vi "manual vs automated tracked data (real world coordinates).vi"() -> ()   [LabVIEW 2013]
panel:
  out "x/y 2":dbl
  out "x/y":dbl
  out "Waveform Graph 2":sgl[][](graph)
  out "Waveform Graph":sgl[][](graph)
  out "Y":sgl[](array[numeric])
  out "X":sgl[](array[numeric])
  out "Y 2":dbl[](array[numeric])
  out "X 2":dbl[](array[numeric])
  in  "auto top FangYang vs Ueda":T1[](array[typedef])=[{"X"=-379.219, "Y"=-1944.1919}, {"X"=240.74095, "Y"=358.58084}, {"X"=236.91107, "Y"=378.82852}, {"X"=238.72923, "Y"=457.2503}, {"X"=246.48058, "Y"=461.8201}, {"X"=265.79745, "Y"=446.8123}, {"X"=271.0491, "Y"=407.61075}, {"X"=277.55893, "Y"=412.3402}, {"X"=288.31927, "Y"=362.18567}, {"X"=298.93817, "Y"=356.80734}, {"X"=303.91098, "Y"=386.79193}, {"X"=329.3833, "Y"=355.87955}, {"X"=354.7859, "Y"=344.95035}, {"X"=363.8193, "Y"=354.83017}, {"X"=363.8193, "Y"=354.83017}, {"X"=414.12973, "Y"=388.4446}, {"X"=421.80878, "Y"=393.18253}, {"X"=440.06366, "Y"=451.29065}, {"X"=455.7114, "Y"=498.36505}, {"X"=464.16785, "Y"=553.61487}, {"X"=472.8004, "Y"=511.89783}, {"X"=458.46417, "Y"=469.90585}, {"X"=458.46417, "Y"=469.90585}, {"X"=447.3518, "Y"=460.67822}, {"X"=444.36072, "Y"=387.53275}, {"X"=437.37646, "Y"=367.7333}, {"X"=415.4438, "Y"=388.40497}, {"X"=397.8395, "Y"=403.80304}, {"X"=389.98856, "Y"=404.03882}, {"X"=361.21103, "Y"=404.90305}, {"X"=363.9455, "Y"=298.30313}, {"X"=396.3589, "Y"=408.77762}, {"X"=400.2796, "Y"=408.66003}, {"X"=419.1897, "Y"=189.43721}, {"X"=436.9622, "Y"=161.15974}, {"X"=445.31467, "Y"=160.89108}, {"X"=461.96823, "Y"=103.768394}, {"X"=460.7954, "Y"=69.094284}, {"X"=468.21814, "Y"=33.54667}, {"X"=467.0633, "Y"=57.186203}, {"X"=470.7626, "Y"=68.76565}, {"X"=470.15222, "Y"=109.23079}, {"X"=464.2563, "Y"=171.41397}, {"X"=456.3204, "Y"=221.01631}, {"X"=445.86578, "Y"=269.50647}, {"X"=438.85596, "Y"=275.0047}, {"X"=424.95166, "Y"=317.16812}, {"X"=423.05118, "Y"=363.13348}, {"X"=412.08105, "Y"=373.52164}, {"X"=396.9989, "Y"=500.07834}, {"X"=382.2929, "Y"=560.511}, {"X"=371.58298, "Y"=583.38385}, {"X"=350.8116, "Y"=458.73624}, {"X"=346.625, "Y"=473.19745}, {"X"=347.8018, "Y"=477.91788}, {"X"=349.33124, "Y"=410.1879}, {"X"=345.52036, "Y"=405.37427}, {"X"=346.936, "Y"=400.39108}, {"X"=340.89392, "Y"=375.6783}, {"X"=333.8183, "Y"=330.26135}, {"X"=326.2376, "Y"=304.67575}, {"X"=323.5547, "Y"=304.75873}, {"X"=322.37048, "Y"=294.37253}, {"X"=313.15634, "Y"=278.9214}, {"X"=295.73862, "Y"=263.60336}, {"X"=294.3835, "Y"=263.64578}, {"X"=297.13943, "Y"=258.24423}, {"X"=278.10477, "Y"=269.45547}, {"X"=241.50314, "Y"=254.66132}, {"X"=216.58736, "Y"=328.72873}, {"X"=210.20592, "Y"=349.36923}, {"X"=204.47275, "Y"=228.98254}, {"X"=197.85901, "Y"=324.16034}, {"X"=200.60747, "Y"=329.22}, {"X"=205.63214, "Y"=308.4058}, {"X"=215.69052, "Y"=364.3957}, {"X"=226.2489, "Y"=364.0744}, {"X"=218.27173, "Y"=359.26556}, {"X"=227.4764, "Y"=353.91983}, {"X"=237.96664, "Y"=338.3229}, {"X"=243.2823, "Y"=338.15997}, {"X"=225.9597, "Y"=333.5725}, {"X"=225.41745, "Y"=276.38568}, {"X"=232.00192, "Y"=254.9596}, {"X"=220.97665, "Y"=239.24193}, {"X"=207.9769, "Y"=185.16287}, {"X"=213.36469, "Y"=173.9132}, {"X"=189.40637, "Y"=72.21436}, {"X"=181.8577, "Y"=48.98817}, {"X"=183.73094, "Y"=72.40179}, {"X"=195.36647, "Y"=89.45416}, {"X"=199.78233, "Y"=100.85296}, {"X"=211.69986, "Y"=151.62987}, {"X"=221.6728, "Y"=173.64636}, {"X"=232.91647, "Y"=195.38316}, {"X"=238.62537, "Y"=227.90225}, {"X"=246.82507, "Y"=227.64288}, {"X"=259.14227, "Y"=243.40915}, {"X"=260.52017, "Y"=270.00504}, {"X"=257.81534, "Y"=270.08957}, {"X"=242.96771, "Y"=275.838}, {"X"=250.69382, "Y"=150.36983}, {"X"=255.08963, "Y"=259.56235}, {"X"=261.86682, "Y"=248.67987}, {"X"=272.69354, "Y"=269.6246}, {"X"=278.10477, "Y"=269.45547}, {"X"=282.1635, "Y"=269.32864}, {"X"=286.2226, "Y"=269.20178}, {"X"=272.70654, "Y"=264.32425}, {"X"=306.6389, "Y"=257.94647}, {"X"=303.5981, "Y"=289.72357}, {"X"=347.25598, "Y"=261.9909}, {"X"=294.258, "Y"=279.51022}, {"X"=364.34863, "Y"=282.58826}, {"X"=356.25198, "Y"=282.84018}, {"X"=356.25198, "Y"=282.84018}, {"X"=309.64783, "Y"=346.32993}, {"X"=304.28574, "Y"=351.5757}, {"X"=304.6125, "Y"=320.87338}, {"X"=304.3941, "Y"=341.39526}, {"X"=300.4082, "Y"=341.51727}, {"X"=303.11807, "Y"=336.32578}, {"X"=301.73682, "Y"=341.4766}, {"X"=293.36713, "Y"=392.0872}, {"X"=265.8795, "Y"=337.4673}, {"X"=229.95079, "Y"=333.44998}, {"X"=224.6294, "Y"=333.61334}, {"X"=221.08926, "Y"=249.96196}, {"X"=206.20949, "Y"=157.41422}, {"X"=199.17181, "Y"=152.03471}, {"X"=177.59418, "Y"=118.7725}, {"X"=162.02908, "Y"=55.53973}, {"X"=181.57751, "Y"=107.19645}, {"X"=187.20538, "Y"=107.01233}, {"X"=210.45204, "Y"=162.8691}, {"X"=229.01479, "Y"=222.7933}, {"X"=241.6175, "Y"=275.88016}, {"X"=265.98276, "Y"=199.81622}, {"X"=281.8607, "Y"=331.85638}, {"X"=309.83194, "Y"=330.9977}, {"X"=353.24872, "Y"=410.0704}, {"X"=369.1337, "Y"=448.57358}, {"X"=354.31934, "Y"=419.85693}, {"X"=388.86124, "Y"=476.71115}, {"X"=404.44525, "Y"=471.49573}, {"X"=397.5853, "Y"=447.73016}, {"X"=335.15945, "Y"=468.76834}, {"X"=399.13074, "Y"=476.40933}, {"X"=409.58768, "Y"=471.34436}, {"X"=442.19287, "Y"=460.83047}, {"X"=428.71732, "Y"=531.71704}, {"X"=435.66354, "Y"=545.30023}, {"X"=441.3716, "Y"=531.35144}, {"X"=441.08243, "Y"=563.3649}, {"X"=441.82288, "Y"=599.25073}, {"X"=441.82288, "Y"=599.25073}, {"X"=300.9056, "Y"=289.80722}, {"X"=303.27682, "Y"=320.91452}, {"X"=304.88873, "Y"=294.91483}, {"X"=302.14774, "Y"=300.21722}, {"X"=311.16425, "Y"=330.9568}, {"X"=325.41125, "Y"=356.0006}, {"X"=336.2913, "Y"=340.41895}, {"X"=345.92438, "Y"=324.75232}, {"X"=359.84485, "Y"=354.9513}, {"X"=373.0323, "Y"=261.1841}, {"X"=376.3531, "Y"=239.7184}, {"X"=397.72824, "Y"=212.01292}, {"X"=403.9889, "Y"=189.92242}, {"X"=421.00232, "Y"=178.3422}, {"X"=435.3338, "Y"=166.7844}, {"X"=443.82617, "Y"=194.148}, {"X"=405.97333, "Y"=211.75133}, {"X"=395.51877, "Y"=195.68765}, {"X"=382.29224, "Y"=223.35791}, {"X"=365.83505, "Y"=277.27997}, {"X"=359.91315, "Y"=298.428}, {"X"=351.9673, "Y"=293.45447}, {"X"=359.40192, "Y"=319.1864}, {"X"=374.11057, "Y"=318.73352}, {"X"=406.23087, "Y"=353.53772}, {"X"=431.4278, "Y"=352.76987}, {"X"=433.6227, "Y"=392.8267}, {"X"=457.67108, "Y"=460.37363}, {"X"=451.4063, "Y"=507.85492}, {"X"=448.51663, "Y"=489.16385}, {"X"=448.51663, "Y"=489.16385}, {"X"=425.93756, "Y"=508.59604}, {"X"=418.19464, "Y"=480.59506}, {"X"=391.5912, "Y"=471.87402}, {"X"=392.87646, "Y"=471.8362}, {"X"=374.60245, "Y"=481.8744}, {"X"=358.30508, "Y"=468.08615}, {"X"=332.6767, "Y"=464.06296}, {"X"=310.7989, "Y"=464.7087}, {"X"=300.5541, "Y"=460.22177}, {"X"=268.79126, "Y"=160.98972}, {"X"=301.7822, "Y"=198.67523}, {"X"=274.39758, "Y"=143.9781}, {"X"=243.649, "Y"=133.67818}, {"X"=223.9627, "Y"=122.96163}, {"X"=206.67265, "Y"=89.082535}, {"X"=209.72241, "Y"=106.27566}, {"X"=213.87715, "Y"=100.39111}, {"X"=224.33687, "Y"=162.4218}, {"X"=244.06622, "Y"=222.31648}, {"X"=246.91164, "Y"=249.15009}, {"X"=248.3299, "Y"=265.08722}, {"X"=240.20668, "Y"=265.34146}, {"X"=222.39363, "Y"=244.5663}, {"X"=217.94925, "Y"=212.27502}, {"X"=216.70294, "Y"=223.18333}, {"X"=220.28804, "Y"=173.69084}, {"X"=208.69188, "Y"=134.81302}, {"X"=206.98508, "Y"=112.09752}, {"X"=199.60603, "Y"=89.31481}, {"X"=199.33972, "Y"=71.88633}, {"X"=200.75891, "Y"=71.83946}, {"X"=199.5175, "Y"=83.52155}, {"X"=197.51016, "Y"=135.17603}, {"X"=206.36482, "Y"=168.57701}, {"X"=205.60648, "Y"=212.66722}, {"X"=200.03648, "Y"=207.38855}, {"X"=192.34073, "Y"=314.00165}, {"X"=187.25673, "Y"=395.2878}, {"X"=175.81679, "Y"=410.47076}, {"X"=170.72452, "Y"=468.84314}, {"X"=160.84576, "Y"=483.4124}, {"X"=164.80504, "Y"=488.03143}, {"X"=126.20091, "Y"=549.63324}, {"X"=122.39982, "Y"=581.50006}, {"X"=113.91068, "Y"=617.37}, {"X"=111.26169, "Y"=613.0294}, {"X"=309.1677, "Y"=273.77222}, {"X"=309.5259, "Y"=356.48468}, {"X"=317.46802, "Y"=356.24268}, {"X"=314.82053, "Y"=356.32333}, {"X"=302.96057, "Y"=351.61618}, {"X"=302.96057, "Y"=351.61618}, {"X"=296.3351, "Y"=351.81836}, {"X"=263.21674, "Y"=392.9966}, {"X"=242.17143, "Y"=378.66916}, {"X"=246.204, "Y"=398.4716}, {"X"=228.1136, "Y"=423.63065}, {"X"=201.92369, "Y"=491.66708}, {"X"=293.8873, "Y"=326.35217}, {"X"=200.47363, "Y"=556.62933}, {"X"=222.29388, "Y"=486.34427}, {"X"=233.27432, "Y"=418.57858}, {"X"=250.01248, "Y"=363.3513}, {"X"=264.5458, "Y"=347.7084}, {"X"=267.19788, "Y"=347.62735}, {"X"=289.39935, "Y"=397.1706}, {"X"=297.43478, "Y"=376.99493}, {"X"=312.10898, "Y"=361.46176}, {"X"=332.48547, "Y"=330.30225}, {"X"=346.03375, "Y"=319.59802}, {"X"=346.5849, "Y"=293.62143}, {"X"=371.967, "Y"=250.56561}, {"X"=379.76813, "Y"=308.2136}, {"X"=402.4357, "Y"=348.58032}, {"X"=411.69434, "Y"=383.5361}, {"X"=419.88736, "Y"=408.07205}, {"X"=429.587, "Y"=238.04216}, {"X"=426.85587, "Y"=238.12817}, {"X"=414.32574, "Y"=383.4566}, {"X"=407.9354, "Y"=378.65494}, {"X"=399.2458, "Y"=363.85678}, {"X"=392.97385, "Y"=353.9417}, {"X"=385.34088, "Y"=344.01648}, {"X"=376.34485, "Y"=287.46362}, {"X"=374.99683, "Y"=287.5055}, {"X"=367.3255, "Y"=271.95737}, {"X"=366.10992, "Y"=266.7051}, {"X"=344.87204, "Y"=246.07013}, {"X"=328.3579, "Y"=257.26566}, {"X"=300.6056, "Y"=320.99677}, {"X"=273.95816, "Y"=301.09036}, {"X"=261.89386, "Y"=347.78946}, {"X"=229.19672, "Y"=398.98386}, {"X"=222.28929, "Y"=364.1949}, {"X"=221.96889, "Y"=333.695}, {"X"=217.18909, "Y"=379.426}, {"X"=224.97849, "Y"=369.1518}, {"X"=236.80927, "Y"=363.75305}, {"X"=257.9162, "Y"=347.91104}, {"X"=281.96057, "Y"=311.23404}, {"X"=295.3917, "Y"=305.62973}, {"X"=304.94443, "Y"=289.68173}, {"X"=306.34842, "Y"=284.3928}, {"X"=340.3712, "Y"=267.5095}, {"X"=347.3689, "Y"=256.66974}, {"X"=357.3827, "Y"=234.94028}, {"X"=360.42987, "Y"=277.4484}, {"X"=369.24594, "Y"=250.65103}, {"X"=385.66235, "Y"=333.79547}, {"X"=417.4444, "Y"=337.93494}, {"X"=413.45056, "Y"=338.0572}, {"X"=428.72202, "Y"=291.07355}, {"X"=409.45697, "Y"=338.17944}, {"X"=394.12802, "Y"=358.966}, {"X"=386.3465, "Y"=354.14368}, {"X"=376.3368, "Y"=334.08133}, {"X"=359.14832, "Y"=329.48373}, {"X"=339.45166, "Y"=314.63647}, {"X"=323.71545, "Y"=294.3308}, {"X"=310.393, "Y"=284.26697}, {"X"=300.9056, "Y"=289.80722}, {"X"=287.60858, "Y"=263.85782}, {"X"=287.64157, "Y"=258.54196}, {"X"=264.582, "Y"=259.2648}, {"X"=252.32089, "Y"=238.25346}, {"X"=234.67851, "Y"=249.5347}, {"X"=218.60973, "Y"=271.31485}, {"X"=176.73038, "Y"=272.62366}, {"X"=169.85439, "Y"=267.54343}, {"X"=161.87743, "Y"=273.08786}, {"X"=305.05627, "Y"=279.17377}, {"X"=303.54422, "Y"=294.95654}, {"X"=313.22327, "Y"=273.64566}, {"X"=320.11566, "Y"=356.162}, {"X"=337.2312, "Y"=360.69733}, {"X"=358.14706, "Y"=370.13712}, {"X"=349.7784, "Y"=390.38565}, {"X"=326.65207, "Y"=361.01923}, {"X"=293.64502, "Y"=356.96863}, {"X"=303.9795, "Y"=252.69997}, {"X"=271.46576, "Y"=210.57452}, {"X"=257.67438, "Y"=161.34784}, {"X"=228.31302, "Y"=139.8306}, {"X"=206.67265, "Y"=89.082535}, {"X"=200.93274, "Y"=83.47496}, {"X"=215.8117, "Y"=145.87416}, {"X"=205.89624, "Y"=134.90378}, {"X"=217.51859, "Y"=173.77979}, {"X"=223.00299, "Y"=168.04184}, {"X"=224.54747, "Y"=184.63231}, {"X"=235.85585, "Y"=222.57658}, {"X"=241.50314, "Y"=254.66132}, {"X"=248.5037, "Y"=312.26724}, {"X"=244.4902, "Y"=312.39117}, {"X"=240.3876, "Y"=296.91562}, {"X"=240.2975, "Y"=281.1916}, {"X"=235.01584, "Y"=297.08224}, {"X"=202.55582, "Y"=282.36755}, {"X"=176.81717, "Y"=213.58202}, {"X"=188.58812, "Y"=256.3225}, {"X"=180.3701, "Y"=186.04678}, {"X"=180.96799, "Y"=147.00183}, {"X"=177.71228, "Y"=124.46775}, {"X"=164.87761, "Y"=55.445217}, {"X"=160.02571, "Y"=31.936}, {"X"=169.54489, "Y"=72.87026}, {"X"=178.41144, "Y"=90.01146}, {"X"=194.80911, "Y"=140.91658}, {"X"=209.06375, "Y"=162.91382}, {"X"=218.84299, "Y"=168.17564}, {"X"=228.83044, "Y"=201.00035}, {"X"=239.9919, "Y"=227.85902}, {"X"=255.0473, "Y"=238.1675}, {"X"=261.87262, "Y"=269.96277}, {"X"=260.51038, "Y"=254.06462}, {"X"=270.03537, "Y"=243.06615}, {"X"=283.65466, "Y"=242.6373}, {"X"=295.8706, "Y"=247.61078}, {"X"=305.56696, "Y"=231.18684}, {"X"=310.6467, "Y"=263.13675}, {"X"=372.19714, "Y"=339.31992}, {"X"=410.2086, "Y"=353.4165}, {"X"=403.69467, "Y"=457.1731}, {"X"=407.02423, "Y"=504.47195}, {"X"=409.40213, "Y"=476.10745}, {"X"=406.8435, "Y"=509.1516}, {"X"=405.7687, "Y"=536.985}, {"X"=404.5055, "Y"=537.0214}, {"X"=398.35855, "Y"=532.59424}, {"X"=398.52753, "Y"=527.9733}, {"X"=395.66397, "Y"=537.2765}, {"X"=381.03802, "Y"=560.54694}, {"X"=347.79678, "Y"=534.0551}, {"X"=323.13248, "Y"=497.53937}, {"X"=293.8394, "Y"=493.69034}, {"X"=265.7652, "Y"=489.79614}, {"X"=250.43665, "Y"=490.24536}, {"X"=245.33957, "Y"=200.47417}, {"X"=118.084724, "Y"=-153.04642}, {"X"=187.93501, "Y"=146.77635}, {"X"=173.50957, "Y"=124.60461}, {"X"=200.81985, "Y"=168.75537}, {"X"=189.63121, "Y"=163.53984}, {"X"=199.95107, "Y"=201.92079}, {"X"=207.12892, "Y"=223.48662}, {"X"=216.70294, "Y"=223.18333}, {"X"=251.02194, "Y"=259.68985}, {"X"=271.15475, "Y"=357.654}, {"X"=286.8732, "Y"=382.31723}, {"X"=290.31995, "Y"=450.90988}, {"X"=285.35538, "Y"=417.019}, {"X"=299.80493, "Y"=535.4418}, {"X"=303.0285, "Y"=469.71536}, {"X"=304.6303, "Y"=440.82095}, {"X"=316.1484, "Y"=450.14423}, {"X"=321.84073, "Y"=415.92648}, {"X"=300.60196, "Y"=455.41882}, {"X"=307.33325, "Y"=431.02618}, {"X"=310.17142, "Y"=411.3622}, {"X"=320.8349, "Y"=396.2238}, {"X"=332.21237, "Y"=345.6403}, {"X"=330.8784, "Y"=420.55783}, {"X"=347.69815, "Y"=424.94507}, {"X"=341.93652, "Y"=256.84}, {"X"=348.63104, "Y"=197.18207}, {"X"=367.4061, "Y"=163.39705}, {"X"=393.15042, "Y"=140.13481}, {"X"=399.95477, "Y"=145.54662}, {"X"=432.32553, "Y"=104.73669}, {"X"=438.21426, "Y"=98.800285}, {"X"=422.44806, "Y"=105.05933}, {"X"=399.95477, "Y"=145.54662}, {"X"=382.86548, "Y"=157.31483}, {"X"=374.20538, "Y"=168.7476}, {"X"=364.89804, "Y"=207.60568}, {"X"=356.017, "Y"=234.98335}, {"X"=357.12906, "Y"=245.68477}, {"X"=362.17767, "Y"=261.52386}, {"X"=376.34485, "Y"=287.46362}, {"X"=403.31186, "Y"=286.62585}, {"X"=404.66055, "Y"=286.58395}, {"X"=412.35614, "Y"=296.80368}, {"X"=416.63788, "Y"=358.28104}, {"X"=404.53503, "Y"=363.69608}, {"X"=396.80368, "Y"=433.2259}, {"X"=390.8023, "Y"=418.76605}, {"X"=388.01697, "Y"=384.25134}, {"X"=382.05923, "Y"=364.379}, {"X"=368.62222, "Y"=324.05447}, {"X"=360.86798, "Y"=313.97607}, {"X"=358.56912, "Y"=298.46964}, {"X"=348.38382, "Y"=272.54846}, {"X"=344.7622, "Y"=251.41966}, {"X"=359.9835, "Y"=240.23386}, {"X"=376.65897, "Y"=228.94151}, {"X"=373.6245, "Y"=239.80432}, {"X"=357.3197, "Y"=118.61896}, {"X"=362.44385, "Y"=250.86458}, {"X"=360.821, "Y"=261.5663}, {"X"=354.0381, "Y"=261.77863}, {"X"=341.50626, "Y"=345.35623}, {"X"=332.03146, "Y"=355.79886}, {"X"=331.9691, "Y"=283.59567}, {"X"=322.37048, "Y"=294.37253}, {"X"=323.87708, "Y"=283.84744}, {"X"=328.74655, "Y"=314.96658}, {"X"=322.0569, "Y"=315.17285}, {"X"=332.76074, "Y"=314.8428}, {"X"=371.3333, "Y"=223.70456}, {"X"=385.69534, "Y"=201.48022}, {"X"=411.3019, "Y"=178.65279}, {"X"=439.07886, "Y"=144.28235}, {"X"=451.1975, "Y"=92.61483}, {"X"=466.7766, "Y"=63.05458}, {"X"=475.5642, "Y"=86.03841}, {"X"=479.00424, "Y"=74.32069}, {"X"=467.62756, "Y"=74.69521}, {"X"=461.96823, "Y"=103.768394}, {"X"=431.8558, "Y"=116.19174}, {"X"=397.63095, "Y"=173.55046}, {"X"=363.11554, "Y"=223.9645}, {"X"=331.4402, "Y"=235.75839}, {"X"=302.19974, "Y"=294.99823}, {"X"=274.0315, "Y"=274.86865}, {"X"=245.69124, "Y"=281.0235}, {"X"=236.21696, "Y"=276.04868}, {"X"=201.98804, "Y"=245.20883}, {"X"=206.22096, "Y"=255.76895}, {"X"=204.9421, "Y"=261.13428}, {"X"=208.01904, "Y"=287.45206}, {"X"=221.96889, "Y"=333.695}, {"X"=237.56705, "Y"=276.00656}, {"X"=263.223, "Y"=301.42285}, {"X"=291.29462, "Y"=316.12143}, {"X"=328.65985, "Y"=320.13297}, {"X"=362.49445, "Y"=354.87054}, {"X"=384.2289, "Y"=379.37207}, {"X"=367.65726, "Y"=359.77148}, {"X"=401.1082, "Y"=348.62085}, {"X"=396.25394, "Y"=374.00113}, {"X"=386.38184, "Y"=394.24954}, {"X"=367.3848, "Y"=369.85684}, {"X"=345.38187, "Y"=350.32153}, {"X"=328.83347, "Y"=309.78653}, {"X"=317.97086, "Y"=320.46207}, {"X"=303.5981, "Y"=289.72357}, {"X"=286.44205, "Y"=231.79086}, {"X"=274.16602, "Y"=226.77806}, {"X"=253.64651, "Y"=222.01299}, {"X"=238.62537, "Y"=227.90225}, {"X"=221.08926, "Y"=249.96196}, {"X"=210.29085, "Y"=255.64119}, {"X"=193.92058, "Y"=250.81616}, {"X"=191.3005, "Y"=256.23737}, {"X"=155.12737, "Y"=273.2988}, {"X"=164.96967, "Y"=288.7914}, {"X"=203.26804, "Y"=239.80038}, {"X"=212.1883, "Y"=190.54393}, {"X"=198.34164, "Y"=271.94827}, {"X"=208.23715, "Y"=303.12598}, {"X"=208.23715, "Y"=303.12598}, {"X"=298.88113, "Y"=215.14905}, {"X"=301.15927, "Y"=263.4337}, {"X"=303.70636, "Y"=279.21582}, {"X"=304.1243, "Y"=366.747}, {"X"=315.16135, "Y"=330.8341}, {"X"=328.00946, "Y"=278.45856}, {"X"=327.75055, "Y"=294.20566}, {"X"=327.2389, "Y"=325.32678}, {"X"=334.5714, "Y"=288.76135}, {"X"=340.2679, "Y"=272.8017}, {"X"=351.0894, "Y"=272.46402}, {"X"=352.08554, "Y"=288.21725}, {"X"=386.3465, "Y"=354.14368}, {"X"=414.32574, "Y"=383.4566}, {"X"=426.63568, "Y"=402.93823}, {"X"=418.67697, "Y"=373.3218}, {"X"=414.65796, "Y"=408.22885}, {"X"=395.2224, "Y"=403.88162}, {"X"=392.6054, "Y"=403.96024}, {"X"=367.88538, "Y"=399.76102}, {"X"=365.2663, "Y"=399.83978}, {"X"=357.40973, "Y"=400.07608}, {"X"=356.1004, "Y"=400.11545}, {"X"=349.08444, "Y"=477.8802}, {"X"=341.68768, "Y"=463.797}, {"X"=353.73636, "Y"=444.2017}, {"X"=365.51648, "Y"=439.01086}, {"X"=380.17352, "Y"=467.44162}, {"X"=386.32892, "Y"=514.4104}, {"X"=457.86722, "Y"=431.4079}, {"X"=484.4065, "Y"=-57.935837}, {"X"=442.9617, "Y"=417.20642}, {"X"=412.45734, "Y"=527.5703}, {"X"=397.76608, "Y"=514.0781}, {"X"=382.66696, "Y"=509.8551}, {"X"=375.16956, "Y"=462.80875}, {"X"=367.88538, "Y"=399.76102}, {"X"=332.62775, "Y"=395.8686}, {"X"=323.45532, "Y"=396.14487}, {"X"=302.5465, "Y"=391.8103}, {"X"=296.03244, "Y"=387.0299}, {"X"=286.81134, "Y"=392.28494}, {"X"=286.81134, "Y"=392.28494}, {"X"=400.17252, "Y"=447.65347}, {"X"=399.2077, "Y"=509.3738}, {"X"=403.02548, "Y"=509.26273}, {"X"=405.19016, "Y"=485.7102}, {"X"=403.02548, "Y"=509.26273}, {"X"=396.90216, "Y"=466.94855}, {"X"=394.44757, "Y"=500.1528}, {"X"=391.42844, "Y"=476.6357}, {"X"=386.60703, "Y"=467.25198}, {"X"=386.60703, "Y"=467.25198}, {"X"=375.7407, "Y"=528.6326}, {"X"=377.27362, "Y"=560.65485}, {"X"=391.75436, "Y"=467.10028}, {"X"=359.71393, "Y"=463.26492}, {"X"=335.34302, "Y"=459.19345}, {"X"=335.34302, "Y"=459.19345}, {"X"=361.00174, "Y"=463.22693}, {"X"=363.57742, "Y"=463.1509}, {"X"=406.55682, "Y"=195.33585}, {"X"=418.8694, "Y"=161.7417}, {"X"=427.36685, "Y"=87.62015}, {"X"=427.5587, "Y"=46.72962}, {"X"=432.80966, "Y"=22.828001}, {"X"=433.52322, "Y"=40.624928}, {"X"=429.9314, "Y"=22.924105}, {"X"=423.71936, "Y"=35.027763}, {"X"=402.69833, "Y"=105.70447}, {"X"=400.40546, "Y"=173.46149}, {"X"=397.3642, "Y"=222.88116}, {"X"=399.36795, "Y"=244.35674}, {"X"=419.91556, "Y"=275.59488}, {"X"=422.62094, "Y"=275.51056}, {"X"=421.35406, "Y"=306.92935}, {"X"=418.98203, "Y"=398.22427}, {"X"=390.63828, "Y"=423.66296}, {"X"=395.90833, "Y"=384.01294}, {"X"=380.73743, "Y"=364.41916}, {"X"=362.3646, "Y"=359.93253}, {"X"=337.32822, "Y"=355.63745}, {"X"=333.35562, "Y"=355.7585}, {"X"=330.70737, "Y"=355.8392}, {"X"=326.73523, "Y"=355.96027}, {"X"=301.38425, "Y"=376.87527}, {"X"=301.6354, "Y"=351.65662}, {"X"=298.9852, "Y"=351.7375}, {"X"=298.9852, "Y"=351.7375}, {"X"=328.31293, "Y"=175.77328}, {"X"=342.16974, "Y"=175.32893}, {"X"=363.3731, "Y"=157.94276}, {"X"=380.4029, "Y"=146.1784}, {"X"=412.9895, "Y"=93.8668}, {"X"=427.05325, "Y"=23.020203}, {"X"=445.9059, "Y"=52.011703}, {"X"=430.90436, "Y"=70.07986}, {"X"=436.11108, "Y"=81.54107}, {"X"=436.11108, "Y"=81.54107}, {"X"=442.61676, "Y"=127.21894}, {"X"=444.85556, "Y"=232.18176}, {"X"=447.96188, "Y"=253.51651}, {"X"=446.4858, "Y"=285.2846}, {"X"=441.34085, "Y"=367.613}, {"X"=451.66818, "Y"=372.32233}, {"X"=455.37817, "Y"=377.21973}, {"X"=457.47787, "Y"=488.9016}, {"X"=450.0969, "Y"=558.5684}, {"X"=438.5471, "Y"=456.1429}, {"X"=428.2476, "Y"=485.0345}, {"X"=432.30676, "Y"=451.52026}, {"X"=422.70807, "Y"=403.05618}, {"X"=417.07404, "Y"=413.07477}, {"X"=395.90833, "Y"=384.01294}, {"X"=386.5079, "Y"=349.06644}, {"X"=377.971, "Y"=323.76706}, {"X"=369.04123, "Y"=308.54486}, {"X"=360.0418, "Y"=293.20398}, {"X"=349.27603, "Y"=293.53793}, {"X"=348.38382, "Y"=272.54846}, {"X"=343.2946, "Y"=256.79742}, {"X"=342.97308, "Y"=272.7173}, {"X"=328.83347, "Y"=309.78653}, {"X"=320.41577, "Y"=335.79553}, {"X"=314.82053, "Y"=356.32333}, {"X"=309.70905, "Y"=341.23257}, {"X"=310.0175, "Y"=315.5441}, {"X"=313.6956, "Y"=341.11057}, {"X"=316.14426, "Y"=356.28302}, {"X"=330.2622, "Y"=304.55127}, {"X"=328.65985, "Y"=320.13297}, {"X"=333.35562, "Y"=355.7585}, {"X"=330.70737, "Y"=355.8392}, {"X"=384.21347, "Y"=250.18115}, {"X"=349.07306, "Y"=240.57741}, {"X"=350.31927, "Y"=245.89886}, {"X"=324.5323, "Y"=241.35014}, {"X"=373.77353, "Y"=234.42339}, {"X"=373.77353, "Y"=234.42339}] {"Y" format="%.2f"; "X" format="%.2f"}
  in  "manual top FangYang vs Ueda":T1[](array[typedef])=[{"X"=239.20204, "Y"=322.8874}, {"X"=235.19978, "Y"=323.01062}, {"X"=230.03725, "Y"=343.67123}, {"X"=239.44966, "Y"=363.67273}, {"X"=246.204, "Y"=398.4716}, {"X"=251.4529, "Y"=403.26276}, {"X"=261.89664, "Y"=357.93613}, {"X"=275.09128, "Y"=367.62915}, {"X"=280.4372, "Y"=352.30356}, {"X"=284.5524, "Y"=326.63916}, {"X"=312.7584, "Y"=310.28296}, {"X"=342.86652, "Y"=277.99564}, {"X"=370.953, "Y"=287.6311}, {"X"=382.5318, "Y"=260.88678}, {"X"=387.81464, "Y"=307.9651}, {"X"=402.80164, "Y"=338.38315}, {"X"=417.96228, "Y"=358.24075}, {"X"=442.4209, "Y"=456.0284}, {"X"=454.60397, "Y"=470.01947}, {"X"=450.98236, "Y"=465.3546}, {"X"=449.82892, "Y"=436.50436}, {"X"=437.07224, "Y"=432.027}, {"X"=433.61102, "Y"=422.37988}, {"X"=428.82626, "Y"=412.72284}, {"X"=416.55896, "Y"=393.34064}, {"X"=399.2458, "Y"=363.85678}, {"X"=396.14706, "Y"=338.58682}, {"X"=374.11057, "Y"=318.73352}, {"X"=370.52417, "Y"=303.3061}, {"X"=378.4604, "Y"=261.01422}, {"X"=392.2322, "Y"=212.1873}, {"X"=400.9716, "Y"=156.73154}, {"X"=415.1122, "Y"=150.6741}, {"X"=431.14822, "Y"=99.03146}, {"X"=444.27118, "Y"=121.48421}, {"X"=457.94797, "Y"=69.18817}, {"X"=467.07086, "Y"=27.642868}, {"X"=467.9282, "Y"=39.481594}, {"X"=488.00742, "Y"=38.81433}, {"X"=489.5957, "Y"=62.30101}, {"X"=481.6519, "Y"=50.827534}, {"X"=474.2033, "Y"=56.950043}, {"X"=455.6411, "Y"=57.563995}, {"X"=445.17215, "Y"=132.80139}, {"X"=435.54196, "Y"=194.41203}, {"X"=435.25616, "Y"=264.54413}, {"X"=411.2074, "Y"=291.61685}, {"X"=379.46008, "Y"=318.56882}, {"X"=371.91138, "Y"=349.5119}, {"X"=379.82373, "Y"=394.44708}, {"X"=360.58163, "Y"=429.43857}, {"X"=362.39056, "Y"=409.79626}, {"X"=356.46255, "Y"=385.2045}, {"X"=351.82843, "Y"=415.0285}, {"X"=360.91373, "Y"=365.02148}, {"X"=361.556, "Y"=339.64563}, {"X"=348.1457, "Y"=345.1533}, {"X"=348.3694, "Y"=334.93866}, {"X"=332.94547, "Y"=304.4683}, {"X"=325.39175, "Y"=273.26593}, {"X"=318.63116, "Y"=273.4769}, {"X"=316.13992, "Y"=257.64865}, {"X"=318.92975, "Y"=252.23064}, {"X"=320.21228, "Y"=257.521}, {"X"=309.47787, "Y"=247.18295}, {"X"=304.03458, "Y"=247.3541}, {"X"=289.0682, "Y"=247.82465}, {"X"=257.80157, "Y"=259.47733}, {"X"=234.82944, "Y"=270.80792}, {"X"=224.47781, "Y"=318.1818}, {"X"=209.71854, "Y"=313.465}, {"X"=206.67325, "Y"=287.49393}, {"X"=208.45354, "Y"=318.6759}, {"X"=203.03413, "Y"=313.67142}, {"X"=210.84918, "Y"=297.8319}, {"X"=214.74847, "Y"=287.24268}, {"X"=217.44046, "Y"=287.15894}, {"X"=228.02405, "Y"=265.72278}, {"X"=246.95456, "Y"=259.81735}, {"X"=251.10126, "Y"=286.11166}, {"X"=249.71925, "Y"=275.62732}, {"X"=253.69653, "Y"=243.58063}, {"X"=246.89008, "Y"=243.79495}, {"X"=226.02925, "Y"=195.60301}, {"X"=211.69986, "Y"=151.62987}, {"X"=205.33966, "Y"=94.906654}, {"X"=199.16093, "Y"=60.185703}, {"X"=201.83557, "Y"=48.324272}, {"X"=189.90411, "Y"=18.999298}, {"X"=189.80031, "Y"=13.007771}, {"X"=198.98116, "Y"=48.41913}, {"X"=202.43257, "Y"=89.22191}, {"X"=215.41914, "Y"=111.822014}, {"X"=228.45569, "Y"=156.69646}, {"X"=235.5224, "Y"=173.20157}, {"X"=246.5597, "Y"=161.7059}, {"X"=254.97212, "Y"=200.16716}, {"X"=265.9705, "Y"=216.1932}, {"X"=268.66595, "Y"=248.46611}, {"X"=270.03537, "Y"=243.06615}, {"X"=261.8712, "Y"=264.6634}, {"X"=260.51364, "Y"=259.3923}, {"X"=261.86972, "Y"=259.3498}, {"X"=270.03537, "Y"=243.06615}, {"X"=279.56854, "Y"=242.76596}, {"X"=276.88205, "Y"=232.0928}, {"X"=276.8446, "Y"=242.85175}, {"X"=280.88235, "Y"=253.42508}, {"X"=288.9635, "Y"=263.8154}, {"X"=284.98718, "Y"=247.95296}, {"X"=298.54404, "Y"=252.8706}, {"X"=300.00217, "Y"=242.12256}, {"X"=322.84717, "Y"=262.75488}, {"X"=351.20712, "Y"=267.17087}, {"X"=374.55194, "Y"=303.18152}, {"X"=324.97818, "Y"=299.51007}, {"X"=312.7584, "Y"=310.28296}, {"X"=304.88873, "Y"=294.91483}, {"X"=307.57788, "Y"=294.8314}, {"X"=298.2132, "Y"=289.89084}, {"X"=286.2537, "Y"=263.90024}, {"X"=271.3745, "Y"=253.72356}, {"X"=283.40732, "Y"=290.3508}, {"X"=274.00204, "Y"=285.39917}, {"X"=276.77036, "Y"=264.19705}, {"X"=267.31775, "Y"=237.78053}, {"X"=232.75221, "Y"=173.29054}, {"X"=215.74673, "Y"=140.23792}, {"X"=197.05548, "Y"=106.69007}, {"X"=181.12276, "Y"=84.12712}, {"X"=173.80034, "Y"=72.72973}, {"X"=174.84859, "Y"=55.114388}, {"X"=185.04059, "Y"=66.51422}, {"X"=198.10231, "Y"=83.56814}, {"X"=225.36484, "Y"=122.91598}, {"X"=229.80086, "Y"=151.04497}, {"X"=240.02283, "Y"=233.25694}, {"X"=249.63046, "Y"=249.06459}, {"X"=278.0243, "Y"=290.51804}, {"X"=322.52853, "Y"=283.8894}, {"X"=353.22137, "Y"=355.15314}, {"X"=369.3323, "Y"=394.76306}, {"X"=385.43167, "Y"=423.81842}, {"X"=396.97522, "Y"=428.35352}, {"X"=394.32822, "Y"=467.0244}, {"X"=385.78766, "Y"=452.89725}, {"X"=389.82434, "Y"=447.96024}, {"X"=394.2067, "Y"=433.3032}, {"X"=401.2898, "Y"=452.4384}, {"X"=424.5509, "Y"=451.74982}, {"X"=437.4779, "Y"=451.3672}, {"X"=441.6659, "Y"=498.77493}, {"X"=453.95383, "Y"=507.7808}, {"X"=454.57773, "Y"=544.75604}, {"X"=450.42508, "Y"=576.64655}, {"X"=292.8288, "Y"=290.05814}, {"X"=291.4072, "Y"=300.5499}, {"X"=288.85962, "Y"=279.67844}, {"X"=291.5207, "Y"=284.85413}, {"X"=295.56424, "Y"=284.7283}, {"X"=303.8152, "Y"=268.65198}, {"X"=324.44962, "Y"=246.71223}, {"X"=341.51572, "Y"=278.03772}, {"X"=348.15652, "Y"=283.09204}, {"X"=361.47995, "Y"=234.81107}, {"X"=364.62234, "Y"=218.49739}, {"X"=382.7011, "Y"=162.90508}, {"X"=401.60315, "Y"=178.96332}, {"X"=428.12524, "Y"=139.0029}, {"X"=432.79208, "Y"=127.53789}, {"X"=439.80954, "Y"=127.310074}, {"X"=432.55756, "Y"=133.21027}, {"X"=411.13034, "Y"=145.18549}, {"X"=398.37158, "Y"=151.21423}, {"X"=381.7242, "Y"=196.12732}, {"X"=342.25513, "Y"=240.79208}, {"X"=350.20212, "Y"=251.24889}, {"X"=340.3712, "Y"=267.5095}, {"X"=355.14798, "Y"=272.33737}, {"X"=377.54062, "Y"=292.6612}, {"X"=399.16617, "Y"=328.25522}, {"X"=423.46967, "Y"=353.0124}, {"X"=440.5809, "Y"=412.37085}, {"X"=441.19894, "Y"=427.03497}, {"X"=445.46802, "Y"=446.31076}, {"X"=447.5864, "Y"=455.87573}, {"X"=434.03534, "Y"=441.81793}, {"X"=434.91373, "Y"=422.34097}, {"X"=419.28314, "Y"=422.80768}, {"X"=394.42258, "Y"=389.03903}, {"X"=376.1881, "Y"=339.19775}, {"X"=366.87634, "Y"=339.48276}, {"X"=370.5846, "Y"=349.55237}, {"X"=368.25726, "Y"=287.71487}, {"X"=349.3053, "Y"=229.80544}, {"X"=337.20065, "Y"=219.36607}, {"X"=326.92743, "Y"=175.81772}, {"X"=299.57486, "Y"=137.52074}, {"X"=278.825, "Y"=80.910706}, {"X"=232.07677, "Y"=82.449684}, {"X"=220.80858, "Y"=88.6179}, {"X"=210.84033, "Y"=83.148796}, {"X"=216.3724, "Y"=71.323845}, {"X"=223.691, "Y"=94.3044}, {"X"=238.08875, "Y"=139.51372}, {"X"=245.09705, "Y"=144.92638}, {"X"=248.09155, "Y"=200.38646}, {"X"=250.89282, "Y"=216.67159}, {"X"=248.15187, "Y"=216.75854}, {"X"=246.71555, "Y"=200.43031}, {"X"=229.80086, "Y"=151.04497}, {"X"=218.539, "Y"=140.1474}, {"X"=205.57951, "Y"=112.143425}, {"X"=216.50261, "Y"=82.962395}, {"X"=206.2772, "Y"=59.949963}, {"X"=194.01985, "Y"=6.85391}, {"X"=198.98116, "Y"=48.41913}, {"X"=201.92157, "Y"=54.21612}, {"X"=206.19743, "Y"=54.07425}, {"X"=223.691, "Y"=94.3044}, {"X"=225.52028, "Y"=139.92111}, {"X"=214.6833, "Y"=168.30945}, {"X"=210.73833, "Y"=185.07445}, {"X"=202.47536, "Y"=277.1016}, {"X"=176.7875, "Y"=395.60358}, {"X"=172.86205, "Y"=395.722}, {"X"=164.08694, "Y"=410.82303}, {"X"=134.96031, "Y"=474.66898}, {"X"=131.66402, "Y"=526.44995}, {"X"=119.037506, "Y"=494.09613}, {"X"=113.462845, "Y"=545.4187}, {"X"=109.466774, "Y"=599.76953}, {"X"=317.13464, "Y"=284.05722}, {"X"=322.29178, "Y"=299.5933}, {"X"=322.37048, "Y"=294.37253}, {"X"=307.8159, "Y"=273.8144}, {"X"=313.15634, "Y"=278.9214}, {"X"=300.9056, "Y"=289.80722}, {"X"=269.90463, "Y"=316.781}, {"X"=269.95078, "Y"=290.76886}, {"X"=263.223, "Y"=301.42285}, {"X"=231.1978, "Y"=323.13382}, {"X"=205.3592, "Y"=379.7844}, {"X"=200.09319, "Y"=458.39398}, {"X"=194.00696, "Y"=477.68924}, {"X"=190.3484, "Y"=487.2818}, {"X"=205.5351, "Y"=477.34998}, {"X"=206.74506, "Y"=472.5532}, {"X"=219.51836, "Y"=467.40295}, {"X"=239.72214, "Y"=408.55157}, {"X"=260.58963, "Y"=383.11234}, {"X"=298.93817, "Y"=356.80734}, {"X"=306.0049, "Y"=315.66782}, {"X"=316.6349, "Y"=320.5032}, {"X"=322.21326, "Y"=304.8002}, {"X"=342.97308, "Y"=272.7173}, {"X"=365.97232, "Y"=271.9996}, {"X"=377.872, "Y"=234.29413}, {"X"=381.81067, "Y"=239.54655}, {"X"=394.5717, "Y"=265.8156}, {"X"=409.87863, "Y"=254.71028}, {"X"=415.78433, "Y"=312.28268}, {"X"=410.98233, "Y"=333.01932}, {"X"=417.4444, "Y"=337.93494}, {"X"=413.45056, "Y"=338.0572}, {"X"=411.53455, "Y"=353.3761}, {"X"=410.4243, "Y"=312.44797}, {"X"=397.0264, "Y"=312.8611}, {"X"=386.1092, "Y"=276.64825}, {"X"=371.38525, "Y"=271.8307}, {"X"=375.89737, "Y"=255.77547}, {"X"=379.8175, "Y"=260.97174}, {"X"=366.66412, "Y"=245.38498}, {"X"=363.25095, "Y"=218.54083}, {"X"=357.12906, "Y"=245.68477}, {"X"=327.3451, "Y"=235.88753}, {"X"=282.4234, "Y"=215.6712}, {"X"=247.03975, "Y"=280.9815}, {"X"=227.1017, "Y"=312.92816}, {"X"=208.88121, "Y"=349.40973}, {"X"=200.52539, "Y"=324.07825}, {"X"=207.33832, "Y"=334.14417}, {"X"=214.3075, "Y"=359.38635}, {"X"=227.29002, "Y"=333.53168}, {"X"=245.828, "Y"=312.34988}, {"X"=274.00204, "Y"=285.39917}, {"X"=290.20917, "Y"=279.63638}, {"X"=303.8152, "Y"=268.65198}, {"X"=312.06784, "Y"=257.77628}, {"X"=324.44962, "Y"=246.71223}, {"X"=353.2857, "Y"=235.06947}, {"X"=357.51, "Y"=229.54631}, {"X"=354.528, "Y"=240.40564}, {"X"=355.76703, "Y"=245.72758}, {"X"=377.25623, "Y"=255.73286}, {"X"=393.7403, "Y"=249.88208}, {"X"=408.32034, "Y"=296.92868}, {"X"=409.66556, "Y"=296.88702}, {"X"=411.568, "Y"=317.5802}, {"X"=410.2298, "Y"=317.6214}, {"X"=393.00766, "Y"=312.98502}, {"X"=389.4904, "Y"=297.5119}, {"X"=384.11157, "Y"=297.6785}, {"X"=350.62164, "Y"=293.4962}, {"X"=325.22568, "Y"=283.80548}, {"X"=310.77457, "Y"=252.48665}, {"X"=313.3577, "Y"=263.05188}, {"X"=297.27725, "Y"=242.20836}, {"X"=290.5397, "Y"=231.66145}, {"X"=283.6269, "Y"=247.99573}, {"X"=267.2944, "Y"=259.17975}, {"X"=248.21169, "Y"=232.9983}, {"X"=219.37984, "Y"=217.6714}, {"X"=192.27815, "Y"=234.76488}, {"X"=176.03485, "Y"=240.6592}, {"X"=143.37236, "Y"=241.68924}, {"X"=290.13678, "Y"=290.14175}, {"X"=298.0269, "Y"=310.73788}, {"X"=292.90836, "Y"=279.55228}, {"X"=302.4617, "Y"=268.69427}, {"X"=321.10266, "Y"=289.17978}, {"X"=346.9191, "Y"=277.86935}, {"X"=360.1708, "Y"=287.96606}, {"X"=351.84933, "Y"=298.6778}, {"X"=359.33545, "Y"=266.91684}, {"X"=335.63342, "Y"=230.23724}, {"X"=295.11438, "Y"=171.2877}, {"X"=266.02444, "Y"=144.24908}, {"X"=243.46063, "Y"=93.6556}, {"X"=222.16544, "Y"=82.77597}, {"X"=205.0978, "Y"=77.52516}, {"X"=207.6228, "Y"=54.02696}, {"X"=210.84033, "Y"=83.148796}, {"X"=220.86732, "Y"=94.39707}, {"X"=226.91663, "Y"=139.87585}, {"X"=233.97882, "Y"=150.90996}, {"X"=238.29272, "Y"=173.1126}, {"X"=242.56001, "Y"=195.07533}, {"X"=245.41104, "Y"=216.8455}, {"X"=256.43686, "Y"=254.1925}, {"X"=252.36363, "Y"=254.32037}, {"X"=249.68388, "Y"=265.04483}, {"X"=248.34941, "Y"=270.3854}, {"X"=209.72043, "Y"=212.5365}, {"X"=189.15364, "Y"=213.19002}, {"X"=181.41675, "Y"=169.37947}, {"X"=182.36133, "Y"=146.95674}, {"X"=178.17488, "Y"=78.412865}, {"X"=175.34163, "Y"=78.50628}, {"X"=173.17143, "Y"=43.36698}, {"X"=171.87143, "Y"=49.32003}, {"X"=171.61406, "Y"=37.492336}, {"X"=177.4572, "Y"=43.224335}, {"X"=185.04059, "Y"=66.51422}, {"X"=201.01929, "Y"=89.26836}, {"X"=215.55072, "Y"=123.235565}, {"X"=227.0157, "Y"=151.13496}, {"X"=236.90755, "Y"=173.15709}, {"X"=239.74142, "Y"=184.14583}, {"X"=255.03665, "Y"=232.78275}, {"X"=264.59296, "Y"=232.48093}, {"X"=274.13583, "Y"=237.56552}, {"X"=283.68253, "Y"=237.26447}, {"X"=285.13602, "Y"=221.01544}, {"X"=301.67697, "Y"=209.61456}, {"X"=308.4837, "Y"=214.84439}, {"X"=311.293, "Y"=209.309}, {"X"=430.9709, "Y"=301.4366}, {"X"=421.2309, "Y"=342.91956}, {"X"=413.9342, "Y"=393.4197}, {"X"=414.0739, "Y"=422.9632}, {"X"=397.41385, "Y"=452.5531}, {"X"=399.4008, "Y"=433.14856}, {"X"=409.2406, "Y"=413.30933}, {"X"=409.42905, "Y"=408.38565}, {"X"=408.4969, "Y"=398.5396}, {"X"=382.75665, "Y"=384.41022}, {"X"=377.49686, "Y"=384.56912}, {"X"=367.24908, "Y"=374.87985}, {"X"=351.61435, "Y"=309.083}, {"X"=346.8074, "Y"=283.134}, {"X"=324.20294, "Y"=262.71243}, {"X"=287.9426, "Y"=210.05096}, {"X"=263.23178, "Y"=172.31165}, {"X"=245.07243, "Y"=139.28735}, {"X"=210.08975, "Y"=134.76764}, {"X"=179.82416, "Y"=89.96503}, {"X"=180.40004, "Y"=118.680984}, {"X"=181.80301, "Y"=118.63523}, {"X"=195.92763, "Y"=123.87458}, {"X"=206.51932, "Y"=179.67885}, {"X"=227.59892, "Y"=217.41063}, {"X"=238.59251, "Y"=222.48988}, {"X"=255.07909, "Y"=254.23512}, {"X"=280.73935, "Y"=285.18954}, {"X"=287.18747, "Y"=331.69287}, {"X"=293.5253, "Y"=372.09772}, {"X"=296.03244, "Y"=387.0299}, {"X"=296.3351, "Y"=351.81836}, {"X"=294.39368, "Y"=426.53662}, {"X"=296.03244, "Y"=387.0299}, {"X"=289.6755, "Y"=357.0896}, {"X"=301.4843, "Y"=366.8272}, {"X"=295.05206, "Y"=346.77603}, {"X"=298.89124, "Y"=361.86395}, {"X"=301.8899, "Y"=326.10614}, {"X"=320.49127, "Y"=330.67047}, {"X"=318.1892, "Y"=304.92468}, {"X"=322.92737, "Y"=257.43588}, {"X"=323.2503, "Y"=236.01666}, {"X"=337.10043, "Y"=224.78738}, {"X"=354.7634, "Y"=107.27028}, {"X"=375.59305, "Y"=118.0239}, {"X"=402.89285, "Y"=99.95587}, {"X"=412.9895, "Y"=93.8668}, {"X"=421.69928, "Y"=87.80615}, {"X"=424.7589, "Y"=81.91421}, {"X"=421.8352, "Y"=46.91952}, {"X"=396.20218, "Y"=88.642914}, {"X"=386.28976, "Y"=88.96822}, {"X"=368.71072, "Y"=112.539276}, {"X"=361.44037, "Y"=180.24925}, {"X"=352.16034, "Y"=224.31102}, {"X"=358.7484, "Y"=234.8972}, {"X"=374.8383, "Y"=245.12798}, {"X"=380.28842, "Y"=244.95662}, {"X"=396.92502, "Y"=276.31122}, {"X"=409.2776, "Y"=307.30228}, {"X"=408.50772, "Y"=327.96844}, {"X"=406.23087, "Y"=353.53772}, {"X"=406.4046, "Y"=312.57193}, {"X"=404.53503, "Y"=363.69608}, {"X"=395.9726, "Y"=343.69153}, {"X"=385.82373, "Y"=328.66483}, {"X"=372.3009, "Y"=287.58923}, {"X"=361.7811, "Y"=277.40628}, {"X"=354.528, "Y"=240.40564}, {"X"=356.50092, "Y"=272.29514}, {"X"=346.45807, "Y"=235.28479}, {"X"=343.72726, "Y"=235.37091}, {"X"=350.67267, "Y"=229.76225}, {"X"=352.04007, "Y"=229.71906}, {"X"=359.26718, "Y"=213.23318}, {"X"=367.50662, "Y"=212.97177}, {"X"=365.7159, "Y"=229.28714}, {"X"=361.2153, "Y"=245.55629}, {"X"=358.49112, "Y"=245.64194}, {"X"=347.7094, "Y"=240.62035}, {"X"=327.0002, "Y"=257.3082}, {"X"=315.20224, "Y"=225.48004}, {"X"=315.9979, "Y"=268.27124}, {"X"=314.71323, "Y"=263.00946}, {"X"=321.5698, "Y"=257.47842}, {"X"=336.9008, "Y"=235.58618}, {"X"=353.38123, "Y"=169.4164}, {"X"=391.5746, "Y"=145.81741}, {"X"=407.33127, "Y"=94.0522}, {"X"=424.81992, "Y"=116.42086}, {"X"=444.6267, "Y"=81.26116}, {"X"=467.62756, "Y"=74.69521}, {"X"=475.63144, "Y"=56.90281}, {"X"=482.15582, "Y"=68.38999}, {"X"=482.89117, "Y"=27.115475}, {"X"=468.4912, "Y"=57.138973}, {"X"=439.19592, "Y"=75.6312}, {"X"=427.1376, "Y"=93.403206}, {"X"=397.71783, "Y"=128.67653}, {"X"=347.94574, "Y"=164.023}, {"X"=340.57178, "Y"=186.43959}, {"X"=279.6133, "Y"=232.00655}, {"X"=264.60855, "Y"=194.37154}, {"X"=248.17186, "Y"=222.18642}, {"X"=222.17453, "Y"=223.01}, {"X"=204.47275, "Y"=228.98254}, {"X"=198.83734, "Y"=218.32315}, {"X"=205.76134, "Y"=223.52995}, {"X"=218.43153, "Y"=255.38562}, {"X"=232.12582, "Y"=270.89243}, {"X"=234.86691, "Y"=276.09082}, {"X"=251.03789, "Y"=265.00244}, {"X"=292.90836, "Y"=279.55228}, {"X"=337.26553, "Y"=288.67764}, {"X"=370.09872, "Y"=318.85706}, {"X"=378.27472, "Y"=313.43933}, {"X"=397.3017, "Y"=343.6509}, {"X"=401.1082, "Y"=348.62085}, {"X"=395.1631, "Y"=328.3781}, {"X"=385.66235, "Y"=333.79547}, {"X"=351.49734, "Y"=314.26505}, {"X"=328.92065, "Y"=304.59277}, {"X"=324.03958, "Y"=273.30814}, {"X"=310.77457, "Y"=252.48665}, {"X"=300.25284, "Y"=215.10553}, {"X"=285.2869, "Y"=193.71147}, {"X"=285.13602, "Y"=221.01544}, {"X"=261.85052, "Y"=188.95625}, {"X"=254.97212, "Y"=200.16716}, {"X"=227.40663, "Y"=195.55904}, {"X"=200.03648, "Y"=207.38855}, {"X"=183.99109, "Y"=229.6304}, {"X"=158.19951, "Y"=235.84119}, {"X"=154.54918, "Y"=252.05402}, {"X"=166.50633, "Y"=240.95969}, {"X"=169.10243, "Y"=235.49684}, {"X"=187.02863, "Y"=245.67987}, {"X"=198.92392, "Y"=223.74655}, {"X"=207.65163, "Y"=261.04935}, {"X"=288.5866, "Y"=321.36682}, {"X"=292.59265, "Y"=321.24347}, {"X"=288.62042, "Y"=316.2039}, {"X"=296.64337, "Y"=315.9565}, {"X"=298.26007, "Y"=284.64444}, {"X"=317.4244, "Y"=262.9246}, {"X"=327.83664, "Y"=288.97058}, {"X"=333.59976, "Y"=267.72113}, {"X"=330.89142, "Y"=267.80576}, {"X"=337.76242, "Y"=262.28806}, {"X"=352.92227, "Y"=251.1635}, {"X"=363.66913, "Y"=256.15878}, {"X"=379.66135, "Y"=266.2816}, {"X"=396.92502, "Y"=276.31122}, {"X"=412.90622, "Y"=317.539}, {"X"=422.56058, "Y"=342.8789}, {"X"=421.2309, "Y"=342.91956}, {"X"=417.85086, "Y"=327.6816}, {"X"=391.98547, "Y"=343.8134}, {"X"=382.52667, "Y"=349.18793}, {"X"=366.49667, "Y"=303.43063}, {"X"=346.69598, "Y"=288.38467}, {"X"=320.9486, "Y"=299.6349}, {"X"=325.14294, "Y"=289.05426}, {"X"=315.43726, "Y"=310.20023}, {"X"=308.8009, "Y"=305.21503}, {"X"=325.5748, "Y"=345.84314}, {"X"=345.94833, "Y"=385.5221}, {"X"=368.51352, "Y"=424.32355}, {"X"=396.73245, "Y"=471.72272}, {"X"=389.18063, "Y"=467.17615}, {"X"=399.8947, "Y"=490.58673}, {"X"=399.30328, "Y"=471.64706}, {"X"=386.13828, "Y"=481.53583}, {"X"=394.2067, "Y"=433.3032}, {"X"=384.65097, "Y"=448.1136}, {"X"=370.2898, "Y"=453.35602}, {"X"=354.43683, "Y"=414.9504}, {"X"=347.59152, "Y"=370.45737}, {"X"=327.07013, "Y"=335.59155}, {"X"=317.5393, "Y"=351.17123}, {"X"=304.66745, "Y"=315.70908}, {"X"=287.12396, "Y"=341.9239}, {"X"=414.0452, "Y"=322.65796}, {"X"=417.55872, "Y"=368.33456}, {"X"=415.57202, "Y"=418.0254}, {"X"=409.6027, "Y"=437.70023}, {"X"=400.52332, "Y"=437.97015}, {"X"=399.57565, "Y"=428.27597}, {"X"=391.13165, "Y"=408.93436}, {"X"=388.01697, "Y"=384.25134}, {"X"=368.06863, "Y"=344.54437}, {"X"=357.5661, "Y"=339.76773}, {"X"=338.01434, "Y"=319.84494}, {"X"=340.07748, "Y"=350.48343}, {"X"=353.33942, "Y"=350.07867}, {"X"=355.51312, "Y"=314.1412}, {"X"=351.84933, "Y"=298.6778}, {"X"=364.21164, "Y"=234.72493}, {"X"=381.96304, "Y"=140.49687}, {"X"=384.4248, "Y"=151.66422}, {"X"=400.90436, "Y"=117.19965}, {"X"=409.15338, "Y"=82.42715}, {"X"=431.61383, "Y"=52.48516}, {"X"=437.12735, "Y"=22.683838}, {"X"=433.53534, "Y"=4.8309765}, {"X"=423.87723, "Y"=-6.91128}, {"X"=434.0063, "Y"=28.745121}, {"X"=433.77863, "Y"=-1.2022539}, {"X"=414.74915, "Y"=5.4612136}, {"X"=393.91827, "Y"=71.29936}, {"X"=392.82605, "Y"=106.02695}, {"X"=392.6142, "Y"=157.00078}, {"X"=397.08078, "Y"=190.14294}, {"X"=400.36182, "Y"=255.00859}, {"X"=395.57294, "Y"=276.35336}, {"X"=393.8288, "Y"=328.41907}, {"X"=387.83505, "Y"=349.0259}, {"X"=392.97385, "Y"=353.9417}, {"X"=383.5382, "Y"=359.28824}, {"X"=369.53668, "Y"=339.40134}, {"X"=359.40192, "Y"=319.1864}, {"X"=351.7317, "Y"=303.8873}, {"X"=345.23938, "Y"=293.66315}, {"X"=321.41327, "Y"=268.102}, {"X"=314.3013, "Y"=294.62283}, {"X"=317.06268, "Y"=289.30527}, {"X"=309.4155, "Y"=252.52931}, {"X"=311.49033, "Y"=192.87505}, {"X"=327.54526, "Y"=136.6141}, {"X"=335.33984, "Y"=169.99582}, {"X"=348.41418, "Y"=141.58264}, {"X"=383.1225, "Y"=100.60268}, {"X"=402.8436, "Y"=59.310295}, {"X"=417.32538, "Y"=52.9585}, {"X"=432.3293, "Y"=34.741188}, {"X"=453.59024, "Y"=39.95807}, {"X"=455.56796, "Y"=28.026333}, {"X"=448.76474, "Y"=51.916996}, {"X"=450.56686, "Y"=75.25686}, {"X"=445.53543, "Y"=92.80036}, {"X"=443.7704, "Y"=132.84682}, {"X"=441.30725, "Y"=188.7312}, {"X"=433.0048, "Y"=221.75381}, {"X"=429.4065, "Y"=306.68066}, {"X"=432.53262, "Y"=357.7974}, {"X"=427.27164, "Y"=388.04822}, {"X"=434.05023, "Y"=412.5664}, {"X"=426.5931, "Y"=373.082}, {"X"=431.4382, "Y"=412.64462}, {"X"=428.37177, "Y"=392.98486}, {"X"=426.84714, "Y"=397.9877}, {"X"=423.74524, "Y"=378.17667}, {"X"=412.11932, "Y"=338.09793}, {"X"=393.8288, "Y"=328.41907}, {"X"=376.19437, "Y"=292.70294}, {"X"=368.6787, "Y"=271.91513}, {"X"=372.4464, "Y"=282.33633}, {"X"=368.6787, "Y"=271.91513}, {"X"=355.64255, "Y"=251.0781}, {"X"=346.23383, "Y"=246.02731}, {"X"=340.68262, "Y"=251.54773}, {"X"=324.44962, "Y"=246.71223}, {"X"=314.5752, "Y"=273.60345}, {"X"=310.07965, "Y"=310.36566}, {"X"=306.93622, "Y"=351.49484}, {"X"=297.7511, "Y"=341.5986}, {"X"=297.88846, "Y"=326.22916}, {"X"=301.9926, "Y"=315.79156}, {"X"=315.8566, "Y"=278.83725}, {"X"=329.35995, "Y"=278.41647}, {"X"=334.85794, "Y"=272.97052}, {"X"=340.68262, "Y"=251.54773}, {"X"=335.63342, "Y"=230.23724}, {"X"=340.89163, "Y"=240.83502}, {"X"=381.08176, "Y"=217.97597}, {"X"=396.5351, "Y"=206.60042}, {"X"=403.9889, "Y"=189.92242}, {"X"=402.4173, "Y"=195.46779}, {"X"=-379.219, "Y"=-1944.1919}] {"Y" format="%.2f"; "X" format="%.2f"}
  in  "auto bottom FangYang vs Ueda":T1[](array[typedef])=[{"X"=-379.219, "Y"=-1944.1919}, {"X"=317.43216, "Y"=1053.8207}, {"X"=317.49054, "Y"=1050.41}, {"X"=317.43216, "Y"=1053.8207}, {"X"=311.58713, "Y"=1080.9746}, {"X"=309.33588, "Y"=1087.7101}, {"X"=313.90225, "Y"=1070.8431}, {"X"=323.50958, "Y"=1019.24695}, {"X"=334.87592, "Y"=1001.4716}, {"X"=354.02655, "Y"=947.34045}, {"X"=386.00964, "Y"=931.91864}, {"X"=424.87033, "Y"=897.5589}, {"X"=417.93372, "Y"=875.1119}, {"X"=368.66806, "Y"=910.1948}, {"X"=368.66806, "Y"=910.1948}, {"X"=394.78656, "Y"=909.5272}, {"X"=402.11484, "Y"=924.15295}, {"X"=393.6163, "Y"=939.0497}, {"X"=364.13254, "Y"=983.05554}, {"X"=366.33206, "Y"=1018.1932}, {"X"=365.123, "Y"=1021.7003}, {"X"=365.123, "Y"=1021.7003}, {"X"=368.22855, "Y"=993.592}, {"X"=379.46252, "Y"=957.5743}, {"X"=391.91815, "Y"=953.6435}, {"X"=399.0943, "Y"=942.56116}, {"X"=436.46927, "Y"=893.511}, {"X"=438.20255, "Y"=882.16473}, {"X"=431.334, "Y"=904.86804}, {"X"=404.85126, "Y"=912.9857}, {"X"=425.50708, "Y"=930.91675}, {"X"=387.59222, "Y"=978.9086}, {"X"=384.96686, "Y"=989.6375}, {"X"=372.923, "Y"=1018.031}, {"X"=362.39078, "Y"=1039.0417}, {"X"=355.14923, "Y"=1063.0914}, {"X"=349.45752, "Y"=1073.3512}, {"X"=341.65085, "Y"=1083.5963}, {"X"=340.98856, "Y"=1110.1201}, {"X"=342.05533, "Y"=1110.0947}, {"X"=357.95953, "Y"=1112.9989}, {"X"=366.27075, "Y"=1119.3464}, {"X"=377.734, "Y"=1125.5931}, {"X"=388.48526, "Y"=1122.0826}, {"X"=390.6117, "Y"=1122.0322}, {"X"=386.48837, "Y"=1118.8671}, {"X"=378.21664, "Y"=1112.5173}, {"X"=362.5376, "Y"=1103.0209}, {"X"=365.9632, "Y"=1096.3248}, {"X"=297.37637, "Y"=1101.2738}, {"X"=306.54126, "Y"=1133.7643}, {"X"=307.14096, "Y"=1091.0928}, {"X"=312.71637, "Y"=1077.5961}, {"X"=314.11032, "Y"=1123.8441}, {"X"=309.61893, "Y"=1140.152}, {"X"=307.55307, "Y"=1136.9739}, {"X"=305.38947, "Y"=1215.7245}, {"X"=295.84958, "Y"=1240.287}, {"X"=297.13528, "Y"=1305.2252}, {"X"=297.068, "Y"=1310.9933}, {"X"=293.07706, "Y"=1311.0812}, {"X"=291.165, "Y"=1302.4653}, {"X"=288.98395, "Y"=1322.636}, {"X"=286.76315, "Y"=1350.9562}, {"X"=286.7863, "Y"=1348.1533}, {"X"=275.12143, "Y"=1311.4768}, {"X"=272.20215, "Y"=1288.3424}, {"X"=262.15225, "Y"=1294.3995}, {"X"=262.14096, "Y"=1253.0728}, {"X"=256.96518, "Y"=1207.6039}, {"X"=257.94162, "Y"=1173.256}, {"X"=257.91043, "Y"=1154.2036}, {"X"=261.0532, "Y"=1138.07}, {"X"=255.6882, "Y"=1102.2697}, {"X"=238.17624, "Y"=1048.9259}, {"X"=245.70853, "Y"=1035.0114}, {"X"=235.8871, "Y"=1035.2518}, {"X"=175.00629, "Y"=962.7145}, {"X"=165.87134, "Y"=955.7153}, {"X"=158.47481, "Y"=934.02374}, {"X"=158.82188, "Y"=944.9903}, {"X"=162.5189, "Y"=955.7998}, {"X"=169.43042, "Y"=962.8546}, {"X"=183.33957, "Y"=984.0048}, {"X"=199.34192, "Y"=1008.3379}, {"X"=210.51334, "Y"=1018.54736}, {"X"=221.96846, "Y"=1056.1407}, {"X"=235.24364, "Y"=1086.1538}, {"X"=244.96594, "Y"=1095.9045}, {"X"=247.10716, "Y"=1095.8533}, {"X"=244.92784, "Y"=1089.2562}, {"X"=236.48578, "Y"=1106.0283}, {"X"=226.9968, "Y"=1116.1119}, {"X"=210.14957, "Y"=1126.3064}, {"X"=203.905, "Y"=1187.0785}, {"X"=195.5931, "Y"=1187.2709}, {"X"=177.58412, "Y"=1175.125}, {"X"=177.58412, "Y"=1175.125}, {"X"=173.33037, "Y"=1275.867}, {"X"=171.13054, "Y"=1270.0055}, {"X"=180.90848, "Y"=1257.893}, {"X"=186.84438, "Y"=1251.7764}, {"X"=195.66212, "Y"=1190.3944}, {"X"=205.63031, "Y"=1168.1509}, {"X"=216.8946, "Y"=1151.967}, {"X"=239.88142, "Y"=1132.0991}, {"X"=254.66339, "Y"=1118.727}, {"X"=264.24527, "Y"=1082.1139}, {"X"=278.22852, "Y"=1081.7773}, {"X"=292.46585, "Y"=1054.4275}, {"X"=299.28894, "Y"=1026.7861}, {"X"=306.9053, "Y"=1030.0598}, {"X"=315.20477, "Y"=1057.2767}, {"X"=328.74234, "Y"=1083.9065}, {"X"=328.74234, "Y"=1083.9065}, {"X"=220.92953, "Y"=1059.5651}, {"X"=220.92953, "Y"=1059.5651}, {"X"=224.89444, "Y"=1028.6123}, {"X"=227.87157, "Y"=1000.6026}, {"X"=229.04831, "Y"=1007.6032}, {"X"=225.62517, "Y"=997.132}, {"X"=224.47919, "Y"=993.6266}, {"X"=235.50273, "Y"=989.81055}, {"X"=245.52074, "Y"=1000.16504}, {"X"=245.55861, "Y"=1007.1949}, {"X"=262.0804, "Y"=1031.1587}, {"X"=259.93384, "Y"=1072.1467}, {"X"=248.00401, "Y"=1058.9078}, {"X"=248.11508, "Y"=1082.502}, {"X"=251.41423, "Y"=1102.3718}, {"X"=253.58083, "Y"=1112.2004}, {"X"=251.43852, "Y"=1108.965}, {"X"=251.43852, "Y"=1108.965}, {"X"=214.08228, "Y"=1106.5627}, {"X"=199.21866, "Y"=1110.2094}, {"X"=186.1953, "Y"=1100.6243}, {"X"=167.06949, "Y"=1104.3866}, {"X"=154.61108, "Y"=1114.5559}, {"X"=152.97029, "Y"=1098.1075}, {"X"=170.17238, "Y"=1101.0076}, {"X"=192.60574, "Y"=1100.471}, {"X"=227.87617, "Y"=1099.6274}, {"X"=262.10156, "Y"=1108.7108}, {"X"=273.8447, "Y"=1105.137}, {"X"=304.5114, "Y"=1127.3252}, {"X"=312.19302, "Y"=1110.8054}, {"X"=318.59076, "Y"=1110.6532}, {"X"=313.3653, "Y"=1104.1941}, {"X"=374.1852, "Y"=1106.04}, {"X"=308.07062, "Y"=1101.0184}, {"X"=337.9461, "Y"=1103.6077}, {"X"=330.03958, "Y"=1123.4669}, {"X"=325.7256, "Y"=1126.8234}, {"X"=323.60382, "Y"=1126.8735}, {"X"=314.0568, "Y"=1127.0994}, {"X"=307.55307, "Y"=1136.9739}, {"X"=390.63345, "Y"=1041.7854}, {"X"=391.04657, "Y"=1031.4528}, {"X"=397.0964, "Y"=1017.43616}, {"X"=400.4864, "Y"=989.2518}, {"X"=406.17334, "Y"=960.51294}, {"X"=404.85126, "Y"=912.9857}, {"X"=398.19485, "Y"=964.3152}, {"X"=396.40134, "Y"=953.53064}, {"X"=363.80133, "Y"=993.70184}, {"X"=389.40057, "Y"=989.5273}, {"X"=380.48615, "Y"=1021.32275}, {"X"=373.5425, "Y"=1031.8813}, {"X"=363.37402, "Y"=1042.4503}, {"X"=356.9139, "Y"=1076.5311}, {"X"=357.8914, "Y"=1079.8604}, {"X"=364.35544, "Y"=1079.7048}, {"X"=368.44113, "Y"=1086.2913}, {"X"=378.60922, "Y"=1072.648}, {"X"=377.79416, "Y"=1035.2251}, {"X"=388.56662, "Y"=982.44666}, {"X"=383.88058, "Y"=1075.8815}, {"X"=380.7692, "Y"=1072.5958}, {"X"=377.4414, "Y"=1014.4345}, {"X"=365.11508, "Y"=1056.0652}, {"X"=348.01596, "Y"=1086.7816}, {"X"=352.12637, "Y"=1093.3385}, {"X"=349.98117, "Y"=1093.3899}, {"X"=355.2467, "Y"=1096.5812}, {"X"=355.2467, "Y"=1096.5812}, {"X"=354.17517, "Y"=1096.6068}, {"X"=374.88528, "Y"=1055.828}, {"X"=392.4431, "Y"=996.52234}, {"X"=395.90652, "Y"=992.90485}, {"X"=397.6018, "Y"=978.65894}, {"X"=391.77585, "Y"=957.2647}, {"X"=375.48044, "Y"=910.0207}, {"X"=338.98715, "Y"=918.37244}, {"X"=329.85562, "Y"=922.30206}, {"X"=324.06586, "Y"=929.81793}, {"X"=345.25888, "Y"=983.5259}, {"X"=305.31195, "Y"=984.5213}, {"X"=303.8005, "Y"=1016.2489}, {"X"=293.71576, "Y"=1037.2811}, {"X"=280.54816, "Y"=1051.309}, {"X"=273.8908, "Y"=1091.89}, {"X"=270.63345, "Y"=1108.5076}, {"X"=259.97192, "Y"=1112.0483}, {"X"=242.86725, "Y"=1102.5759}, {"X"=234.56107, "Y"=1128.9799}, {"X"=229.23006, "Y"=1125.8545}, {"X"=219.64369, "Y"=1122.8235}, {"X"=212.00273, "Y"=1109.9047}, {"X"=215.04802, "Y"=1099.9342}, {"X"=219.50714, "Y"=1113.0114}, {"X"=227.9869, "Y"=1109.5238}, {"X"=239.73592, "Y"=1112.5299}, {"X"=254.63722, "Y"=1108.8887}, {"X"=262.10156, "Y"=1108.7108}, {"X"=267.42914, "Y"=1111.8708}, {"X"=272.74603, "Y"=1115.0245}, {"X"=274.88733, "Y"=1111.6934}, {"X"=257.8415, "Y"=1112.099}, {"X"=235.50548, "Y"=1115.9097}, {"X"=209.64755, "Y"=1096.7504}, {"X"=165.7979, "Y"=1097.8003}, {"X"=125.99809, "Y"=1141.253}, {"X"=94.56652, "Y"=1145.2146}, {"X"=78.01701, "Y"=1132.6831}, {"X"=71.93826, "Y"=1119.7979}, {"X"=94.03958, "Y"=1135.5449}, {"X"=126.11102, "Y"=1095.4331}, {"X"=116.03825, "Y"=1108.902}, {"X"=144.42017, "Y"=1098.3123}, {"X"=232.4427, "Y"=1129.03}, {"X"=248.1778, "Y"=1095.8276}, {"X"=269.60187, "Y"=1091.9928}, {"X"=287.80573, "Y"=1094.8788}, {"X"=216.4497, "Y"=1049.4552}, {"X"=223.13757, "Y"=1062.9033}, {"X"=219.3811, "Y"=1025.2822}, {"X"=213.64305, "Y"=1007.9842}, {"X"=213.42786, "Y"=993.90125}, {"X"=227.87157, "Y"=1000.6026}, {"X"=235.50273, "Y"=989.81055}, {"X"=232.04779, "Y"=975.6513}, {"X"=248.70644, "Y"=971.6532}, {"X"=253.14786, "Y"=967.9525}, {"X"=252.09328, "Y"=985.8474}, {"X"=249.93388, "Y"=1000.0556}, {"X"=251.03722, "Y"=1000.02826}, {"X"=254.31917, "Y"=989.3423}, {"X"=275.3703, "Y"=985.2674}, {"X"=274.11514, "Y"=1027.404}, {"X"=309.34305, "Y"=1012.62164}, {"X"=310.72488, "Y"=1136.8992}, {"X"=306.49582, "Y"=1136.9989}, {"X"=321.6222, "Y"=1174.9293}, {"X"=345.22577, "Y"=1190.0593}, {"X"=370.97424, "Y"=1253.6117}, {"X"=391.95245, "Y"=1285.6796}, {"X"=401.47684, "Y"=1297.1262}, {"X"=397.59592, "Y"=1294.3063}, {"X"=387.03903, "Y"=1282.8601}, {"X"=373.25366, "Y"=1274.3469}, {"X"=370.43484, "Y"=1268.5006}, {"X"=364.04752, "Y"=1217.4493}, {"X"=357.7015, "Y"=1189.7712}, {"X"=354.7662, "Y"=1148.7332}, {"X"=348.00232, "Y"=1164.8314}, {"X"=343.29117, "Y"=1103.4801}, {"X"=340.74307, "Y"=1119.9518}, {"X"=357.36417, "Y"=1132.5651}, {"X"=367.73914, "Y"=1138.7838}, {"X"=390.5978, "Y"=1173.3269}, {"X"=417.88095, "Y"=1191.5}, {"X"=449.33923, "Y"=1236.8092}, {"X"=458.4028, "Y"=1254.632}, {"X"=466.14484, "Y"=1260.4194}, {"X"=448.96368, "Y"=1242.8508}, {"X"=434.82242, "Y"=1240.1573}, {"X"=415.28033, "Y"=1222.396}, {"X"=400.54175, "Y"=1207.3944}, {"X"=378.50058, "Y"=1189.2909}, {"X"=356.19556, "Y"=1170.9707}, {"X"=335.57574, "Y"=1158.7659}, {"X"=314.63092, "Y"=1156.0684}, {"X"=295.34027, "Y"=1091.3757}, {"X"=293.0358, "Y"=1107.9738}, {"X"=307.5996, "Y"=1133.7394}, {"X"=315.62714, "Y"=1159.232}, {"X"=342.10724, "Y"=1190.1313}, {"X"=366.232, "Y"=1183.321}, {"X"=392.13712, "Y"=1210.6669}, {"X"=418.29443, "Y"=1243.5441}, {"X"=429.20297, "Y"=1249.3052}, {"X"=439.8924, "Y"=1258.0315}, {"X"=431.07437, "Y"=1252.2579}, {"X"=414.61743, "Y"=1255.6171}, {"X"=403.10715, "Y"=1240.8751}, {"X"=393.0377, "Y"=1213.7197}, {"X"=405.4047, "Y"=1191.7877}, {"X"=379.45624, "Y"=1164.0981}, {"X"=360.33868, "Y"=1138.958}, {"X"=349.58774, "Y"=1145.6469}, {"X"=334.96704, "Y"=1093.7494}, {"X"=320.78433, "Y"=1107.3125}, {"X"=298.83377, "Y"=1159.6245}, {"X"=269.4574, "Y"=1160.311}, {"X"=247.62549, "Y"=1198.5342}, {"X"=231.18791, "Y"=1211.2772}, {"X"=197.37207, "Y"=1221.2572}, {"X"=177.94211, "Y"=1224.7563}, {"X"=163.3621, "Y"=1249.3068}, {"X"=153.62811, "Y"=1261.4889}, {"X"=149.80202, "Y"=1267.52}, {"X"=156.774, "Y"=1264.3938}, {"X"=172.063, "Y"=1234.0188}, {"X"=177.00327, "Y"=1227.8269}, {"X"=178.02148, "Y"=1190.8022}, {"X"=176.45218, "Y"=1171.9945}, {"X"=175.45996, "Y"=1136.8577}, {"X"=396.80643, "Y"=1024.3925}, {"X"=392.8412, "Y"=1014.0551}, {"X"=394.226, "Y"=1007.0267}, {"X"=394.6554, "Y"=996.46747}, {"X"=394.79913, "Y"=992.9324}, {"X"=373.64227, "Y"=996.98846}, {"X"=348.21576, "Y"=997.61884}, {"X"=344.8109, "Y"=1001.2256}, {"X"=347.3876, "Y"=1029.0674}, {"X"=326.52716, "Y"=1033.0325}, {"X"=315.03763, "Y"=1067.4427}, {"X"=298.70975, "Y"=1077.9335}, {"X"=281.5348, "Y"=1068.253}, {"X"=268.5297, "Y"=1092.0186}, {"X"=258.8853, "Y"=1095.5713}, {"X"=247.24, "Y"=1122.1691}, {"X"=231.38356, "Y"=1129.055}, {"X"=201.67142, "Y"=1126.5072}, {"X"=181.58812, "Y"=1168.7113}, {"X"=167.8421, "Y"=1197.267}, {"X"=142.50998, "Y"=1185.3696}, {"X"=128.172, "Y"=1213.6392}, {"X"=121.63982, "Y"=1271.1151}, {"X"=114.15748, "Y"=1283.0746}, {"X"=114.30515, "Y"=1286.0045}, {"X"=121.92117, "Y"=1277.0167}, {"X"=145.40562, "Y"=1258.6926}, {"X"=159.08377, "Y"=1243.3859}, {"X"=165.43448, "Y"=1218.9258}, {"X"=183.37242, "Y"=1196.9088}, {"X"=197.67096, "Y"=1187.2228}, {"X"=208.1446, "Y"=1132.849}, {"X"=216.4116, "Y"=1119.6353}, {"X"=224.86983, "Y"=1116.1626}, {"X"=231.21765, "Y"=1112.7327}, {"X"=227.83913, "Y"=1096.3147}, {"X"=219.73424, "Y"=1129.3307}, {"X"=194.46902, "Y"=1136.409}, {"X"=179.49799, "Y"=1168.7601}, {"X"=167.6472, "Y"=1191.0421}, {"X"=148.25287, "Y"=1143.9507}, {"X"=131.87415, "Y"=1105.2273}, {"X"=127.96529, "Y"=1137.9784}, {"X"=122.99322, "Y"=1235.1345}, {"X"=125.678246, "Y"=1271.0245}, {"X"=123.797806, "Y"=1274.0237}, {"X"=139.44537, "Y"=1261.808}, {"X"=167.97223, "Y"=1234.1118}, {"X"=195.4546, "Y"=1181.0046}, {"X"=214.64189, "Y"=1142.3878}, {"X"=257.80902, "Y"=1092.2755}, {"X"=289.2665, "Y"=1047.6812}, {"X"=294.70438, "Y"=1047.5487}, {"X"=304.2281, "Y"=1067.7042}, {"X"=314.87155, "Y"=1077.5441}, {"X"=323.4288, "Y"=1080.6897}, {"X"=312.66354, "Y"=1080.9487}, {"X"=356.05453, "Y"=993.89417}, {"X"=357.47052, "Y"=983.22156}, {"X"=355.55414, "Y"=972.56195}, {"X"=355.14905, "Y"=947.31213}, {"X"=349.37085, "Y"=910.6881}, {"X"=344.3757, "Y"=929.3021}, {"X"=323.1386, "Y"=918.77655}, {"X"=337.817, "Y"=969.4214}, {"X"=308.34183, "Y"=1005.64215}, {"X"=286.0288, "Y"=1044.3372}, {"X"=281.6946, "Y"=1041.0127}, {"X"=252.30298, "Y"=1048.5817}, {"X"=245.8923, "Y"=1069.115}, {"X"=234.2003, "Y"=1089.5137}, {"X"=219.23146, "Y"=1093.2004}, {"X"=202.09433, "Y"=1093.6113}, {"X"=192.15758, "Y"=1080.5007}, {"X"=187.42303, "Y"=1107.1989}, {"X"=182.99036, "Y"=1100.7009}, {"X"=191.70367, "Y"=1060.2744}, {"X"=204.62875, "Y"=1056.5621}, {"X"=217.63304, "Y"=1056.2461}, {"X"=231.95659, "Y"=1079.5419}, {"X"=253.4913, "Y"=1082.3727}, {"X"=236.23248, "Y"=1076.0825}, {"X"=242.76079, "Y"=1085.973}, {"X"=308.40628, "Y"=1077.6998}, {"X"=336.9787, "Y"=1053.3457}, {"X"=349.5097, "Y"=990.5188}, {"X"=364.46594, "Y"=972.33905}, {"X"=372.23102, "Y"=939.59076}, {"X"=378.24164, "Y"=928.44196}, {"X"=382.2936, "Y"=909.84656}, {"X"=378.65802, "Y"=883.7006}, {"X"=385.24936, "Y"=891.07}, {"X"=378.9834, "Y"=939.4199}, {"X"=369.98038, "Y"=939.6477}, {"X"=361.01614, "Y"=976.00244}, {"X"=358.47626, "Y"=986.7501}, {"X"=354.4488, "Y"=1011.5089}, {"X"=349.48328, "Y"=1032.4705}, {"X"=349.92032, "Y"=1056.4341}, {"X"=354.85483, "Y"=1073.221}, {"X"=363.38474, "Y"=1076.3752}, {"X"=374.05295, "Y"=1079.4714}, {"X"=413.98303, "Y"=1054.879}, {"X"=425.58667, "Y"=1061.386}, {"X"=441.72452, "Y"=1043.9668}, {"X"=432.27396, "Y"=1057.8331}, {"X"=431.72995, "Y"=1047.6302}, {"X"=419.7512, "Y"=1047.9218}, {"X"=411.04095, "Y"=1048.1337}, {"X"=386.9617, "Y"=1052.1309}, {"X"=381.5266, "Y"=1052.263}, {"X"=332.1895, "Y"=1073.7677}, {"X"=322.16357, "Y"=1090.7325}, {"X"=334.27182, "Y"=1077.0767}, {"X"=329.96008, "Y"=1077.1805}, {"X"=336.87714, "Y"=1103.6332}, {"X"=340.50528, "Y"=1171.3357}, {"X"=346.52228, "Y"=1180.6416}, {"X"=359.18127, "Y"=1142.2068}, {"X"=387.64792, "Y"=1062.3046}, {"X"=404.6555, "Y"=1185.5625}, {"X"=420.33853, "Y"=1243.4978}, {"X"=437.96283, "Y"=1290.499}, {"X"=444.1086, "Y"=1304.8695}, {"X"=441.63348, "Y"=1296.2374}, {"X"=434.78995, "Y"=1275.9196}, {"X"=422.00137, "Y"=1231.3727}, {"X"=408.22583, "Y"=1197.9398}, {"X"=395.18976, "Y"=1163.7313}, {"X"=377.37466, "Y"=1135.3282}, {"X"=362.74805, "Y"=1096.4017}, {"X"=341.40732, "Y"=1049.8281}, {"X"=343.88312, "Y"=994.19635}, {"X"=339.79312, "Y"=980.10126}, {"X"=341.07547, "Y"=972.92413}, {"X"=337.16434, "Y"=997.8929}, {"X"=329.213, "Y"=1008.6325}, {"X"=327.0105, "Y"=1008.68695}, {"X"=334.40924, "Y"=1022.45514}, {"X"=335.58145, "Y"=1066.946}, {"X"=331.4018, "Y"=1060.2786}, {"X"=330.10284, "Y"=1070.4519}, {"X"=330.5351, "Y"=1100.4818}, {"X"=334.66373, "Y"=1106.9818}, {"X"=331.53268, "Y"=1103.7606}, {"X"=318.64935, "Y"=1107.3634}, {"X"=294.10278, "Y"=1107.9482}, {"X"=257.75955, "Y"=1062.064}, {"X"=232.61368, "Y"=1035.3319}, {"X"=207.22366, "Y"=1018.6284}, {"X"=192.66629, "Y"=1004.99304}, {"X"=184.70451, "Y"=994.61523}, {"X"=184.03046, "Y"=1012.21857}, {"X"=188.50522, "Y"=1015.6026}, {"X"=193.34737, "Y"=1036.2935}, {"X"=201.57513, "Y"=1066.8099}, {"X"=215.14891, "Y"=1106.5374}, {"X"=218.34892, "Y"=1106.461}, {"X"=215.14891, "Y"=1106.5374}, {"X"=209.87184, "Y"=1109.9554}, {"X"=211.10472, "Y"=986.8688}, {"X"=221.25456, "Y"=1000.76666}, {"X"=224.74951, "Y"=1106.3083}, {"X"=228.02364, "Y"=1112.8087}, {"X"=238.67107, "Y"=1112.5553}, {"X"=258.91095, "Y"=1115.3534}, {"X"=274.8748, "Y"=1114.9739}, {"X"=286.53494, "Y"=1121.2373}, {"X"=295.13593, "Y"=1111.2114}, {"X"=287.57153, "Y"=1124.4727}, {"X"=268.45407, "Y"=1134.6631}, {"X"=245.46492, "Y"=1182.9836}, {"X"=229.12575, "Y"=1211.3246}, {"X"=194.13058, "Y"=1168.419}, {"X"=170.27744, "Y"=1140.2095}, {"X"=152.42903, "Y"=1200.7273}, {"X"=140.61429, "Y"=1240.787}, {"X"=126.63017, "Y"=1291.5796}, {"X"=134.39723, "Y"=1285.5568}, {"X"=148.23816, "Y"=1279.374}, {"X"=168.25916, "Y"=1243.178}, {"X"=187.09955, "Y"=1221.492}, {"X"=194.42914, "Y"=1227.4297}, {"X"=196.15233, "Y"=1165.2013}, {"X"=194.8146, "Y"=1103.7238}, {"X"=186.88753, "Y"=1039.8936}, {"X"=183.19157, "Y"=1022.6998}, {"X"=184.03046, "Y"=1012.21857}, {"X"=167.6202, "Y"=977.2628}, {"X"=150.35143, "Y"=926.87286}, {"X"=150.35143, "Y"=926.87286}, {"X"=384.0408, "Y"=1014.2719}, {"X"=387.3408, "Y"=1014.1906}, {"X"=394.6132, "Y"=1024.4463}, {"X"=407.6219, "Y"=1075.3094}, {"X"=413.45807, "Y"=1088.5437}, {"X"=417.61414, "Y"=1134.3799}, {"X"=425.62033, "Y"=1163.0219}, {"X"=435.18842, "Y"=1215.8241}, {"X"=440.7315, "Y"=1260.9899}, {"X"=439.36194, "Y"=1266.957}, {"X"=425.81512, "Y"=1255.3651}, {"X"=405.5841, "Y"=1231.7456}, {"X"=394.06964, "Y"=1213.6962}, {"X"=404.07596, "Y"=1198.0354}, {"X"=370.95517, "Y"=1167.4651}, {"X"=359.73346, "Y"=1158.2013}, {"X"=350.2792, "Y"=1158.4222}, {"X"=355.92535, "Y"=1109.7646}, {"X"=355.44553, "Y"=1052.8969}, {"X"=357.6185, "Y"=1052.844}, {"X"=353.759, "Y"=1035.8129}, {"X"=323.97195, "Y"=994.6906}, {"X"=292.9802, "Y"=998.98834}, {"X"=281.93954, "Y"=999.2621}, {"X"=269.77505, "Y"=1010.10065}, {"X"=262.07184, "Y"=999.7547}, {"X"=264.27756, "Y"=1003.2198}, {"X"=268.67493, "Y"=1010.1278}, {"X"=308.3912, "Y"=1002.12744}, {"X"=356.3603, "Y"=983.2492}, {"X"=352.93115, "Y"=986.8881}, {"X"=370.55972, "Y"=989.9956}, {"X"=358.8959, "Y"=972.4784}, {"X"=368.31427, "Y"=921.32275}, {"X"=382.56647, "Y"=837.6409}, {"X"=359.1968, "Y"=802.95575}, {"X"=372.25012, "Y"=834.0247}, {"X"=372.8794, "Y"=814.44147}, {"X"=373.00613, "Y"=810.4977}, {"X"=318.19775, "Y"=804.0427}, {"X"=319.63058, "Y"=788.086}, {"X"=313.7487, "Y"=788.24274}, {"X"=281.5745, "Y"=1061.4866}] {"Y" format="%.2f"; "X" format="%.2f"}
  in  "manual bottom FangYang vs Ueda":T1[](array[typedef])=[{"X"=328.9264, "Y"=1022.5899}, {"X"=326.73343, "Y"=1022.6438}, {"X"=329.42963, "Y"=998.08466}, {"X"=323.90546, "Y"=998.2216}, {"X"=313.85245, "Y"=1005.50586}, {"X"=312.5884, "Y"=1016.0324}, {"X"=309.3934, "Y"=1009.1221}, {"X"=315.23883, "Y"=987.8262}, {"X"=329.33743, "Y"=947.9635}, {"X"=361.52554, "Y"=921.4956}, {"X"=396.67096, "Y"=890.7762}, {"X"=407.76764, "Y"=871.57446}, {"X"=419.96964, "Y"=855.9692}, {"X"=424.03778, "Y"=867.3437}, {"X"=425.60135, "Y"=882.4898}, {"X"=431.70978, "Y"=874.7556}, {"X"=422.16516, "Y"=882.5784}, {"X"=400.56268, "Y"=879.35266}, {"X"=382.2936, "Y"=909.84656}, {"X"=375.8576, "Y"=932.17615}, {"X"=369.2727, "Y"=961.43945}, {"X"=370.09924, "Y"=935.98755}, {"X"=395.5287, "Y"=890.80554}, {"X"=422.8872, "Y"=867.37354}, {"X"=430.56165, "Y"=874.78534}, {"X"=437.4508, "Y"=874.6072}, {"X"=443.1924, "Y"=874.4587}, {"X"=444.54626, "Y"=870.62213}, {"X"=434.39404, "Y"=867.07513}, {"X"=424.63843, "Y"=878.73083}, {"X"=411.02228, "Y"=901.6553}, {"X"=388.1267, "Y"=935.5308}, {"X"=376.2298, "Y"=954.0384}, {"X"=367.2355, "Y"=990.07825}, {"X"=358.4368, "Y"=1025.3344}, {"X"=357.13736, "Y"=1032.283}, {"X"=352.95755, "Y"=1025.4688}, {"X"=345.93488, "Y"=1042.8757}, {"X"=339.33716, "Y"=1090.3208}, {"X"=332.7487, "Y"=1097.1193}, {"X"=340.16547, "Y"=1100.2517}, {"X"=355.44214, "Y"=1089.9347}, {"X"=377.87512, "Y"=1092.7219}, {"X"=388.34192, "Y"=1099.101}, {"X"=391.69107, "Y"=1095.7095}, {"X"=393.1762, "Y"=1085.6975}, {"X"=379.07108, "Y"=1089.3682}, {"X"=368.48456, "Y"=1052.58}, {"X"=349.2971, "Y"=1039.3616}, {"X"=324.27527, "Y"=1036.5338}, {"X"=326.4587, "Y"=1036.4805}, {"X"=315.2607, "Y"=1053.8734}, {"X"=313.03577, "Y"=1057.3293}, {"X"=297.63245, "Y"=1077.9595}, {"X"=283.36923, "Y"=1118.0455}, {"X"=288.4991, "Y"=1140.6492}, {"X"=289.11887, "Y"=1191.355}, {"X"=292.02594, "Y"=1212.9595}, {"X"=290.60107, "Y"=1255.4221}, {"X"=289.29382, "Y"=1287.9624}, {"X"=286.37018, "Y"=1276.288}, {"X"=286.44037, "Y"=1267.4203}, {"X"=280.27902, "Y"=1282.305}, {"X"=274.21268, "Y"=1288.2977}, {"X"=270.23505, "Y"=1270.7444}, {"X"=258.04288, "Y"=1235.0964}, {"X"=253.9043, "Y"=1219.9657}, {"X"=254.90817, "Y"=1210.7334}, {"X"=257.92606, "Y"=1163.7594}, {"X"=257.89993, "Y"=1147.8}, {"X"=264.22507, "Y"=1131.5239}, {"X"=264.23038, "Y"=1118.5}, {"X"=264.24255, "Y"=1088.7926}, {"X"=265.35132, "Y"=1041.4119}, {"X"=251.06313, "Y"=1007.0587}, {"X"=219.9646, "Y"=986.648}, {"X"=186.26138, "Y"=918.5661}, {"X"=160.82816, "Y"=900.5933}, {"X"=153.85449, "Y"=930.4665}, {"X"=149.59413, "Y"=904.62274}, {"X"=149.21164, "Y"=893.3851}, {"X"=150.72888, "Y"=904.5936}, {"X"=173.19908, "Y"=937.31683}, {"X"=197.53145, "Y"=972.9349}, {"X"=201.07138, "Y"=983.5624}, {"X"=211.44264, "Y"=1008.0386}, {"X"=229.26788, "Y"=1028.5049}, {"X"=241.459, "Y"=1052.2601}, {"X"=253.43065, "Y"=1062.1688}, {"X"=254.50383, "Y"=1058.7501}, {"X"=239.28818, "Y"=1052.313}, {"X"=227.50203, "Y"=1066.1821}, {"X"=211.46107, "Y"=1076.6802}, {"X"=204.42188, "Y"=1103.4943}, {"X"=191.91205, "Y"=1116.946}, {"X"=186.57733, "Y"=1159.0647}, {"X"=177.75961, "Y"=1181.4153}, {"X"=174.05371, "Y"=1197.1238}, {"X"=177.26346, "Y"=1236.9312}, {"X"=170.29834, "Y"=1243.1317}, {"X"=171.78676, "Y"=1224.8969}, {"X"=185.20494, "Y"=1187.5114}, {"X"=200.07835, "Y"=1152.3616}, {"X"=213.69005, "Y"=1148.8383}, {"X"=243.95558, "Y"=1105.8501}, {"X"=268.5653, "Y"=1071.9382}, {"X"=274.01956, "Y"=1054.8757}, {"X"=283.94177, "Y"=1030.6228}, {"X"=290.8631, "Y"=988.4328}, {"X"=302.28558, "Y"=959.5146}, {"X"=309.64694, "Y"=991.50964}, {"X"=316.92438, "Y"=1019.409}, {"X"=315.6558, "Y"=1029.8452}, {"X"=322.0919, "Y"=1036.5873}, {"X"=332.36618, "Y"=1015.5451}, {"X"=211.55429, "Y"=1015.034}, {"X"=215.74097, "Y"=1000.9034}, {"X"=226.53076, "Y"=979.3621}, {"X"=228.44855, "Y"=950.50964}, {"X"=231.70496, "Y"=939.4936}, {"X"=230.68855, "Y"=950.4531}, {"X"=231.70496, "Y"=939.4936}, {"X"=237.32413, "Y"=939.3512}, {"X"=240.76974, "Y"=950.19867}, {"X"=244.21342, "Y"=964.5795}, {"X"=248.79973, "Y"=993.02203}, {"X"=250.0184, "Y"=1021.0554}, {"X"=246.8692, "Y"=1048.7141}, {"X"=250.15686, "Y"=1055.4557}, {"X"=256.7173, "Y"=1082.295}, {"X"=261.01886, "Y"=1082.1915}, {"X"=257.79263, "Y"=1082.2692}, {"X"=251.34074, "Y"=1082.4244}, {"X"=245.92859, "Y"=1075.8486}, {"X"=228.61919, "Y"=1069.5327}, {"X"=198.197, "Y"=1060.1168}, {"X"=164.20749, "Y"=1081.1742}, {"X"=155.83763, "Y"=1088.0623}, {"X"=155.61024, "Y"=1081.3813}, {"X"=165.17844, "Y"=1077.7966}, {"X"=198.40395, "Y"=1070.2634}, {"X"=243.855, "Y"=1089.282}, {"X"=261.0168, "Y"=1078.8417}, {"X"=274.00772, "Y"=1058.2766}, {"X"=295.27188, "Y"=1098.0155}, {"X"=313.3653, "Y"=1104.1941}, {"X"=323.36465, "Y"=1084.0358}, {"X"=328.6726, "Y"=1087.246}, {"X"=333.19385, "Y"=1077.1027}, {"X"=339.33716, "Y"=1090.3208}, {"X"=336.19424, "Y"=1087.0653}, {"X"=339.92178, "Y"=1110.1455}, {"X"=339.01508, "Y"=1103.5822}, {"X"=319.59756, "Y"=1113.9108}, {"X"=299.32324, "Y"=1117.6667}, {"X"=390.09232, "Y"=1000.1043}, {"X"=389.81598, "Y"=1007.1356}, {"X"=389.81598, "Y"=1007.1356}, {"X"=395.3773, "Y"=978.7144}, {"X"=403.93625, "Y"=960.5691}, {"X"=398.94354, "Y"=946.20685}, {"X"=399.91528, "Y"=949.8163}, {"X"=397.9697, "Y"=942.58954}, {"X"=395.86786, "Y"=938.99274}, {"X"=386.04276, "Y"=961.0184}, {"X"=388.00345, "Y"=968.1645}, {"X"=384.96686, "Y"=989.6375}, {"X"=379.04474, "Y"=1000.37787}, {"X"=365.88617, "Y"=1032.0687}, {"X"=354.16367, "Y"=1059.7268}, {"X"=352.9833, "Y"=1063.1439}, {"X"=365.76047, "Y"=1069.5906}, {"X"=378.4862, "Y"=1076.0114}, {"X"=380.18845, "Y"=1059.0958}, {"X"=380.18845, "Y"=1059.0958}, {"X"=383.44238, "Y"=1059.017}, {"X"=387.5149, "Y"=1065.6901}, {"X"=386.56433, "Y"=1062.3308}, {"X"=368.14648, "Y"=1062.7767}, {"X"=360.46027, "Y"=1066.3444}, {"X"=359.48132, "Y"=1062.9866}, {"X"=362.17728, "Y"=1045.9048}, {"X"=363.48206, "Y"=1039.0151}, {"X"=362.4979, "Y"=1035.5991}, {"X"=367.62213, "Y"=1045.7721}, {"X"=376.71158, "Y"=1003.9513}, {"X"=380.71176, "Y"=953.9256}, {"X"=383.2945, "Y"=913.536}, {"X"=377.2719, "Y"=857.08057}, {"X"=378.2943, "Y"=860.8879}, {"X"=376.88324, "Y"=868.5663}, {"X"=368.04422, "Y"=857.32074}, {"X"=357.23605, "Y"=872.88293}, {"X"=351.29672, "Y"=880.62506}, {"X"=346.24576, "Y"=899.5765}, {"X"=326.6054, "Y"=914.9832}, {"X"=308.79025, "Y"=973.7317}, {"X"=296.1842, "Y"=1009.44836}, {"X"=289.52307, "Y"=1016.6007}, {"X"=276.2463, "Y"=1041.1458}, {"X"=271.8403, "Y"=1058.3292}, {"X"=270.69043, "Y"=1085.3018}, {"X"=267.45755, "Y"=1092.0442}, {"X"=263.16867, "Y"=1098.7833}, {"X"=255.63417, "Y"=1078.9713}, {"X"=249.17566, "Y"=1079.127}, {"X"=222.40237, "Y"=1089.7969}, {"X"=222.31633, "Y"=1083.1228}, {"X"=221.37398, "Y"=1093.149}, {"X"=223.43297, "Y"=1086.4376}, {"X"=240.66019, "Y"=1092.6866}, {"X"=253.4913, "Y"=1082.3727}, {"X"=261.02298, "Y"=1088.8699}, {"X"=268.5356, "Y"=1088.6895}, {"X"=277.15277, "Y"=1081.8032}, {"X"=286.7595, "Y"=1091.5814}, {"X"=281.41672, "Y"=1088.3802}, {"X"=277.18295, "Y"=1075.0947}, {"X"=254.5755, "Y"=1085.6891}, {"X"=218.20757, "Y"=1096.5453}, {"X"=174.35126, "Y"=1097.5956}, {"X"=123.638725, "Y"=1112.0103}, {"X"=89.242546, "Y"=1106.2456}, {"X"=75.86843, "Y"=1096.6377}, {"X"=76.93695, "Y"=1096.612}, {"X"=103.71637, "Y"=1075.9198}, {"X"=124.9444, "Y"=1068.6654}, {"X"=157.19817, "Y"=1064.5018}, {"X"=201.57513, "Y"=1066.8099}, {"X"=231.98947, "Y"=1082.89}, {"X"=257.78717, "Y"=1078.9194}, {"X"=277.25903, "Y"=1058.1978}, {"X"=210.39955, "Y"=1011.56726}, {"X"=213.74994, "Y"=1014.97986}, {"X"=213.48183, "Y"=997.4335}, {"X"=216.5913, "Y"=983.1752}, {"X"=221.63766, "Y"=943.401}, {"X"=229.56854, "Y"=950.4814}, {"X"=236.2299, "Y"=943.0318}, {"X"=232.559, "Y"=909.9556}, {"X"=241.77289, "Y"=931.9081}, {"X"=238.42082, "Y"=935.6624}, {"X"=245.0529, "Y"=913.3547}, {"X"=245.07289, "Y"=917.0647}, {"X"=249.644, "Y"=928.03046}, {"X"=246.31598, "Y"=939.1234}, {"X"=251.93661, "Y"=938.981}, {"X"=262.0621, "Y"=964.13135}, {"X"=262.07278, "Y"=1003.27435}, {"X"=277.30508, "Y"=1047.9725}, {"X"=284.6835, "Y"=1081.6221}, {"X"=294.20148, "Y"=1098.0411}, {"X"=320.8761, "Y"=1159.1094}, {"X"=348.43207, "Y"=1186.8623}, {"X"=369.79596, "Y"=1229.5227}, {"X"=388.159, "Y"=1256.2123}, {"X"=386.24786, "Y"=1253.2676}, {"X"=382.77588, "Y"=1238.3175}, {"X"=366.9275, "Y"=1223.498}, {"X"=363.1189, "Y"=1214.404}, {"X"=363.52798, "Y"=1202.0662}, {"X"=364.6704, "Y"=1167.6115}, {"X"=361.80798, "Y"=1125.9698}, {"X"=358.26004, "Y"=1103.1229}, {"X"=338.5839, "Y"=1076.9728}, {"X"=334.81506, "Y"=1100.3795}, {"X"=337.78833, "Y"=1110.1963}, {"X"=336.56674, "Y"=1116.7826}, {"X"=358.62332, "Y"=1126.0452}, {"X"=389.5503, "Y"=1147.9174}, {"X"=421.71497, "Y"=1197.6295}, {"X"=455.2392, "Y"=1224.5356}, {"X"=464.92044, "Y"=1248.4998}, {"X"=454.46274, "Y"=1236.6931}, {"X"=437.0748, "Y"=1218.8433}, {"X"=423.08023, "Y"=1191.38}, {"X"=412.22336, "Y"=1200.947}, {"X"=399.10455, "Y"=1169.9727}, {"X"=377.35876, "Y"=1164.147}, {"X"=348.45645, "Y"=1109.9424}, {"X"=327.59818, "Y"=1087.2717}, {"X"=298.67178, "Y"=1081.2854}, {"X"=288.9872, "Y"=1081.5184}, {"X"=289.92007, "Y"=1098.1436}, {"X"=293.9722, "Y"=1121.0609}, {"X"=308.5153, "Y"=1143.3981}, {"X"=340.90726, "Y"=1155.4535}, {"X"=367.38135, "Y"=1180.1582}, {"X"=405.1134, "Y"=1198.0115}, {"X"=428.15906, "Y"=1231.2329}, {"X"=437.89258, "Y"=1240.0879}, {"X"=435.8458, "Y"=1240.1342}, {"X"=415.33298, "Y"=1200.8756}, {"X"=398.40567, "Y"=1185.707}, {"X"=400.20706, "Y"=1191.9076}, {"X"=389.8136, "Y"=1167.026}, {"X"=379.49182, "Y"=1135.2783}, {"X"=372.39407, "Y"=1096.171}, {"X"=363.06537, "Y"=1086.4203}, {"X"=348.1062, "Y"=1083.4412}, {"X"=340.49277, "Y"=1086.9622}, {"X"=325.3832, "Y"=1090.6554}, {"X"=288.68674, "Y"=1117.9193}, {"X"=263.16577, "Y"=1141.2456}, {"X"=238.10252, "Y"=1173.7174}, {"X"=208.67398, "Y"=1220.999}, {"X"=186.86803, "Y"=1212.2935}, {"X"=167.68355, "Y"=1224.9905}, {"X"=159.29253, "Y"=1249.3987}, {"X"=144.93272, "Y"=1246.7179}, {"X"=151.61208, "Y"=1234.4838}, {"X"=175.85724, "Y"=1187.7278}, {"X"=183.76007, "Y"=1171.8243}, {"X"=181.41983, "Y"=1162.3687}, {"X"=176.78542, "Y"=1146.4954}, {"X"=176.94392, "Y"=1114.0244}, {"X"=399.88785, "Y"=1003.3781}, {"X"=401.29272, "Y"=996.3029}, {"X"=400.27805, "Y"=967.85706}, {"X"=403.31732, "Y"=974.9457}, {"X"=397.22552, "Y"=960.7376}, {"X"=390.5156, "Y"=960.90607}, {"X"=381.7011, "Y"=957.518}, {"X"=381.57025, "Y"=961.1307}, {"X"=362.02023, "Y"=979.5467}, {"X"=342.86395, "Y"=990.684}, {"X"=320.15497, "Y"=1022.8055}, {"X"=307.9505, "Y"=1033.4873}, {"X"=289.43698, "Y"=1027.028}, {"X"=278.32642, "Y"=1061.5653}, {"X"=261.01062, "Y"=1068.7494}, {"X"=264.25354, "Y"=1061.9065}, {"X"=241.55072, "Y"=1065.842}, {"X"=216.747, "Y"=1069.8198}, {"X"=197.0189, "Y"=1106.9698}, {"X"=175.5511, "Y"=1140.0852}, {"X"=153.74623, "Y"=1150.246}, {"X"=137.05678, "Y"=1179.2169}, {"X"=124.055275, "Y"=1213.7335}, {"X"=114.96846, "Y"=1238.346}, {"X"=102.83165, "Y"=1259.6516}, {"X"=110.9385, "Y"=1259.469}, {"X"=135.38547, "Y"=1237.8822}, {"X"=161.22012, "Y"=1215.955}, {"X"=168.0362, "Y"=1203.4666}, {"X"=180.4579, "Y"=1165.5676}, {"X"=197.77379, "Y"=1142.7849}, {"X"=210.03883, "Y"=1119.7866}, {"X"=215.04802, "Y"=1099.9342}, {"X"=229.83974, "Y"=1082.9418}, {"X"=241.70937, "Y"=1089.3335}, {"X"=236.26086, "Y"=1079.4381}, {"X"=226.6153, "Y"=1083.0194}, {"X"=200.82637, "Y"=1083.64}, {"X"=178.00761, "Y"=1113.999}, {"X"=171.7123, "Y"=1153.0269}, {"X"=150.93758, "Y"=1188.3046}, {"X"=143.36049, "Y"=1153.6919}, {"X"=136.4062, "Y"=1188.6409}, {"X"=142.09125, "Y"=1200.9655}, {"X"=122.228264, "Y"=1262.1954}, {"X"=125.453415, "Y"=1244.1478}, {"X"=127.21778, "Y"=1238.0677}, {"X"=138.96948, "Y"=1225.6458}, {"X"=154.60745, "Y"=1203.7755}, {"X"=195.94461, "Y"=1155.6553}, {"X"=226.95901, "Y"=1112.834}, {"X"=286.2036, "Y"=1020.165}, {"X"=296.0048, "Y"=1026.8668}, {"X"=294.97925, "Y"=1019.94904}, {"X"=323.64096, "Y"=1012.2689}, {"X"=339.8926, "Y"=1022.3204}, {"X"=345.73465, "Y"=1008.2244}, {"X"=353.62515, "Y"=961.83234}, {"X"=354.2286, "Y"=940.04626}, {"X"=359.42276, "Y"=876.62506}, {"X"=355.56915, "Y"=849.95294}, {"X"=358.31537, "Y"=834.39026}, {"X"=350.94638, "Y"=850.0736}, {"X"=349.39676, "Y"=865.4634}, {"X"=347.95712, "Y"=876.9216}, {"X"=319.4279, "Y"=937.27124}, {"X"=302.24225, "Y"=963.1225}, {"X"=291.97086, "Y"=988.4052}, {"X"=276.43472, "Y"=995.8707}, {"X"=266.45956, "Y"=1024.1251}, {"X"=240.34937, "Y"=1048.8729}, {"X"=234.97675, "Y"=1055.8246}, {"X"=220.97441, "Y"=1062.9557}, {"X"=216.69771, "Y"=1066.4437}, {"X"=212.37656, "Y"=1066.5485}, {"X"=189.14505, "Y"=1043.2731}, {"X"=182.35814, "Y"=1033.1132}, {"X"=191.0118, "Y"=1029.444}, {"X"=203.2257, "Y"=1039.494}, {"X"=218.43103, "Y"=1035.6792}, {"X"=246.7999, "Y"=1034.9846}, {"X"=274.10312, "Y"=1030.864}, {"X"=289.29477, "Y"=1044.2574}, {"X"=301.3128, "Y"=1040.5336}, {"X"=326.73343, "Y"=1022.6438}, {"X"=348.96567, "Y"=969.14215}, {"X"=365.82178, "Y"=928.75745}, {"X"=376.4972, "Y"=879.9742}, {"X"=381.2139, "Y"=876.0615}, {"X"=395.88303, "Y"=852.75287}, {"X"=392.1448, "Y"=829.6067}, {"X"=393.72147, "Y"=848.9573}, {"X"=387.5132, "Y"=860.64825}, {"X"=367.53275, "Y"=910.2239}, {"X"=362.7683, "Y"=917.7661}, {"X"=351.68344, "Y"=951.0319}, {"X"=349.06033, "Y"=965.54736}, {"X"=346.46033, "Y"=979.9349}, {"X"=346.65442, "Y"=1015.19305}, {"X"=353.8569, "Y"=1032.3633}, {"X"=346.39697, "Y"=1066.6844}, {"X"=366.42203, "Y"=1049.2194}, {"X"=405.29233, "Y"=1055.09}, {"X"=428.4392, "Y"=1027.0803}, {"X"=441.40094, "Y"=1030.2198}, {"X"=451.25812, "Y"=1029.9785}, {"X"=448.37234, "Y"=1023.1267}, {"X"=433.7354, "Y"=1030.4075}, {"X"=429.17624, "Y"=1033.9685}, {"X"=423.65332, "Y"=1013.29596}, {"X"=407.30127, "Y"=1010.2051}, {"X"=382.81088, "Y"=1017.7877}, {"X"=357.64786, "Y"=1014.92224}, {"X"=336.12772, "Y"=1043.115}, {"X"=327.8299, "Y"=1022.6169}, {"X"=326.25424, "Y"=1046.78}, {"X"=320.199, "Y"=1080.7673}, {"X"=319.71683, "Y"=1107.3379}, {"X"=334.82333, "Y"=1145.9935}, {"X"=358.1897, "Y"=1174.0797}, {"X"=379.98032, "Y"=1122.284}, {"X"=401.85913, "Y"=1201.1853}, {"X"=433.1128, "Y"=1252.212}, {"X"=465.34375, "Y"=1315.9061}, {"X"=456.65344, "Y"=1281.3102}, {"X"=447.38373, "Y"=1251.8905}, {"X"=433.46344, "Y"=1228.075}, {"X"=415.4888, "Y"=1197.7727}, {"X"=404.9256, "Y"=1157.145}, {"X"=394.07635, "Y"=1115.4171}, {"X"=369.9701, "Y"=1072.8563}, {"X"=360.26877, "Y"=1000.84283}, {"X"=345.53006, "Y"=972.8127}, {"X"=347.38657, "Y"=987.02606}, {"X"=350.08066, "Y"=969.11426}, {"X"=342.62656, "Y"=954.8843}, {"X"=335.82782, "Y"=958.6713}, {"X"=328.97217, "Y"=966.0511}, {"X"=334.00418, "Y"=990.90424}, {"X"=328.1826, "Y"=1005.1515}, {"X"=326.73343, "Y"=1022.6438}, {"X"=323.2485, "Y"=1033.1128}, {"X"=322.79697, "Y"=1057.0924}, {"X"=333.3435, "Y"=1070.3735}, {"X"=337.26883, "Y"=1087.0396}, {"X"=334.0451, "Y"=1087.117}, {"X"=322.542, "Y"=1070.6345}, {"X"=292.18417, "Y"=1084.7852}, {"X"=256.64362, "Y"=1045.054}, {"X"=219.91754, "Y"=983.09216}, {"X"=202.4447, "Y"=997.7075}, {"X"=186.66386, "Y"=983.9219}, {"X"=177.88358, "Y"=944.508}, {"X"=177.42519, "Y"=969.85144}, {"X"=182.67076, "Y"=1001.7233}, {"X"=186.5589, "Y"=1026.0889}, {"X"=205.46631, "Y"=1042.8745}, {"X"=220.07599, "Y"=1076.4723}, {"X"=230.88057, "Y"=1079.5677}, {"X"=221.28584, "Y"=1086.4893}, {"X"=224.54727, "Y"=1089.7455}, {"X"=225.58018, "Y"=1086.386}, {"X"=217.96996, "Y"=1079.8788}, {"X"=221.37398, "Y"=1093.149}, {"X"=223.39104, "Y"=1083.0969}, {"X"=243.75334, "Y"=1072.5375}, {"X"=270.73166, "Y"=1068.5143}, {"X"=294.30078, "Y"=1088.071}, {"X"=299.82623, "Y"=1074.5485}, {"X"=303.0191, "Y"=1077.8297}, {"X"=288.84976, "Y"=1098.1691}, {"X"=262.10602, "Y"=1125.0758}, {"X"=247.45119, "Y"=1164.0039}, {"X"=222.48668, "Y"=1177.2323}, {"X"=190.17482, "Y"=1177.9829}, {"X"=169.81734, "Y"=1194.1099}, {"X"=155.4846, "Y"=1228.3173}, {"X"=126.55183, "Y"=1268.0419}, {"X"=123.06801, "Y"=1279.9364}, {"X"=131.4741, "Y"=1264.9624}, {"X"=157.70612, "Y"=1203.7042}, {"X"=186.89232, "Y"=1171.7513}, {"X"=212.16602, "Y"=1183.7552}, {"X"=214.59155, "Y"=1139.165}, {"X"=208.63503, "Y"=1100.0876}, {"X"=204.18866, "Y"=1032.578}, {"X"=191.72017, "Y"=1012.0286}, {"X"=177.70625, "Y"=980.58185}, {"X"=172.07524, "Y"=937.34534}, {"X"=165.4827, "Y"=904.215}, {"X"=151.86365, "Y"=904.5645}, {"X"=389.12488, "Y"=996.6046}, {"X"=392.86804, "Y"=985.89417}, {"X"=386.3449, "Y"=982.502}, {"X"=399.59055, "Y"=1010.3953}, {"X"=406.05835, "Y"=1037.9752}, {"X"=406.3786, "Y"=1055.0636}, {"X"=417.59412, "Y"=1091.7708}, {"X"=426.8066, "Y"=1140.6167}, {"X"=432.96277, "Y"=1181.7764}, {"X"=441.1976, "Y"=1218.7491}, {"X"=430.71234, "Y"=1203.6156}, {"X"=402.10193, "Y"=1173.0597}, {"X"=397.50223, "Y"=1182.5972}, {"X"=390.86148, "Y"=1167.0016}, {"X"=380.55045, "Y"=1135.2534}, {"X"=366.5969, "Y"=1109.5106}, {"X"=363.81973, "Y"=1096.3761}, {"X"=371.51218, "Y"=1059.3063}, {"X"=360.84018, "Y"=1018.3283}, {"X"=339.79312, "Y"=980.10126}, {"X"=323.5267, "Y"=958.9805}, {"X"=313.85703, "Y"=933.7489}, {"X"=310.53, "Y"=930.16174}, {"X"=300.17325, "Y"=948.6995}, {"X"=290.08145, "Y"=948.9542}, {"X"=287.81158, "Y"=952.64185}, {"X"=286.71793, "Y"=949.0391}, {"X"=302.11285, "Y"=973.89874}, {"X"=307.72647, "Y"=970.17505}, {"X"=346.63278, "Y"=929.2448}, {"X"=374.4698, "Y"=906.3234}, {"X"=373.97217, "Y"=921.17865}, {"X"=383.83517, "Y"=898.6119}, {"X"=382.7675, "Y"=864.597}, {"X"=389.23468, "Y"=814.0095}, {"X"=379.4297, "Y"=758.26117}, {"X"=381.80438, "Y"=758.19727}, {"X"=387.57516, "Y"=729.343}, {"X"=391.77533, "Y"=712.61523}, {"X"=373.20947, "Y"=729.73315}, {"X"=347.47995, "Y"=755.0511}, {"X"=335.5158, "Y"=759.44257}, {"X"=314.2246, "Y"=755.9469}, {"X"=-379.219, "Y"=-1944.1919}] {"Y" format="%.2f"; "X" format="%.2f"}
  in  "auto top ChenJin vs DuPengYu":T1[](array[typedef])=[{"X"=288.0406, "Y"=182.67284}, {"X"=308.2389, "Y"=133.07611}, {"X"=300.85416, "Y"=151.20926}, {"X"=296.96878, "Y"=173.83543}, {"X"=295.00314, "Y"=187.33553}, {"X"=293.7917, "Y"=267.28165}, {"X"=294.45398, "Y"=336.57956}, {"X"=298.15305, "Y"=319.4983}, {"X"=303.89093, "Y"=284.98685}, {"X"=315.57, "Y"=306.95084}, {"X"=319.60938, "Y"=276.61542}, {"X"=324.26416, "Y"=302.82043}, {"X"=322.54178, "Y"=302.78146}, {"X"=317.1562, "Y"=223.6457}, {"X"=319.95352, "Y"=259.09164}, {"X"=320.213, "Y"=245.87904}, {"X"=301.44354, "Y"=223.294}, {"X"=270.366, "Y"=191.28714}, {"X"=249.47635, "Y"=168.25151}, {"X"=238.9849, "Y"=154.39336}, {"X"=226.7244, "Y"=126.68263}, {"X"=223.17773, "Y"=126.60424}, {"X"=221.40443, "Y"=126.56505}, {"X"=217.87636, "Y"=117.28437}, {"X"=230.32771, "Y"=112.94699}, {"X"=253.29005, "Y"=131.86093}, {"X"=277.88095, "Y"=150.69997}, {"X"=294.73105, "Y"=205.2913}, {"X"=303.48645, "Y"=205.48682}, {"X"=310.7312, "Y"=192.18687}, {"X"=322.48282, "Y"=219.31165}, {"X"=331.626, "Y"=281.25278}, {"X"=343.52173, "Y"=290.23465}, {"X"=348.9166, "Y"=281.64273}, {"X"=348.9166, "Y"=281.64273}, {"X"=370.3977, "Y"=376.56277}, {"X"=376.6957, "Y"=393.54694}, {"X"=389.99347, "Y"=402.23444}, {"X"=398.19925, "Y"=308.82074}, {"X"=396.62802, "Y"=406.56885}, {"X"=370.2758, "Y"=380.77936}, {"X"=378.9037, "Y"=376.757}, {"X"=371.97568, "Y"=380.8182}, {"X"=358.8303, "Y"=363.60336}, {"X"=330.12766, "Y"=350.19812}, {"X"=310.4855, "Y"=302.5088}, {"X"=305.54327, "Y"=289.37717}, {"X"=296.70798, "Y"=302.19717}, {"X"=287.91287, "Y"=314.9589}, {"X"=279.82062, "Y"=275.71857}, {"X"=277.8197, "Y"=297.43692}, {"X"=270.53854, "Y"=331.75488}, {"X"=251.52797, "Y"=352.66507}, {"X"=234.40248, "Y"=365.0035}, {"X"=224.1484, "Y"=377.44104}, {"X"=212.25989, "Y"=377.16946}, {"X"=207.1714, "Y"=347.39996}, {"X"=213.98798, "Y"=356.05914}, {"X"=215.69987, "Y"=351.84927}, {"X"=224.32544, "Y"=322.12476}, {"X"=234.52985, "Y"=339.49265}, {"X"=243.21873, "Y"=318.25302}, {"X"=246.6516, "Y"=318.33084}, {"X"=245.14061, "Y"=288.01334}, {"X"=212.34041, "Y"=304.61475}, {"X"=210.64159, "Y"=278.52423}, {"X"=205.45476, "Y"=234.46014}, {"X"=222.86363, "Y"=234.85048}, {"X"=222.8124, "Y"=252.50897}, {"X"=222.79964, "Y"=256.9069}, {"X"=226.16138, "Y"=287.58484}, {"X"=241.68968, "Y"=287.93542}, {"X"=254.02156, "Y"=257.609}, {"X"=262.14246, "Y"=314.37506}, {"X"=272.8513, "Y"=279.92725}, {"X"=274.3219, "Y"=301.69086}, {"X"=272.60004, "Y"=301.65192}, {"X"=274.73526, "Y"=266.85263}, {"X"=266.48572, "Y"=226.95732}, {"X"=252.78308, "Y"=195.38855}, {"X"=254.57356, "Y"=190.93513}, {"X"=252.78308, "Y"=195.38855}, {"X"=251.44745, "Y"=140.98119}, {"X"=244.60835, "Y"=104.01568}, {"X"=244.72885, "Y"=85.439186}, {"X"=212.60518, "Y"=66.039665}, {"X"=209.0156, "Y"=79.9919}, {"X"=210.80258, "Y"=80.03115}, {"X"=221.47652, "Y"=98.87238}, {"X"=224.89243, "Y"=144.96277}, {"X"=230.12149, "Y"=163.28682}, {"X"=235.43167, "Y"=158.86314}, {"X"=252.64023, "Y"=213.29016}, {"X"=266.11945, "Y"=262.27316}, {"X"=269.58652, "Y"=262.35117}, {"X"=273.41083, "Y"=231.55151}, {"X"=279.98822, "Y"=262.58524}, {"X"=275.10107, "Y"=236.02177}, {"X"=284.28503, "Y"=200.57802}, {"X"=281.29892, "Y"=159.88121}, {"X"=277.99203, "Y"=141.56894}, {"X"=281.4733, "Y"=146.21634}, {"X"=280.22055, "Y"=104.80031}, {"X"=262.6337, "Y"=81.169556}, {"X"=257.39145, "Y"=67.02148}, {"X"=232.14586, "Y"=103.7411}, {"X"=219.73785, "Y"=80.2274}, {"X"=228.60292, "Y"=99.0293}, {"X"=241.02031, "Y"=108.56333}, {"X"=246.04617, "Y"=154.54999}, {"X"=251.09889, "Y"=186.35748}, {"X"=271.71802, "Y"=227.07451}, {"X"=279.98822, "Y"=262.58524}, {"X"=279.93225, "Y"=266.96964}, {"X"=262.31143, "Y"=297.08636}, {"X"=227.73904, "Y"=326.49582}, {"X"=222.57318, "Y"=334.9465}, {"X"=208.91833, "Y"=269.74896}, {"X"=222.73611, "Y"=278.797}, {"X"=222.59805, "Y"=326.37915}, {"X"=232.92055, "Y"=318.0196}, {"X"=245.14061, "Y"=288.01334}, {"X"=255.30801, "Y"=309.9069}, {"X"=264.1658, "Y"=284.09042}, {"X"=280.98416, "Y"=319.1091}, {"X"=305.16974, "Y"=311.03592}, {"X"=312.60843, "Y"=280.82388}, {"X"=328.44525, "Y"=268.06183}, {"X"=340.0688, "Y"=290.15668}, {"X"=351.19345, "Y"=259.79416}, {"X"=352.59613, "Y"=272.98553}, {"X"=364.71912, "Y"=273.25864}, {"X"=380.43893, "Y"=269.23242}, {"X"=411.95435, "Y"=261.16055}, {"X"=426.17914, "Y"=252.67204}, {"X"=433.48083, "Y"=244.00073}, {"X"=440.98386, "Y"=230.86539}, {"X"=465.23062, "Y"=235.85004}, {"X"=465.23062, "Y"=235.85004}, {"X"=425.98633, "Y"=348.11542}, {"X"=418.66812, "Y"=360.72226}, {"X"=411.1052, "Y"=427.72137}, {"X"=405.1665, "Y"=452.36823}, {"X"=401.95187, "Y"=448.1787}, {"X"=418.19424, "Y"=373.4279}, {"X"=421.12073, "Y"=386.1547}, {"X"=412.80484, "Y"=473.03192}, {"X"=406.6986, "Y"=456.51297}, {"X"=402.5768, "Y"=381.5173}, {"X"=394.35532, "Y"=372.88388}, {"X"=385.07068, "Y"=342.91473}, {"X"=381.7736, "Y"=282.38373}, {"X"=373.25256, "Y"=277.82452}, {"X"=368.06055, "Y"=277.7075}, {"X"=352.37494, "Y"=281.7207}, {"X"=340.2711, "Y"=281.44772}, {"X"=323.87067, "Y"=237.1153}, {"X"=311.4365, "Y"=250.09474}, {"X"=304.4849, "Y"=249.9386}, {"X"=304.03873, "Y"=276.26443}, {"X"=236.17215, "Y"=352.3154}, {"X"=227.54527, "Y"=377.51865}, {"X"=217.3718, "Y"=368.84506}, {"X"=217.28764, "Y"=410.80026}, {"X"=217.28764, "Y"=410.80026}, {"X"=215.7217, "Y"=339.0651}, {"X"=219.17079, "Y"=326.3014}, {"X"=219.05322, "Y"=377.32465}, {"X"=220.71877, "Y"=389.97778}, {"X"=222.52368, "Y"=352.00464}, {"X"=227.69028, "Y"=339.3372}, {"X"=229.38266, "Y"=343.64374}, {"X"=232.84, "Y"=335.17975}, {"X"=239.68488, "Y"=335.33527}, {"X"=243.21873, "Y"=318.25302}, {"X"=246.6516, "Y"=318.33084}, {"X"=243.55669, "Y"=266.15067}, {"X"=231.414, "Y"=270.2557}, {"X"=219.31067, "Y"=265.6048}, {"X"=224.63301, "Y"=226.01999}, {"X"=212.44275, "Y"=212.39148}, {"X"=233.33063, "Y"=230.65335}, {"X"=233.18568, "Y"=261.53214}, {"X"=240.22224, "Y"=244.08337}, {"X"=250.08455, "Y"=318.40866}, {"X"=256.98886, "Y"=314.2583}, {"X"=261.16953, "Y"=235.7094}, {"X"=260.71188, "Y"=284.01248}, {"X"=264.03452, "Y"=297.1253}, {"X"=267.61978, "Y"=284.16837}, {"X"=267.2503, "Y"=318.7978}, {"X"=270.78076, "Y"=310.25726}, {"X"=265.35568, "Y"=335.9185}, {"X"=264.61105, "Y"=407.71762}, {"X"=277.39456, "Y"=465.81787}, {"X"=290.47006, "Y"=486.48096}, {"X"=297.47086, "Y"=466.2817}, {"X"=301.3043, "Y"=437.61307}, {"X"=305.61844, "Y"=478.70486}, {"X"=306.62808, "Y"=515.11456}, {"X"=303.38123, "Y"=511.01962}, {"X"=295.86334, "Y"=462.15445}, {"X"=288.39514, "Y"=399.90707}, {"X"=283.48862, "Y"=387.21454}, {"X"=275.4176, "Y"=353.209}, {"X"=273.81213, "Y"=344.65427}, {"X"=270.53854, "Y"=331.75488}, {"X"=270.78076, "Y"=310.25726}, {"X"=267.57336, "Y"=288.51984}, {"X"=258.945, "Y"=288.32504}, {"X"=239.98987, "Y"=283.54486}, {"X"=233.39322, "Y"=217.31876}, {"X"=228.00288, "Y"=257.0239}, {"X"=228.01959, "Y"=252.62599}, {"X"=236.88605, "Y"=217.39688}, {"X"=233.64648, "Y"=163.36511}, {"X"=235.45438, "Y"=154.31503}, {"X"=239.31902, "Y"=94.62417}, {"X"=244.4886, "Y"=122.47708}, {"X"=257.91956, "Y"=5.4553514}, {"X"=225.09923, "Y"=80.34515}, {"X"=214.29851, "Y"=135.58218}, {"X"=216.08466, "Y"=126.44748}, {"X"=231.90393, "Y"=158.78485}, {"X"=270.46478, "Y"=182.28154}, {"X"=286.09857, "Y"=196.13159}, {"X"=294.25888, "Y"=236.45132}, {"X"=307.42218, "Y"=280.7069}, {"X"=331.1539, "Y"=302.97626}, {"X"=365.0093, "Y"=325.31564}, {"X"=380.19647, "Y"=334.24484}, {"X"=394.77594, "Y"=360.17795}, {"X"=427.36664, "Y"=356.66888}, {"X"=449.2105, "Y"=365.66357}, {"X"=464.3707, "Y"=370.24854}, {"X"=479.30673, "Y"=379.04947}, {"X"=318.5591, "Y"=241.42241}, {"X"=319.95352, "Y"=259.09164}, {"X"=323.33548, "Y"=263.56058}, {"X"=325.8065, "Y"=311.50317}, {"X"=318.75803, "Y"=319.9654}, {"X"=328.26035, "Y"=276.8104}, {"X"=331.626, "Y"=281.25278}, {"X"=333.16312, "Y"=290.00076}, {"X"=342.82596, "Y"=246.38667}, {"X"=366.90756, "Y"=193.43904}, {"X"=388.118, "Y"=189.4098}, {"X"=400.86823, "Y"=176.14578}, {"X"=416.09125, "Y"=144.62672}, {"X"=454.63586, "Y"=113.27279}, {"X"=471.90735, "Y"=85.76598}, {"X"=476.43246, "Y"=104.486244}, {"X"=479.57532, "Y"=113.82262}, {"X"=484.91995, "Y"=113.940445}, {"X"=498.71835, "Y"=123.48362}, {"X"=488.9459, "Y"=141.65967}, {"X"=478.06577, "Y"=222.79198}, {"X"=464.05252, "Y"=262.33212}, {"X"=460.38614, "Y"=266.64432}, {"X"=458.05975, "Y"=240.12411}, {"X"=401.05698, "Y"=326.13324}, {"X"=431.1182, "Y"=348.23212}, {"X"=449.7545, "Y"=352.9205}, {"X"=299.87003, "Y"=319.53723}, {"X"=296.09848, "Y"=340.89224}, {"X"=301.444, "Y"=328.1685}, {"X"=304.94696, "Y"=323.95337}, {"X"=311.81012, "Y"=324.109}, {"X"=311.73096, "Y"=328.40192}, {"X"=308.07278, "Y"=341.16443}, {"X"=290.7139, "Y"=357.80713}, {"X"=276.546, "Y"=399.63565}, {"X"=256.12396, "Y"=411.69135}, {"X"=238.96991, "Y"=456.7453}, {"X"=235.83841, "Y"=415.38788}, {"X"=225.65697, "Y"=431.74042}, {"X"=239.11534, "Y"=432.05005}, {"X"=237.50247, "Y"=419.58194}, {"X"=247.5579, "Y"=428.10657}, {"X"=257.9276, "Y"=399.20914}, {"X"=268.40567, "Y"=370.00967}, {"X"=283.60355, "Y"=378.79932}, {"X"=295.6967, "Y"=366.4015}, {"X"=312.9653, "Y"=354.064}, {"X"=327.70898, "Y"=302.89835}, {"X"=331.24805, "Y"=298.64462}, {"X"=335.8678, "Y"=246.23047}, {"X"=336.0282, "Y"=316.04898}, {"X"=322.10544, "Y"=324.34253}, {"X"=285.36145, "Y"=374.6212}, {"X"=251.39265, "Y"=369.62143}, {"X"=236.01547, "Y"=381.92358}, {"X"=203.77826, "Y"=402.14874}, {"X"=190.14832, "Y"=363.99417}, {"X"=205.4636, "Y"=338.8319}, {"X"=210.57187, "Y"=364.46}, {"X"=212.27866, "Y"=360.2627}, {"X"=224.18895, "Y"=364.77057}, {"X"=236.2624, "Y"=335.2575}, {"X"=241.44916, "Y"=326.80698}, {"X"=248.20982, "Y"=339.80362}, {"X"=256.95062, "Y"=318.5643}, {"X"=260.26175, "Y"=331.5215}, {"X"=261.8909, "Y"=340.11462}, {"X"=255.56851, "Y"=279.53748}, {"X"=260.67065, "Y"=288.36398}, {"X"=260.96054, "Y"=257.76505}, {"X"=252.53365, "Y"=226.64485}, {"X"=230.01048, "Y"=190.38762}, {"X"=217.77554, "Y"=167.54703}, {"X"=205.44559, "Y"=126.21234}, {"X"=203.6707, "Y"=121.575516}, {"X"=194.74652, "Y"=93.64334}, {"X"=180.3864, "Y"=70.01724}, {"X"=178.72449, "Y"=97.93103}, {"X"=184.11879, "Y"=111.92761}, {"X"=189.44995, "Y"=112.04522}, {"X"=200.1218, "Y"=121.49713}, {"X"=205.44519, "Y"=121.614716}, {"X"=224.95105, "Y"=126.64343}, {"X"=258.28317, "Y"=168.44722}, {"X"=285.85406, "Y"=214.0327}, {"X"=303.11533, "Y"=227.77768}, {"X"=306.8346, "Y"=214.50174}, {"X"=324.77353, "Y"=192.49988}, {"X"=337.20895, "Y"=263.87274}, {"X"=343.93738, "Y"=272.7905}, {"X"=343.31485, "Y"=298.9174}, {"X"=338.96698, "Y"=337.59088}, {"X"=332.40137, "Y"=324.57605}, {"X"=309.70602, "Y"=345.47064}, {"X"=285.06802, "Y"=395.64365}, {"X"=280.59283, "Y"=349.07086}, {"X"=270.68365, "Y"=318.8756}, {"X"=264.12198, "Y"=288.44193}, {"X"=265.17877, "Y"=352.9759}, {"X"=260.6295, "Y"=292.70895}, {"X"=258.90515, "Y"=292.67}, {"X"=259.63208, "Y"=213.44647}, {"X"=264.38593, "Y"=262.23416}, {"X"=258.74628, "Y"=309.98474}, {"X"=258.78592, "Y"=305.6658}, {"X"=262.01642, "Y"=327.2737}, {"X"=274.01514, "Y"=327.54602}, {"X"=296.36835, "Y"=323.7588}, {"X"=325.09146, "Y"=345.8206}, {"X"=345.08878, "Y"=367.528}, {"X"=360.65018, "Y"=359.40045}, {"X"=380.1755, "Y"=277.98056}, {"X"=390.97946, "Y"=265.0826}, {"X"=373.46597, "Y"=329.80295}, {"X"=372.34576, "Y"=368.14966}, {"X"=370.88718, "Y"=359.6337}, {"X"=366.20895, "Y"=282.0327}, {"X"=370.28735, "Y"=260.22354}, {"X"=368.19916, "Y"=333.9724}, {"X"=371.50314, "Y"=338.33008}, {"X"=379.7819, "Y"=291.05334}, {"X"=384.559, "Y"=304.1841}, {"X"=389.72815, "Y"=304.30103}, {"X"=396.184, "Y"=265.1997}, {"X"=413.3678, "Y"=221.34471}, {"X"=431.71188, "Y"=199.37924}, {"X"=446.67474, "Y"=177.16435}, {"X"=453.29117, "Y"=145.4504}, {"X"=466.70007, "Y"=122.776855}, {"X"=464.92145, "Y"=122.737595}, {"X"=464.92145, "Y"=122.737595}, {"X"=464.92145, "Y"=122.737595}, {"X"=483.35385, "Y"=109.27589}, {"X"=477.37216, "Y"=123.01243}, {"X"=469.09088, "Y"=108.96163}, {"X"=470.05255, "Y"=127.45922}, {"X"=484.53766, "Y"=159.84033}, {"X"=486.99036, "Y"=182.58493}, {"X"=482.1135, "Y"=284.64667}, {"X"=473.5763, "Y"=319.16522}, {"X"=467.67758, "Y"=297.38647}, {"X"=458.47525, "Y"=310.18478}, {"X"=457.88806, "Y"=284.1003}, {"X"=453.4938, "Y"=305.74323}, {"X"=448.4214, "Y"=261.98062}, {"X"=450.19885, "Y"=177.24272}, {"X"=454.72058, "Y"=195.3964}, {"X"=445.2805, "Y"=168.0654}, {"X"=432.75336, "Y"=172.32446}, {"X"=423.19516, "Y"=239.34238}, {"X"=420.6884, "Y"=212.57892}, {"X"=421.34625, "Y"=194.65248}, {"X"=344.16455, "Y"=405.36636}, {"X"=316.46143, "Y"=349.88712}, {"X"=321.4267, "Y"=272.2834}, {"X"=316.79178, "Y"=332.8051}, {"X"=310.1723, "Y"=319.77075}, {"X"=306.51218, "Y"=332.57172}, {"X"=292.61273, "Y"=345.08188}, {"X"=273.40976, "Y"=378.56644}, {"X"=252.8156, "Y"=403.27267}, {"X"=225.70045, "Y"=419.31085}, {"X"=227.37065, "Y"=423.49884}, {"X"=207.15701, "Y"=414.72943}, {"X"=220.58887, "Y"=439.88037}, {"X"=227.35492, "Y"=427.64203}, {"X"=239.18854, "Y"=419.62067}, {"X"=257.966, "Y"=395.02313}, {"X"=275.00632, "Y"=387.02054}, {"X"=285.53854, "Y"=361.93268}, {"X"=297.3996, "Y"=366.44034}, {"X"=316.8747, "Y"=328.51865}, {"X"=323.73322, "Y"=328.67432}, {"X"=331.81586, "Y"=272.51743}, {"X"=349.0245, "Y"=277.2784}, {"X"=366.45105, "Y"=273.29767}, {"X"=398.19925, "Y"=308.82074}, {"X"=418.86288, "Y"=309.28836}, {"X"=416.20822, "Y"=287.52133}, {"X"=426.24762, "Y"=296.45053}, {"X"=414.47968, "Y"=287.48233}, {"X"=378.18475, "Y"=286.66333}, {"X"=361.72598, "Y"=255.63101}, {"X"=356.17322, "Y"=268.6861}, {"X"=349.56647, "Y"=255.35773}, {"X"=339.2457, "Y"=250.71938}, {"X"=325.0696, "Y"=263.59958}, {"X"=316.5665, "Y"=254.61606}, {"X"=314.66513, "Y"=263.36548}, {"X"=278.3093, "Y"=258.15518}, {"X"=255.75629, "Y"=257.648}, {"X"=222.73611, "Y"=278.797}, {"X"=193.37465, "Y"=282.49298}, {"X"=151.90904, "Y"=277.19968}, {"X"=145.00067, "Y"=277.04385}, {"X"=138.09259, "Y"=276.88806}, {"X"=124.583885, "Y"=298.30423}, {"X"=123.78886, "Y"=362.48068}, {"X"=141.83652, "Y"=303.01926}, {"X"=145.04657, "Y"=281.4024}, {"X"=179.58507, "Y"=286.5332}, {"X"=205.45921, "Y"=287.1174}, {"X"=229.62982, "Y"=283.3111}, {"X"=263.73047, "Y"=327.31262}, {"X"=287.30313, "Y"=357.72943}, {"X"=295.63007, "Y"=370.63095}, {"X"=348.19116, "Y"=446.9399}, {"X"=402.33704, "Y"=485.01056}, {"X"=429.9022, "Y"=505.90002}, {"X"=458.74774, "Y"=530.68024}, {"X"=474.34515, "Y"=550.97754}, {"X"=498.86234, "Y"=587.075}, {"X"=531.23285, "Y"=649.88043}, {"X"=531.23285, "Y"=649.88043}, {"X"=425.7513, "Y"=309.44424}, {"X"=426.1506, "Y"=343.84857}, {"X"=404.0677, "Y"=435.84497}, {"X"=402.62338, "Y"=476.87604}, {"X"=395.93658, "Y"=476.72137}, {"X"=389.93048, "Y"=351.55908}, {"X"=395.3548, "Y"=393.9739}, {"X"=389.38382, "Y"=472.4905}, {"X"=375.19336, "Y"=443.44104}, {"X"=375.81613, "Y"=422.7589}, {"X"=374.005, "Y"=426.86874}, {"X"=357.47827, "Y"=414.0169}, {"X"=335.99216, "Y"=392.61554}, {"X"=319.2028, "Y"=383.82507}, {"X"=302.009, "Y"=396.03152}, {"X"=293.60306, "Y"=391.64557}, {"X"=278.45285, "Y"=382.89362}, {"X"=285.47943, "Y"=366.16846}, {"X"=308.40726, "Y"=417.05383}, {"X"=346.71768, "Y"=438.65842}, {"X"=367.99323, "Y"=459.72308}, {"X"=383.08032, "Y"=460.0713}, {"X"=382.30646, "Y"=431.205}, {"X"=392.41693, "Y"=431.43747}, {"X"=398.73257, "Y"=443.98315}, {"X"=401.95187, "Y"=448.1787}, {"X"=393.13916, "Y"=460.30344}, {"X"=383.33972, "Y"=451.865}, {"X"=372.22223, "Y"=372.37878}, {"X"=362.00793, "Y"=372.1457}, {"X"=352.22864, "Y"=354.958}, {"X"=340.77994, "Y"=333.34982}, {"X"=334.79248, "Y"=294.38443}, {"X"=352.818, "Y"=264.22394}, {"X"=364.5993, "Y"=277.62946}, {"X"=390.0805, "Y"=238.59987}, {"X"=392.67468, "Y"=211.953}, {"X"=376.0102, "Y"=242.71135}, {"X"=415.2616, "Y"=313.5287}, {"X"=385.09747, "Y"=286.8193}, {"X"=386.59512, "Y"=238.52171}, {"X"=384.58093, "Y"=247.324}, {"X"=375.3669, "Y"=264.73132}, {"X"=364.5993, "Y"=277.62946}, {"X"=353.15204, "Y"=251.03174}, {"X"=352.525, "Y"=206.58185}, {"X"=337.8074, "Y"=237.42778}, {"X"=229.4352, "Y"=330.82156}, {"X"=232.73997, "Y"=356.48636}, {"X"=225.89116, "Y"=364.8094}, {"X"=220.58887, "Y"=439.88037}, {"X"=222.29254, "Y"=431.66302}, {"X"=237.85452, "Y"=356.60287}, {"X"=242.69589, "Y"=398.86023}, {"X"=247.5885, "Y"=423.9635}, {"X"=254.43526, "Y"=411.6526}, {"X"=254.43526, "Y"=411.6526}, {"X"=266.83987, "Y"=357.26324}, {"X"=285.47943, "Y"=366.16846}, {"X"=295.63007, "Y"=370.63095}, {"X"=309.3975, "Y"=362.47653}, {"X"=321.8452, "Y"=337.20187}, {"X"=334.2134, "Y"=320.31573}, {"X"=344.93423, "Y"=303.28793}, {"X"=364.12173, "Y"=295.047}, {"X"=374.6533, "Y"=229.37984}, {"X"=379.4644, "Y"=184.70822}, {"X"=382.30536, "Y"=207.24683}, {"X"=381.5006, "Y"=233.97371}, {"X"=370.66147, "Y"=247.01154}, {"X"=374.7285, "Y"=286.58533}, {"X"=368.42847, "Y"=264.5752}, {"X"=353.6585, "Y"=299.15118}, {"X"=335.9308, "Y"=320.35468}, {"X"=327.80054, "Y"=298.56668}, {"X"=329.61728, "Y"=294.2675}, {"X"=318.67358, "Y"=324.26468}, {"X"=329.2092, "Y"=392.46033}, {"X"=351.76434, "Y"=438.7746}, {"X"=372.90005, "Y"=463.93335}, {"X"=376.87463, "Y"=443.47974}, {"X"=384.12244, "Y"=427.10126}, {"X"=386.82993, "Y"=447.83026}, {"X"=381.5323, "Y"=455.93243}, {"X"=373.02213, "Y"=459.83914}, {"X"=355.45798, "Y"=426.4425}, {"X"=337.88312, "Y"=384.25208}, {"X"=326.44165, "Y"=362.86505}, {"X"=318.0861, "Y"=354.18057}, {"X"=301.444, "Y"=328.1685}, {"X"=290.0091, "Y"=289.02643}, {"X"=288.22122, "Y"=293.3323}, {"X"=284.59448, "Y"=306.24988}, {"X"=275.8862, "Y"=314.68643}, {"X"=256.87436, "Y"=327.157}, {"X"=236.3532, "Y"=318.0974}, {"X"=227.69028, "Y"=339.3372}, {"X"=214.02402, "Y"=330.47162}, {"X"=190.14832, "Y"=363.99417}, {"X"=162.98457, "Y"=371.82697}, {"X"=164.68364, "Y"=371.86575}, {"X"=294.71912, "Y"=319.42047}, {"X"=296.03125, "Y"=345.15964}, {"X"=298.639, "Y"=289.22125}, {"X"=303.67, "Y"=298.02124}, {"X"=308.2254, "Y"=332.61063}, {"X"=310.0943, "Y"=324.0701}, {"X"=310.01642, "Y"=328.363}, {"X"=303.0858, "Y"=332.4939}, {"X"=298.56927, "Y"=293.56607}, {"X"=290.39053, "Y"=262.81927}, {"X"=266.76334, "Y"=200.187}, {"X"=259.8788, "Y"=186.55307}, {"X"=240.64331, "Y"=172.58296}, {"X"=230.12149, "Y"=163.28682}, {"X"=208.98482, "Y"=140.04099}, {"X"=184.20311, "Y"=134.91621}, {"X"=169.95903, "Y"=120.83091}, {"X"=175.1862, "Y"=102.48612}, {"X"=166.288, "Y"=102.29007}, {"X"=157.39026, "Y"=102.094025}, {"X"=171.6801, "Y"=111.65321}, {"X"=116.881676, "Y"=128.84428}, {"X"=316.9871, "Y"=232.52802}, {"X"=318.1332, "Y"=263.4435}, {"X"=310.87967, "Y"=280.78488}, {"X"=318.5051, "Y"=332.84402}, {"X"=323.5573, "Y"=337.24078}, {"X"=330.77878, "Y"=320.23788}, {"X"=338.96698, "Y"=337.59088}, {"X"=340.37805, "Y"=350.4314}, {"X"=348.81918, "Y"=422.13882}, {"X"=371.8309, "Y"=443.3636}, {"X"=376.62436, "Y"=451.71017}, {"X"=387.0954, "Y"=439.58786}, {"X"=378.3919, "Y"=393.58575}, {"X"=384.4957, "Y"=468.2923}, {"X"=380.1095, "Y"=447.6754}, {"X"=361.8582, "Y"=439.00693}, {"X"=349.02975, "Y"=413.82306}, {"X"=333.35452, "Y"=358.7786}, {"X"=321.50003, "Y"=354.25833}, {"X"=310.01642, "Y"=328.363}, {"X"=292.7422, "Y"=336.54068}, {"X"=276.14926, "Y"=293.05957}, {"X"=260.71188, "Y"=284.01248}, {"X"=245.08168, "Y"=296.6969}, {"X"=236.81549, "Y"=230.73145}, {"X"=226.29926, "Y"=248.18242}, {"X"=219.36134, "Y"=243.61507}, {"X"=219.36134, "Y"=243.61507}, {"X"=229.86403, "Y"=226.13715}, {"X"=243.55669, "Y"=266.15067}, {"X"=271.07385, "Y"=284.2463}, {"X"=294.91904, "Y"=306.48352}, {"X"=316.066, "Y"=280.90186}, {"X"=331.1539, "Y"=302.97626}, {"X"=364.6529, "Y"=338.17444}, {"X"=391.63943, "Y"=351.59796}, {"X"=403.7501, "Y"=347.60965}, {"X"=414.94794, "Y"=322.14584}, {"X"=422.20892, "Y"=265.7853}, {"X"=423.6147, "Y"=274.58536}, {"X"=425.34723, "Y"=274.6244}, {"X"=415.4106, "Y"=356.39667}, {"X"=408.57898, "Y"=356.2411}, {"X"=400.1845, "Y"=351.79242}, {"X"=391.4512, "Y"=304.34}, {"X"=389.1061, "Y"=269.42755}, {"X"=384.1573, "Y"=317.13937}, {"X"=385.60703, "Y"=325.7828}, {"X"=390.89532, "Y"=321.60062}, {"X"=392.05554, "Y"=338.797}, {"X"=396.62433, "Y"=355.9689}, {"X"=411.883, "Y"=452.52307}, {"X"=436.05563, "Y"=518.12354}, {"X"=456.75504, "Y"=574.2983}, {"X"=431.16522, "Y"=635.99243}, {"X"=441.03928, "Y"=670.65015}, {"X"=467.2407, "Y"=663.6583}, {"X"=452.83478, "Y"=514.4923}, {"X"=446.36374, "Y"=510.31497}, {"X"=431.5657, "Y"=505.93863}, {"X"=412.3531, "Y"=485.24246}, {"X"=394.10208, "Y"=431.4762}, {"X"=385.1498, "Y"=447.79153}, {"X"=374.005, "Y"=426.86874}, {"X"=356.0097, "Y"=405.63788}, {"X"=345.5035, "Y"=350.54803}, {"X"=336.0884, "Y"=388.4175}, {"X"=331.55524, "Y"=362.98163}, {"X"=319.43808, "Y"=285.33768}, {"X"=312.4478, "Y"=289.53305}, {"X"=308.45523, "Y"=319.73184}, {"X"=305.39352, "Y"=298.06018}, {"X"=295.32156, "Y"=280.434}, {"X"=278.03647, "Y"=280.0442}, {"X"=281.8942, "Y"=249.43117}, {"X"=282.12518, "Y"=231.7468}, {"X"=271.9188, "Y"=209.25494}, {"X"=261.46475, "Y"=204.54848}, {"X"=269.8281, "Y"=240.32912}, {"X"=275.36478, "Y"=213.79819}, {"X"=288.84488, "Y"=249.5873}, {"X"=307.57544, "Y"=271.97137}, {"X"=316.1491, "Y"=276.5374}, {"X"=323.0697, "Y"=276.6934}, {"X"=331.12424, "Y"=223.95834}, {"X"=334.98666, "Y"=285.68854}, {"X"=338.6421, "Y"=277.0444}, {"X"=347.08102, "Y"=285.96146}, {"X"=368.06055, "Y"=277.7075}, {"X"=382.30566, "Y"=264.88745}, {"X"=398.3676, "Y"=198.63556}, {"X"=409.60123, "Y"=278.6438}, {"X"=428.98083, "Y"=270.3253}, {"X"=440.4483, "Y"=244.15704}, {"X"=442.36978, "Y"=239.77232}, {"X"=429.3186, "Y"=261.55103}, {"X"=399.8004, "Y"=260.88724}, {"X"=388.75458, "Y"=225.24828}, {"X"=381.23398, "Y"=242.82855}, {"X"=369.54227, "Y"=224.81825}, {"X"=351.52408, "Y"=246.58194}, {"X"=337.5075, "Y"=250.68033}, {"X"=329.7104, "Y"=289.92282}, {"X"=313.849, "Y"=306.9119}, {"X"=288.15936, "Y"=297.67062}, {"X"=261.68298, "Y"=361.3889}, {"X"=246.16968, "Y"=386.36102}, {"X"=218.91867, "Y"=435.71667}, {"X"=200.41322, "Y"=418.73}, {"X"=193.58879, "Y"=380.95383}, {"X"=202.079, "Y"=389.55124}, {"X"=208.85042, "Y"=402.26498}, {"X"=213.95819, "Y"=377.20825}, {"X"=222.53604, "Y"=347.74963}, {"X"=225.98042, "Y"=339.2983}, {"X"=244.96437, "Y"=313.98587}, {"X"=258.74628, "Y"=309.98474}, {"X"=265.66782, "Y"=305.82156}, {"X"=265.8928, "Y"=284.1294}, {"X"=260.46542, "Y"=310.02368}, {"X"=236.55951, "Y"=279.10876}, {"X"=226.19186, "Y"=278.87494}, {"X"=215.86972, "Y"=252.35294}, {"X"=215.87724, "Y"=247.94832}, {"X"=205.4555, "Y"=243.3029}, {"X"=200.21938, "Y"=221.02834}, {"X"=200.21938, "Y"=221.02834}, {"X"=423.2134, "Y"=330.9319}, {"X"=416.80447, "Y"=364.9249}] {"Y" format="%.2f"; "X" format="%.2f"}
  in  "manual top ChenJin vs DuPengYu":T1[](array[typedef])=[{"X"=281.66464, "Y"=267.00864}, {"X"=284.9503, "Y"=280.2001}, {"X"=291.5417, "Y"=302.08032}, {"X"=283.22183, "Y"=280.16113}, {"X"=290.32672, "Y"=267.20364}, {"X"=279.8764, "Y"=271.3474}, {"X"=290.263, "Y"=271.5814}, {"X"=291.8644, "Y"=280.35605}, {"X"=307.3457, "Y"=285.0648}, {"X"=321.51398, "Y"=267.9058}, {"X"=328.35272, "Y"=272.43942}, {"X"=328.35272, "Y"=272.43942}, {"X"=326.98685, "Y"=254.85025}, {"X"=324.05014, "Y"=228.24654}, {"X"=322.39407, "Y"=223.76294}, {"X"=317.92368, "Y"=183.33813}, {"X"=291.75336, "Y"=169.19102}, {"X"=267.5163, "Y"=127.584175}, {"X"=249.81342, "Y"=122.594696}, {"X"=228.58533, "Y"=103.66264}, {"X"=223.23123, "Y"=108.17115}, {"X"=217.89487, "Y"=108.0535}, {"X"=210.77998, "Y"=107.896645}, {"X"=219.70566, "Y"=94.19257}, {"X"=246.3888, "Y"=104.0549}, {"X"=274.55844, "Y"=132.33127}, {"X"=295.3456, "Y"=164.73543}, {"X"=304.2372, "Y"=160.39035}, {"X"=312.6498, "Y"=183.22072}, {"X"=317.75223, "Y"=192.34337}, {"X"=326.06906, "Y"=214.93175}, {"X"=334.42072, "Y"=232.9187}, {"X"=341.0864, "Y"=246.34763}, {"X"=337.10974, "Y"=268.2569}, {"X"=339.66602, "Y"=307.49612}, {"X"=356.87958, "Y"=307.88568}, {"X"=382.43713, "Y"=372.6119}, {"X"=388.70465, "Y"=389.62085}, {"X"=385.70877, "Y"=376.91238}, {"X"=372.7175, "Y"=355.42453}, {"X"=368.07797, "Y"=338.25226}, {"X"=366.36545, "Y"=338.21335}, {"X"=347.63434, "Y"=333.50546}, {"X"=341.08295, "Y"=320.47147}, {"X"=317.20752, "Y"=311.30847}, {"X"=296.7762, "Y"=297.86542}, {"X"=295.0528, "Y"=297.82645}, {"X"=286.43604, "Y"=297.63168}, {"X"=276.25507, "Y"=284.36322}, {"X"=274.68332, "Y"=271.23044}, {"X"=276.30807, "Y"=280.0052}, {"X"=269.0142, "Y"=314.53073}, {"X"=248.27298, "Y"=331.2493}, {"X"=244.76077, "Y"=343.9935}, {"X"=224.20251, "Y"=360.53452}, {"X"=207.16687, "Y"=368.61218}, {"X"=205.46503, "Y"=355.86496}, {"X"=215.71442, "Y"=343.33286}, {"X"=224.22969, "Y"=352.0435}, {"X"=232.98128, "Y"=305.08185}, {"X"=243.21873, "Y"=318.25302}, {"X"=251.8354, "Y"=314.14154}, {"X"=246.74326, "Y"=305.39328}, {"X"=239.9131, "Y"=296.58005}, {"X"=246.83531, "Y"=292.39734}, {"X"=227.8537, "Y"=296.30746}, {"X"=233.06267, "Y"=287.74066}, {"X"=219.35118, "Y"=248.02635}, {"X"=219.31067, "Y"=265.6048}, {"X"=222.77417, "Y"=265.68277}, {"X"=238.45908, "Y"=248.45555}, {"X"=254.09444, "Y"=248.80675}, {"X"=259.30655, "Y"=248.92381}, {"X"=280.04425, "Y"=258.19418}, {"X"=283.22183, "Y"=280.16113}, {"X"=283.4556, "Y"=262.66324}, {"X"=278.52902, "Y"=240.52432}, {"X"=268.46762, "Y"=204.70485}, {"X"=258.24298, "Y"=172.97432}, {"X"=247.77931, "Y"=159.13722}, {"X"=244.3696, "Y"=140.82448}, {"X"=251.55307, "Y"=127.23137}, {"X"=250.15575, "Y"=76.22524}, {"X"=239.44933, "Y"=71.31285}, {"X"=228.69131, "Y"=75.754105}, {"X"=210.83305, "Y"=42.469032}, {"X"=198.23993, "Y"=37.46549}, {"X"=207.23665, "Y"=42.39044}, {"X"=216.15573, "Y"=84.81122}, {"X"=214.37007, "Y"=84.77197}, {"X"=226.82129, "Y"=98.990074}, {"X"=239.13828, "Y"=126.95699}, {"X"=265.32898, "Y"=168.6038}, {"X"=280.8951, "Y"=191.52184}, {"X"=291.16394, "Y"=209.68494}, {"X"=282.12518, "Y"=231.7468}, {"X"=287.60236, "Y"=214.07178}, {"X"=284.64597, "Y"=173.56142}, {"X"=279.93317, "Y"=127.858604}, {"X"=280.04785, "Y"=118.65673}, {"X"=278.49612, "Y"=100.1279}, {"X"=287.6613, "Y"=81.71925}, {"X"=271.77704, "Y"=62.644356}, {"X"=261.14746, "Y"=48.290337}, {"X"=250.36372, "Y"=48.05454}, {"X"=218.0261, "Y"=42.626217}, {"X"=218.00717, "Y"=52.060837}, {"X"=234.30054, "Y"=24.02175}, {"X"=232.26852, "Y"=75.83262}, {"X"=242.82794, "Y"=103.97645}, {"X"=256.63864, "Y"=154.78496}, {"X"=284.64597, "Y"=173.56142}, {"X"=289.2236, "Y"=223.0205}, {"X"=282.0673, "Y"=236.17796}, {"X"=260.71188, "Y"=284.01248}, {"X"=246.7739, "Y"=301.0678}, {"X"=220.90678, "Y"=317.74725}, {"X"=226.04039, "Y"=322.16367}, {"X"=227.82082, "Y"=304.9651}, {"X"=222.66052, "Y"=304.8483}, {"X"=241.58238, "Y"=305.2765}, {"X"=253.69633, "Y"=296.89163}, {"X"=255.38216, "Y"=301.2625}, {"X"=272.8009, "Y"=284.28528}, {"X"=300.50745, "Y"=280.55096}, {"X"=310.72165, "Y"=289.49408}, {"X"=317.87924, "Y"=276.57642}, {"X"=332.00626, "Y"=263.75568}, {"X"=351.0836, "Y"=264.18494}, {"X"=356.17322, "Y"=268.6861}, {"X"=366.69388, "Y"=264.53616}, {"X"=377.4909, "Y"=251.57843}, {"X"=389.0335, "Y"=216.33942}, {"X"=411.61954, "Y"=221.3056}, {"X"=424.7719, "Y"=243.80534}, {"X"=435.74628, "Y"=230.74808}, {"X"=445.20422, "Y"=213.12668}, {"X"=467.5725, "Y"=222.55725}, {"X"=422.6325, "Y"=300.7103}, {"X"=426.08194, "Y"=300.78827}, {"X"=423.2134, "Y"=330.9319}, {"X"=423.62628, "Y"=365.08038}, {"X"=425.00595, "Y"=373.5833}, {"X"=424.51904, "Y"=386.23236}, {"X"=424.19562, "Y"=394.63388}, {"X"=419.8528, "Y"=419.6123}, {"X"=412.3194, "Y"=394.36212}, {"X"=401.02124, "Y"=377.262}, {"X"=391.77792, "Y"=347.33734}, {"X"=385.87643, "Y"=317.1783}, {"X"=380.98148, "Y"=308.4311}, {"X"=380.0441, "Y"=282.34473}, {"X"=368.30563, "Y"=268.95926}, {"X"=344.25073, "Y"=259.63806}, {"X"=327.26254, "Y"=241.61768}, {"X"=321.60138, "Y"=263.52155}, {"X"=308.03806, "Y"=245.60574}, {"X"=306.07095, "Y"=258.77948}, {"X"=304.4849, "Y"=249.9386}, {"X"=234.74467, "Y"=296.46323}, {"X"=236.42166, "Y"=305.1597}, {"X"=239.68488, "Y"=335.33527}, {"X"=219.08241, "Y"=364.65408}, {"X"=227.54527, "Y"=377.51865}, {"X"=219.03383, "Y"=385.74045}, {"X"=215.61354, "Y"=402.41998}, {"X"=215.62068, "Y"=398.24}, {"X"=224.10803, "Y"=390.05533}, {"X"=222.42557, "Y"=385.818}, {"X"=220.77357, "Y"=368.9227}, {"X"=229.40015, "Y"=339.37604}, {"X"=229.45274, "Y"=326.53473}, {"X"=236.3532, "Y"=318.0974}, {"X"=241.55565, "Y"=309.59552}, {"X"=246.68211, "Y"=314.02478}, {"X"=248.43169, "Y"=309.7512}, {"X"=243.24666, "Y"=313.94696}, {"X"=239.96423, "Y"=287.89648}, {"X"=231.39479, "Y"=274.62708}, {"X"=229.66554, "Y"=274.5881}, {"X"=231.45251, "Y"=261.49313}, {"X"=226.22243, "Y"=270.13876}, {"X"=238.3119, "Y"=274.783}, {"X"=252.11217, "Y"=279.4595}, {"X"=260.71188, "Y"=284.01248}, {"X"=264.29767, "Y"=270.99646}, {"X"=267.6663, "Y"=279.8103}, {"X"=267.71286, "Y"=275.44568}, {"X"=271.07385, "Y"=284.2463}, {"X"=271.0248, "Y"=288.59778}, {"X"=260.67065, "Y"=288.36398}, {"X"=250.25043, "Y"=296.81372}, {"X"=246.59073, "Y"=326.92365}, {"X"=266.74942, "Y"=365.74127}, {"X"=281.5125, "Y"=408.10522}, {"X"=284.48764, "Y"=437.22598}, {"X"=296.0608, "Y"=449.85275}, {"X"=296.1268, "Y"=445.7402}, {"X"=304.59546, "Y"=441.8151}, {"X"=301.3043, "Y"=437.61307}, {"X"=294.83826, "Y"=420.8989}, {"X"=283.54605, "Y"=383.01004}, {"X"=272.0046, "Y"=353.13132}, {"X"=270.39407, "Y"=344.5765}, {"X"=268.6383, "Y"=348.7988}, {"X"=265.53363, "Y"=318.75888}, {"X"=272.60004, "Y"=301.65192}, {"X"=264.1658, "Y"=284.09042}, {"X"=253.80426, "Y"=283.8566}, {"X"=240.19627, "Y"=248.49457}, {"X"=231.64684, "Y"=217.2797}, {"X"=226.43903, "Y"=208.23878}, {"X"=230.17738, "Y"=149.64243}, {"X"=237.17154, "Y"=163.4434}, {"X"=235.6143, "Y"=122.281075}, {"X"=232.14586, "Y"=103.7411}, {"X"=233.90445, "Y"=108.406456}, {"X"=235.66032, "Y"=113.06463}, {"X"=232.20705, "Y"=89.81945}, {"X"=224.99527, "Y"=112.82935}, {"X"=221.47652, "Y"=98.87238}, {"X"=219.61002, "Y"=135.6997}, {"X"=226.77274, "Y"=112.86856}, {"X"=240.9931, "Y"=113.18227}, {"X"=264.0137, "Y"=122.90834}, {"X"=270.86295, "Y"=145.98126}, {"X"=292.71494, "Y"=223.09865}, {"X"=306.68094, "Y"=223.41124}, {"X"=335.67096, "Y"=255.04543}, {"X"=353.32608, "Y"=312.1263}, {"X"=382.57056, "Y"=312.78848}, {"X"=393.17432, "Y"=304.37897}, {"X"=432.4909, "Y"=356.78558}, {"X"=454.5127, "Y"=361.53888}, {"X"=466.85098, "Y"=353.30957}, {"X"=325.0696, "Y"=263.59958}, {"X"=323.24677, "Y"=267.9448}, {"X"=225.19228, "Y"=997.0872}, {"X"=328.44525, "Y"=268.06183}, {"X"=326.98685, "Y"=254.85025}, {"X"=321.2525, "Y"=281.01883}, {"X"=321.16562, "Y"=285.37665}, {"X"=319.69522, "Y"=272.2444}, {"X"=324.23016, "Y"=219.35074}, {"X"=344.7212, "Y"=165.83203}, {"X"=375.62, "Y"=134.56622}, {"X"=393.79224, "Y"=121.1675}, {"X"=415.77863, "Y"=103.15071}, {"X"=437.54367, "Y"=94.33509}, {"X"=468.73795, "Y"=76.34253}, {"X"=483.7858, "Y"=100.00371}, {"X"=493.386, "Y"=86.23774}, {"X"=499.62943, "Y"=104.99702}, {"X"=507.23636, "Y"=95.86773}, {"X"=496.28632, "Y"=100.27878}, {"X"=480.2914, "Y"=136.881}, {"X"=475.07635, "Y"=173.26501}, {"X"=460.5774, "Y"=222.40077}, {"X"=448.97348, "Y"=248.76953}, {"X"=450.90005, "Y"=244.39154}, {"X"=448.87042, "Y"=292.61328}, {"X"=451.58548, "Y"=310.02887}, {"X"=289.81964, "Y"=302.04138}, {"X"=296.30075, "Y"=328.05176}, {"X"=291.5417, "Y"=302.08032}, {"X"=300.15225, "Y"=302.2751}, {"X"=303.96478, "Y"=280.62894}, {"X"=312.28766, "Y"=298.21603}, {"X"=315.81744, "Y"=293.95575}, {"X"=310.8006, "Y"=285.14276}, {"X"=291.4133, "Y"=310.72443}, {"X"=277.0712, "Y"=357.49634}, {"X"=261.3945, "Y"=390.90854}, {"X"=239.1641, "Y"=423.7699}, {"X"=229.05537, "Y"=423.53757}, {"X"=223.93513, "Y"=444.0767}, {"X"=223.96152, "Y"=435.83276}, {"X"=225.67145, "Y"=427.6033}, {"X"=237.66579, "Y"=390.36557}, {"X"=264.95914, "Y"=374.15533}, {"X"=278.99384, "Y"=340.50342}, {"X"=291.15765, "Y"=327.93503}, {"X"=301.51547, "Y"=323.87552}, {"X"=322.80515, "Y"=289.7669}, {"X"=340.0688, "Y"=290.15668}, {"X"=340.2711, "Y"=281.44772}, {"X"=342.20566, "Y"=272.7515}, {"X"=343.72925, "Y"=281.52573}, {"X"=311.2768, "Y"=258.89655}, {"X"=275.93866, "Y"=310.37402}, {"X"=239.83669, "Y"=309.55658}, {"X"=222.53604, "Y"=347.74963}, {"X"=207.16869, "Y"=360.1462}, {"X"=207.16869, "Y"=360.1462}, {"X"=207.16687, "Y"=368.61218}, {"X"=220.8177, "Y"=351.9658}, {"X"=229.33037, "Y"=356.40866}, {"X"=248.33632, "Y"=322.66937}, {"X"=248.33632, "Y"=322.66937}, {"X"=250.01854, "Y"=327.00143}, {"X"=255.30801, "Y"=309.9069}, {"X"=253.58891, "Y"=309.86798}, {"X"=267.2503, "Y"=318.7978}, {"X"=265.80258, "Y"=292.82584}, {"X"=259.22577, "Y"=257.726}, {"X"=271.8685, "Y"=213.72003}, {"X"=272.1715, "Y"=186.82692}, {"X"=253.10774, "Y"=154.70663}, {"X"=235.59135, "Y"=126.8786}, {"X"=214.35043, "Y"=98.71548}, {"X"=194.70277, "Y"=70.33128}, {"X"=191.14668, "Y"=79.59943}, {"X"=183.87921, "Y"=46.600765}, {"X"=174.89682, "Y"=46.404354}, {"X"=173.22865, "Y"=69.86023}, {"X"=180.44614, "Y"=84.02641}, {"X"=182.21295, "Y"=79.40321}, {"X"=189.37282, "Y"=84.222595}, {"X"=205.44284, "Y"=93.878716}, {"X"=228.58533, "Y"=103.66264}, {"X"=277.99203, "Y"=141.56894}, {"X"=300.20023, "Y"=191.95215}, {"X"=310.8115, "Y"=187.68768}, {"X"=323.46808, "Y"=169.89583}, {"X"=335.00958, "Y"=206.19072}, {"X"=346.83966, "Y"=224.3101}, {"X"=355.00342, "Y"=246.66003}, {"X"=355.8333, "Y"=281.7987}, {"X"=354.66492, "Y"=259.87222}, {"X"=328.35272, "Y"=272.43942}, {"X"=301.94653, "Y"=297.98227}, {"X"=287.66788, "Y"=332.14383}, {"X"=265.2671, "Y"=344.4599}, {"X"=256.68466, "Y"=348.52676}, {"X"=265.2671, "Y"=344.4599}, {"X"=258.50974, "Y"=335.76294}, {"X"=260.4246, "Y"=314.33615}, {"X"=258.945, "Y"=288.32504}, {"X"=263.99088, "Y"=301.4572}, {"X"=265.7576, "Y"=297.16425}, {"X"=264.1658, "Y"=284.09042}, {"X"=253.84033, "Y"=279.4985}, {"X"=262.4814, "Y"=279.69336}, {"X"=278.14536, "Y"=271.3084}, {"X"=293.65912, "Y"=276.0305}, {"X"=323.15817, "Y"=272.32242}, {"X"=339.76648, "Y"=303.17105}, {"X"=344.8299, "Y"=307.61298}, {"X"=358.25797, "Y"=320.86078}, {"X"=370.28152, "Y"=321.13333}, {"X"=369.05255, "Y"=303.8334}, {"X"=365.60687, "Y"=303.75546}, {"X"=358.94562, "Y"=294.93005}, {"X"=360.7875, "Y"=290.62448}, {"X"=354.3279, "Y"=273.02457}, {"X"=368.06055, "Y"=277.7075}, {"X"=376.5852, "Y"=282.26672}, {"X"=368.06055, "Y"=277.7075}, {"X"=381.7736, "Y"=282.38373}, {"X"=385.1248, "Y"=229.61436}, {"X"=400.1224, "Y"=198.6747}, {"X"=422.50726, "Y"=163.01549}, {"X"=434.157, "Y"=135.86075}, {"X"=460.77136, "Y"=94.8459}, {"X"=468.73795, "Y"=76.34253}, {"X"=468.73795, "Y"=76.34253}, {"X"=483.73016, "Y"=62.585087}, {"X"=486.66428, "Y"=76.735756}, {"X"=494.06052, "Y"=72.20976}, {"X"=486.88382, "Y"=72.05244}, {"X"=483.94797, "Y"=57.8797}, {"X"=489.3637, "Y"=95.474686}, {"X"=480.85645, "Y"=85.96254}, {"X"=492.49155, "Y"=104.83985}, {"X"=478.51678, "Y"=136.84175}, {"X"=479.7359, "Y"=186.94058}, {"X"=470.6665, "Y"=231.53015}, {"X"=467.13074, "Y"=271.18417}, {"X"=459.80984, "Y"=279.77548}, {"X"=447.68915, "Y"=279.5023}, {"X"=460.19376, "Y"=271.02798}, {"X"=463.09457, "Y"=244.66513}, {"X"=455.40503, "Y"=301.4511}, {"X"=463.46747, "Y"=275.48312}, {"X"=437.84518, "Y"=221.89226}, {"X"=433.30817, "Y"=248.41786}, {"X"=431.36685, "Y"=208.34236}, {"X"=431.0229, "Y"=217.27814}, {"X"=424.19043, "Y"=212.65717}, {"X"=320.90576, "Y"=298.41083}, {"X"=312.4478, "Y"=289.53305}, {"X"=321.2525, "Y"=281.01883}, {"X"=311.03815, "Y"=272.04938}, {"X"=298.98926, "Y"=267.39868}, {"X"=300.79352, "Y"=263.05338}, {"X"=284.9503, "Y"=280.2001}, {"X"=256.95062, "Y"=318.5643}, {"X"=244.53067, "Y"=377.90668}, {"X"=224.08122, "Y"=398.4338}, {"X"=217.31276, "Y"=398.27875}, {"X"=205.47107, "Y"=427.13882}, {"X"=208.84401, "Y"=414.76816}, {"X"=222.36484, "Y"=406.7488}, {"X"=237.83081, "Y"=360.84515}, {"X"=277.39008, "Y"=331.91046}, {"X"=289.4433, "Y"=327.89615}, {"X"=300.01093, "Y"=310.9191}, {"X"=312.20776, "Y"=302.54773}, {"X"=331.43674, "Y"=289.9618}, {"X"=331.43674, "Y"=289.9618}, {"X"=349.13257, "Y"=272.90753}, {"X"=351.3035, "Y"=255.39676}, {"X"=370.9118, "Y"=238.17006}, {"X"=403.4224, "Y"=256.5681}, {"X"=429.48788, "Y"=257.15393}, {"X"=436.61414, "Y"=252.90643}, {"X"=429.48788, "Y"=257.15393}, {"X"=403.7221, "Y"=247.75371}, {"X"=382.57288, "Y"=256.09955}, {"X"=363.82196, "Y"=242.43791}, {"X"=358.48288, "Y"=246.73814}, {"X"=346.30515, "Y"=246.46478}, {"X"=341.189, "Y"=241.93013}, {"X"=327.6321, "Y"=223.88019}, {"X"=318.90213, "Y"=223.68478}, {"X"=311.9185, "Y"=223.52847}, {"X"=306.60428, "Y"=227.85582}, {"X"=266.6242, "Y"=213.60278}, {"X"=212.43286, "Y"=221.3017}, {"X"=175.93216, "Y"=247.05109}, {"X"=144.7238, "Y"=250.75395}, {"X"=134.20609, "Y"=241.70346}, {"X"=118.6362, "Y"=245.76413}, {"X"=120.30727, "Y"=241.39145}, {"X"=120.24228, "Y"=236.9731}, {"X"=125.39703, "Y"=232.66505}, {"X"=151.53995, "Y"=237.67526}, {"X"=196.72998, "Y"=220.95023}, {"X"=210.68082, "Y"=230.14578}, {"X"=222.90227, "Y"=221.53604}, {"X"=243.52829, "Y"=270.5286}, {"X"=263.99088, "Y"=301.4572}, {"X"=291.2214, "Y"=323.64206}, {"X"=347.96808, "Y"=388.68918}, {"X"=393.51968, "Y"=398.12668}, {"X"=433.3804, "Y"=461.2322}, {"X"=460.0324, "Y"=502.56055}, {"X"=482.7414, "Y"=515.18726}, {"X"=492.29657, "Y"=523.4469}, {"X"=521.71, "Y"=532.14624}, {"X"=433.66608, "Y"=283.55405}, {"X"=433.83798, "Y"=279.1901}, {"X"=421.9826, "Y"=317.99634}, {"X"=421.60007, "Y"=373.50558}, {"X"=417.72247, "Y"=386.07703}, {"X"=412.6252, "Y"=385.9605}, {"X"=408.77628, "Y"=398.47598}, {"X"=401.706, "Y"=406.6852}, {"X"=390.95004, "Y"=372.80615}, {"X"=382.30618, "Y"=376.8347}, {"X"=365.2943, "Y"=376.44626}, {"X"=364.53445, "Y"=342.4479}, {"X"=345.5035, "Y"=350.54803}, {"X"=320.73315, "Y"=307.0677}, {"X"=303.37704, "Y"=315.30927}, {"X"=291.4133, "Y"=310.72443}, {"X"=286.13464, "Y"=319.22586}, {"X"=279.3223, "Y"=314.76428}, {"X"=272.15247, "Y"=340.3479}, {"X"=306.28723, "Y"=345.39288}, {"X"=334.77283, "Y"=371.52417}, {"X"=352.84213, "Y"=397.19534}, {"X"=377.3774, "Y"=426.94626}, {"X"=390.7318, "Y"=431.3987}, {"X"=399.2997, "Y"=427.45007}, {"X"=402.81738, "Y"=423.37912}, {"X"=396.76886, "Y"=402.38965}, {"X"=388.56946, "Y"=393.81863}, {"X"=367.47476, "Y"=359.55594}, {"X"=350.95325, "Y"=337.8632}, {"X"=351.17017, "Y"=329.29697}, {"X"=350.10217, "Y"=303.40482}, {"X"=342.00015, "Y"=281.48672}, {"X"=333.54745, "Y"=272.55643}, {"X"=344.35553, "Y"=255.24062}, {"X"=350.2223, "Y"=228.83269}, {"X"=363.94193, "Y"=238.01378}, {"X"=363.70215, "Y"=246.85532}, {"X"=374.9105, "Y"=220.48444}, {"X"=385.1248, "Y"=229.61436}, {"X"=393.13916, "Y"=251.92992}, {"X"=389.94067, "Y"=243.0239}, {"X"=385.1248, "Y"=229.61436}, {"X"=363.82196, "Y"=242.43791}, {"X"=346.62537, "Y"=233.19218}, {"X"=340.0591, "Y"=215.24452}, {"X"=339.65118, "Y"=233.0359}, {"X"=229.62982, "Y"=283.3111}, {"X"=227.88667, "Y"=287.62378}, {"X"=229.54095, "Y"=305.004}, {"X"=227.64172, "Y"=352.1212}, {"X"=232.62094, "Y"=381.846}, {"X"=232.5815, "Y"=390.2492}, {"X"=227.52928, "Y"=381.7296}, {"X"=234.29721, "Y"=386.0895}, {"X"=241.0554, "Y"=390.4431}, {"X"=249.56197, "Y"=386.43863}, {"X"=261.51776, "Y"=378.29477}, {"X"=273.86276, "Y"=340.38678}, {"X"=287.66788, "Y"=332.14383}, {"X"=311.88943, "Y"=319.8097}, {"X"=317.6264, "Y"=289.64996}, {"X"=336.813, "Y"=281.36975}, {"X"=335.18146, "Y"=276.9664}, {"X"=338.6421, "Y"=277.0444}, {"X"=354.3279, "Y"=273.02457}, {"X"=356.40067, "Y"=259.9113}, {"X"=356.51465, "Y"=255.51389}, {"X"=365.32104, "Y"=251.30507}, {"X"=365.32104, "Y"=251.30507}, {"X"=372.27512, "Y"=251.46127}, {"X"=372.27512, "Y"=251.46127}, {"X"=360.10565, "Y"=251.18793}, {"X"=346.30515, "Y"=246.46478}, {"X"=316.81845, "Y"=241.38336}, {"X"=299.3422, "Y"=245.41052}, {"X"=300.79352, "Y"=263.05338}, {"X"=307.19315, "Y"=293.7609}, {"X"=318.5051, "Y"=332.84402}, {"X"=344.98547, "Y"=371.75723}, {"X"=364.7054, "Y"=397.46695}, {"X"=369.54807, "Y"=405.94815}, {"X"=381.13638, "Y"=414.55972}, {"X"=381.5246, "Y"=402.04044}, {"X"=368.215, "Y"=393.35287}, {"X"=360.3056, "Y"=372.10684}, {"X"=336.76624, "Y"=358.85632}, {"X"=316.54382, "Y"=345.62616}, {"X"=306.66272, "Y"=323.99228}, {"X"=303.4501, "Y"=310.99698}, {"X"=294.91904, "Y"=306.48352}, {"X"=286.55725, "Y"=288.9485}, {"X"=276.30807, "Y"=280.0052}, {"X"=276.36115, "Y"=275.6406}, {"X"=264.34177, "Y"=266.61862}, {"X"=246.89693, "Y"=283.70074}, {"X"=239.83669, "Y"=309.55658}, {"X"=226.05544, "Y"=317.86398}, {"X"=207.17874, "Y"=313.12982}, {"X"=184.90215, "Y"=325.52368}, {"X"=164.46835, "Y"=342.16727}, {"X"=283.04742, "Y"=293.21542}, {"X"=284.772, "Y"=293.2544}, {"X"=291.5417, "Y"=302.08032}, {"X"=291.5417, "Y"=302.08032}, {"X"=291.5417, "Y"=302.08032}, {"X"=309.46313, "Y"=263.24844}, {"X"=309.46313, "Y"=263.24844}, {"X"=314.50092, "Y"=272.12738}, {"X"=309.3068, "Y"=272.01038}, {"X"=295.86398, "Y"=245.33244}, {"X"=270.31674, "Y"=195.7796}, {"X"=251.23767, "Y"=168.29065}, {"X"=240.75018, "Y"=154.43251}, {"X"=230.2148, "Y"=140.51106}, {"X"=212.54332, "Y"=121.77149}, {"X"=198.33557, "Y"=112.241234}, {"X"=171.60019, "Y"=97.77416}, {"X"=166.31877, "Y"=106.91643}, {"X"=166.288, "Y"=102.29007}, {"X"=155.45392, "Y"=83.47714}, {"X"=153.62814, "Y"=78.77538}, {"X"=151.79955, "Y"=74.06634}, {"X"=326.53012, "Y"=276.7714}, {"X"=322.71722, "Y"=294.1116}, {"X"=323.0697, "Y"=276.6934}, {"X"=322.71722, "Y"=294.1116}, {"X"=315.98303, "Y"=285.2597}, {"X"=316.066, "Y"=280.90186}, {"X"=310.72165, "Y"=289.49408}, {"X"=308.99548, "Y"=289.4551}, {"X"=310.0943, "Y"=324.0701}, {"X"=328.51065, "Y"=345.89835}, {"X"=343.58987, "Y"=359.01178}, {"X"=368.81738, "Y"=372.3011}, {"X"=371.11853, "Y"=410.1601}, {"X"=374.50082, "Y"=410.23764}, {"X"=379.9594, "Y"=397.8162}, {"X"=373.30338, "Y"=393.46933}, {"X"=351.79425, "Y"=371.91263}, {"X"=328.23706, "Y"=358.66202}, {"X"=308.07278, "Y"=341.16443}, {"X"=306.66272, "Y"=323.99228}, {"X"=300.294, "Y"=293.60504}, {"X"=288.40732, "Y"=280.27808}, {"X"=266.07397, "Y"=266.65762}, {"X"=257.41312, "Y"=266.46265}, {"X"=238.45908, "Y"=248.45555}, {"X"=228.06985, "Y"=239.39224}, {"X"=219.39192, "Y"=230.341}, {"X"=219.39192, "Y"=230.341}, {"X"=221.18053, "Y"=212.58682}, {"X"=226.37666, "Y"=226.05904}, {"X"=250.75563, "Y"=231.04382}, {"X"=289.0338, "Y"=236.33417}, {"X"=318.21814, "Y"=259.05264}, {"X"=330.27206, "Y"=263.71664}, {"X"=347.50772, "Y"=268.491}, {"X"=370.16306, "Y"=264.61423}, {"X"=382.30566, "Y"=264.88745}, {"X"=395.18182, "Y"=295.7487}, {"X"=408.98813, "Y"=296.0606}, {"X"=410.71402, "Y"=296.09958}, {"X"=416.04984, "Y"=291.87222}, {"X"=410.25272, "Y"=309.0935}, {"X"=405.53644, "Y"=295.98264}, {"X"=400.35907, "Y"=295.86566}, {"X"=378.44476, "Y"=277.94153}, {"X"=381.9063, "Y"=278.01956}, {"X"=375.49518, "Y"=260.34067}, {"X"=378.83624, "Y"=264.8094}, {"X"=354.4401, "Y"=268.6471}, {"X"=354.3279, "Y"=273.02457}, {"X"=357.3342, "Y"=290.5465}, {"X"=374.22122, "Y"=303.95032}, {"X"=395.91693, "Y"=377.14545}, {"X"=413.55518, "Y"=406.95682}, {"X"=429.32974, "Y"=436.42618}, {"X"=450.9318, "Y"=482.06744}, {"X"=455.21838, "Y"=498.4042}, {"X"=465.40424, "Y"=494.58972}, {"X"=461.5119, "Y"=506.63376}, {"X"=434.05655, "Y"=485.74493}, {"X"=417.38504, "Y"=440.28506}, {"X"=390.59613, "Y"=435.53503}, {"X"=369.4274, "Y"=410.1213}, {"X"=372.93283, "Y"=406.02576}, {"X"=361.6611, "Y"=384.79556}, {"X"=344.00073, "Y"=341.98114}, {"X"=330.4989, "Y"=333.11636}, {"X"=324.26416, "Y"=302.82043}, {"X"=317.6264, "Y"=289.64996}, {"X"=309.3068, "Y"=272.01038}, {"X"=314.99506, "Y"=245.76192}, {"X"=308.03806, "Y"=245.60574}, {"X"=304.7095, "Y"=236.68565}, {"X"=290.58258, "Y"=249.62633}, {"X"=302.23608, "Y"=280.58994}, {"X"=278.3641, "Y"=253.75748}, {"X"=281.8942, "Y"=249.43117}, {"X"=278.6947, "Y"=227.23076}, {"X"=273.41083, "Y"=231.55151}, {"X"=282.35757, "Y"=213.95453}, {"X"=290.96927, "Y"=223.05957}, {"X"=308.66144, "Y"=210.0759}, {"X"=322.30545, "Y"=228.20746}, {"X"=325.7948, "Y"=228.28561}, {"X"=334.42072, "Y"=232.9187}, {"X"=339.5496, "Y"=237.46686}, {"X"=346.4117, "Y"=242.0473}, {"X"=351.0836, "Y"=264.18494}, {"X"=361.72598, "Y"=255.63101}, {"X"=386.32095, "Y"=247.36307}, {"X"=393.56595, "Y"=238.67802}, {"X"=427.5821, "Y"=261.512}, {"X"=431.739, "Y"=243.96165}, {"X"=451.64655, "Y"=226.65598}, {"X"=462.1308, "Y"=226.89064}, {"X"=451.27274, "Y"=235.53725}, {"X"=422.1093, "Y"=221.54025}, {"X"=399.67767, "Y"=212.10948}, {"X"=390.64197, "Y"=220.83633}, {"X"=383.24454, "Y"=234.0128}, {"X"=366.29364, "Y"=215.83102}, {"X"=345.3057, "Y"=215.36182}, {"X"=339.5496, "Y"=237.46686}, {"X"=323.78113, "Y"=241.53957}, {"X"=299.62646, "Y"=227.69954}, {"X"=252.3571, "Y"=248.76772}, {"X"=250.28375, "Y"=292.47525}, {"X"=220.88441, "Y"=326.34027}, {"X"=215.68538, "Y"=360.34036}, {"X"=203.76375, "Y"=364.30472}, {"X"=205.4654, "Y"=360.1074}, {"X"=205.46431, "Y"=347.3611}, {"X"=215.7217, "Y"=339.0651}, {"X"=224.31169, "Y"=326.41806}, {"X"=217.44861, "Y"=330.54938}, {"X"=243.3307, "Y"=300.98993}, {"X"=259.02493, "Y"=279.61542}, {"X"=264.34177, "Y"=266.61862}, {"X"=276.25507, "Y"=284.36322}, {"X"=269.44247, "Y"=275.48465}, {"X"=250.48476, "Y"=266.30664}, {"X"=248.8175, "Y"=257.49197}, {"X"=236.69861, "Y"=252.82106}, {"X"=229.73734, "Y"=257.0629}, {"X"=229.79147, "Y"=243.84921}, {"X"=191.56172, "Y"=247.40216}, {"X"=170.72264, "Y"=246.93408}, {"X"=425.7513, "Y"=309.44424}, {"X"=415.73383, "Y"=300.55435}, {"X"=-423.1004, "Y"=-1143.6017}] {"Y" format="%.2f"; "X" format="%.2f"}
  in  "auto bottom ChenJin vs DuPengYu":T1[](array[typedef])=[{"X"=385.56198, "Y"=827.943}, {"X"=385.56198, "Y"=827.943}, {"X"=385.56198, "Y"=827.943}, {"X"=382.19427, "Y"=1057.2422}, {"X"=382.07922, "Y"=1060.511}, {"X"=379.19833, "Y"=1057.1677}, {"X"=375.36856, "Y"=1037.3528}, {"X"=376.14993, "Y"=1014.16876}, {"X"=375.70258, "Y"=1027.4429}, {"X"=372.79865, "Y"=1024.0563}, {"X"=362.34756, "Y"=1020.47864}, {"X"=353.3929, "Y"=1016.9338}, {"X"=346.3073, "Y"=1000.0768}, {"X"=345.06854, "Y"=989.9842}, {"X"=332.0943, "Y"=1023.0487}, {"X"=312.08072, "Y"=1042.373}, {"X"=296.83047, "Y"=1055.1208}, {"X"=287.95444, "Y"=1048.346}, {"X"=280.07126, "Y"=1074.2648}, {"X"=275.64294, "Y"=1070.905}, {"X"=270.95493, "Y"=1086.9929}, {"X"=266.41464, "Y"=1093.332}, {"X"=264.96756, "Y"=1090.0718}, {"X"=261.95874, "Y"=1093.2208}, {"X"=269.18045, "Y"=1109.4592}, {"X"=281.02527, "Y"=1109.7555}, {"X"=286.73926, "Y"=1122.6711}, {"X"=303.7696, "Y"=1157.8875}, {"X"=342.8482, "Y"=1177.6433}, {"X"=372.26776, "Y"=1215.5067}, {"X"=387.04016, "Y"=1285.4816}, {"X"=405.19357, "Y"=1261.9622}, {"X"=422.1698, "Y"=1268.4127}, {"X"=416.4277, "Y"=1268.2665}, {"X"=-423.1004, "Y"=-1143.6017}, {"X"=400.88202, "Y"=1261.8523}, {"X"=395.25214, "Y"=1258.6943}, {"X"=391.87088, "Y"=1234.3545}, {"X"=382.5336, "Y"=1212.6946}, {"X"=374.7864, "Y"=1184.6749}, {"X"=368.52255, "Y"=1153.2262}, {"X"=358.33688, "Y"=1149.8191}, {"X"=344.04553, "Y"=1187.0062}, {"X"=340.61432, "Y"=1205.4785}, {"X"=331.89636, "Y"=1205.258}, {"X"=303.67322, "Y"=1235.1608}, {"X"=271.34134, "Y"=1276.5571}, {"X"=242.63857, "Y"=1287.7509}, {"X"=225.51692, "Y"=1287.3135}, {"X"=209.82121, "Y"=1289.8845}, {"X"=222.62198, "Y"=1299.1055}, {"X"=231.19252, "Y"=1293.399}, {"X"=248.39902, "Y"=1281.9424}, {"X"=246.81747, "Y"=1299.7244}, {"X"=251.08762, "Y"=1299.8336}, {"X"=254.325, "Y"=1261.1312}, {"X"=256.04227, "Y"=1233.9517}, {"X"=256.16876, "Y"=1221.7563}, {"X"=244.74164, "Y"=1203.0536}, {"X"=243.43193, "Y"=1184.467}, {"X"=222.97078, "Y"=1199.4207}, {"X"=195.35382, "Y"=1192.5466}, {"X"=185.32938, "Y"=1229.1134}, {"X"=186.809, "Y"=1238.2693}, {"X"=182.50154, "Y"=1241.1915}, {"X"=182.53098, "Y"=1247.2444}, {"X"=192.59729, "Y"=1247.5004}, {"X"=202.64139, "Y"=1214.2781}, {"X"=205.5362, "Y"=1195.8939}, {"X"=202.6076, "Y"=1164.7433}, {"X"=192.34113, "Y"=1155.0845}, {"X"=186.45357, "Y"=1148.6497}, {"X"=183.46098, "Y"=1135.9526}, {"X"=184.85097, "Y"=1116.9326}, {"X"=187.73447, "Y"=1097.8019}, {"X"=190.64049, "Y"=1078.5216}, {"X"=189.09726, "Y"=1062.2402}, {"X"=187.56798, "Y"=1052.4056}, {"X"=189.09726, "Y"=1062.2402}, {"X"=192.08398, "Y"=1062.3146}, {"X"=198.05244, "Y"=1059.2017}, {"X"=209.99753, "Y"=1072.5193}, {"X"=221.89182, "Y"=1082.5369}, {"X"=230.78673, "Y"=1089.2188}, {"X"=242.62737, "Y"=1095.9579}, {"X"=252.9255, "Y"=1105.8495}, {"X"=266.1416, "Y"=1115.7775}, {"X"=271.971, "Y"=1122.3011}, {"X"=272.01355, "Y"=1119.1154}, {"X"=264.5496, "Y"=1125.298}, {"X"=244.01294, "Y"=1108.8297}, {"X"=238.15411, "Y"=1099.0616}, {"X"=233.84915, "Y"=1073.1134}, {"X"=235.47443, "Y"=1050.3217}, {"X"=229.4685, "Y"=1053.4469}, {"X"=224.87978, "Y"=1079.3751}, {"X"=220.38525, "Y"=1088.9592}, {"X"=220.3946, "Y"=1085.7316}, {"X"=221.91254, "Y"=1076.0608}, {"X"=227.829, "Y"=1085.9171}, {"X"=246.06326, "Y"=1037.4432}, {"X"=253.20035, "Y"=1076.8403}, {"X"=260.4029, "Y"=1099.6174}, {"X"=269.3032, "Y"=1099.8398}, {"X"=278.064, "Y"=1109.6814}, {"X"=291.3902, "Y"=1110.0148}, {"X"=297.2543, "Y"=1113.361}, {"X"=312.25928, "Y"=1104.1251}, {"X"=324.12244, "Y"=1104.4216}, {"X"=328.4921, "Y"=1107.7389}, {"X"=332.77426, "Y"=1114.2498}, {"X"=335.56723, "Y"=1120.7069}, {"X"=337.1301, "Y"=1117.5544}, {"X"=327.78326, "Y"=1136.408}, {"X"=318.79773, "Y"=1142.5122}, {"X"=312.32806, "Y"=1100.9148}, {"X"=296.6105, "Y"=1148.2682}, {"X"=290.57028, "Y"=1157.5554}, {"X"=285.10938, "Y"=1132.1666}, {"X"=281.17105, "Y"=1100.1364}, {"X"=284.39197, "Y"=1084.0955}, {"X"=294.40884, "Y"=1106.8867}, {"X"=298.73416, "Y"=1113.398}, {"X"=318.3648, "Y"=1161.3932}, {"X"=354.82434, "Y"=1168.5765}, {"X"=381.41528, "Y"=1203.4269}, {"X"=400.5162, "Y"=1270.8646}, {"X"=430.36182, "Y"=1277.6212}, {"X"=448.31503, "Y"=1263.0598}, {"X"=454.41278, "Y"=1284.2162}, {"X"=462.5207, "Y"=1293.3677}, {"X"=455.22186, "Y"=1296.1553}, {"X"=458.07745, "Y"=1296.2283}, {"X"=456.98352, "Y"=1316.9158}, {"X"=453.41446, "Y"=1357.7206}, {"X"=452.5054, "Y"=1375.0096}, {"X"=451.4018, "Y"=1369.2245}, {"X"=471.63382, "Y"=1334.9055}, {"X"=471.63382, "Y"=1334.9055}, {"X"=292.3081, "Y"=968.4423}, {"X"=293.42435, "Y"=992.0689}, {"X"=297.72964, "Y"=1005.5626}, {"X"=300.879, "Y"=998.95544}, {"X"=304.89844, "Y"=1025.6896}, {"X"=313.37097, "Y"=1052.2566}, {"X"=321.98218, "Y"=1068.8047}, {"X"=329.2092, "Y"=1078.7344}, {"X"=336.07065, "Y"=1101.508}, {"X"=349.05676, "Y"=1114.6572}, {"X"=372.39667, "Y"=1169.019}, {"X"=397.77838, "Y"=1194.5654}, {"X"=407.8509, "Y"=1197.9155}, {"X"=410.869, "Y"=1160.5815}, {"X"=406.52188, "Y"=1194.7863}, {"X"=400.94064, "Y"=1188.4423}, {"X"=381.51993, "Y"=1159.8433}, {"X"=368.6268, "Y"=1150.0776}, {"X"=354.40295, "Y"=1133.9045}, {"X"=341.30588, "Y"=1127.2216}, {"X"=-423.1004, "Y"=-1143.6017}, {"X"=306.33865, "Y"=1029.035}, {"X"=301.76025, "Y"=1032.2269}, {"X"=297.24786, "Y"=1032.1151}, {"X"=295.80273, "Y"=1028.774}, {"X"=294.2397, "Y"=1032.0405}, {"X"=286.56076, "Y"=1041.7399}, {"X"=283.3054, "Y"=1058.0555}, {"X"=281.56253, "Y"=1074.3019}, {"X"=276.8582, "Y"=1090.3685}, {"X"=271.54837, "Y"=1153.9348}, {"X"=271.33908, "Y"=1169.6002}, {"X"=262.4554, "Y"=1178.7307}, {"X"=241.86002, "Y"=1199.8983}, {"X"=217.0745, "Y"=1236.0022}, {"X"=196.91728, "Y"=1250.6306}, {"X"=186.809, "Y"=1238.2693}, {"X"=199.81483, "Y"=1268.748}, {"X"=209.83815, "Y"=1269.0035}, {"X"=228.48264, "Y"=1263.4789}, {"X"=238.47949, "Y"=1269.7336}, {"X"=251.56924, "Y"=1249.0}, {"X"=262.02686, "Y"=1215.7823}, {"X"=269.55182, "Y"=1194.4214}, {"X"=266.83472, "Y"=1178.8412}, {"X"=250.89226, "Y"=1165.9592}, {"X"=237.78333, "Y"=1156.2277}, {"X"=218.81595, "Y"=1120.9696}, {"X"=208.51025, "Y"=1065.9805}, {"X"=199.55519, "Y"=1065.7576}, {"X"=190.51013, "Y"=1036.0654}, {"X"=178.28358, "Y"=995.9293}, {"X"=170.74214, "Y"=999.0866}, {"X"=178.21034, "Y"=982.5093}, {"X"=199.46654, "Y"=996.4522}, {"X"=208.52873, "Y"=1029.9164}, {"X"=219.02655, "Y"=1040.0642}, {"X"=231.01425, "Y"=1043.6489}, {"X"=253.38536, "Y"=1057.3116}, {"X"=263.93246, "Y"=1051.0286}, {"X"=269.88245, "Y"=1054.4512}, {"X"=279.6875, "Y"=1100.0994}, {"X"=281.81982, "Y"=1154.1931}, {"X"=281.9171, "Y"=1147.8989}, {"X"=271.25574, "Y"=1175.8385}, {"X"=247.69897, "Y"=1196.9595}, {"X"=224.30734, "Y"=1230.1025}, {"X"=195.45374, "Y"=1238.4889}, {"X"=182.4868, "Y"=1238.1594}, {"X"=201.2467, "Y"=1268.7845}, {"X"=208.40622, "Y"=1268.967}, {"X"=218.477, "Y"=1251.1791}, {"X"=235.59662, "Y"=1272.6547}, {"X"=254.2645, "Y"=1267.1377}, {"X"=265.99347, "Y"=1246.3419}, {"X"=271.66946, "Y"=1252.5322}, {"X"=274.8912, "Y"=1228.3383}, {"X"=288.2091, "Y"=1210.3071}, {"X"=290.08585, "Y"=1185.6444}, {"X"=290.2467, "Y"=1176.3173}, {"X"=287.58502, "Y"=1160.6187}, {"X"=289.42416, "Y"=1138.6122}, {"X"=294.23764, "Y"=1116.4807}, {"X"=310.98022, "Y"=1094.4447}, {"X"=334.3373, "Y"=1111.089}, {"X"=350.63046, "Y"=1111.4966}, {"X"=375.92374, "Y"=1108.9249}, {"X"=389.3261, "Y"=1147.4424}, {"X"=396.19382, "Y"=1160.2124}, {"X"=410.869, "Y"=1160.5815}, {"X"=417.1449, "Y"=1151.2968}, {"X"=417.00955, "Y"=1154.445}, {"X"=412.9991, "Y"=1144.8774}, {"X"=410.4484, "Y"=1135.3102}, {"X"=422.52844, "Y"=1129.2571}, {"X"=417.5742, "Y"=1106.7574}, {"X"=413.9373, "Y"=1157.5153}, {"X"=208.50858, "Y"=1069.2334}, {"X"=219.0437, "Y"=1033.4772}, {"X"=228.14581, "Y"=1013.83606}, {"X"=235.68819, "Y"=1014.0226}, {"X"=255.33244, "Y"=1011.18176}, {"X"=258.2141, "Y"=1024.5336}, {"X"=273.36075, "Y"=1018.2768}, {"X"=282.30765, "Y"=1025.1302}, {"X"=285.424, "Y"=1018.5753}, {"X"=292.90677, "Y"=1022.07874}, {"X"=306.07568, "Y"=1042.224}, {"X"=318.0126, "Y"=1045.8083}, {"X"=325.0469, "Y"=1065.6227}, {"X"=332.19064, "Y"=1078.8087}, {"X"=336.40842, "Y"=1088.6257}, {"X"=346.82382, "Y"=1088.8856}, {"X"=351.38214, "Y"=1085.7661}, {"X"=358.52988, "Y"=1095.6318}, {"X"=370.41937, "Y"=1095.9286}, {"X"=380.9368, "Y"=1092.9661}, {"X"=393.71402, "Y"=1109.3698}, {"X"=404.22076, "Y"=1106.4237}, {"X"=403.50403, "Y"=1087.0658}, {"X"=404.47766, "Y"=1100.0001}, {"X"=402.0146, "Y"=1087.0287}, {"X"=399.76987, "Y"=1106.3125}, {"X"=399.76987, "Y"=1106.3125}, {"X"=378.4894, "Y"=1034.1284}, {"X"=373.23868, "Y"=1010.7646}, {"X"=365.46985, "Y"=1017.2325}, {"X"=361.35016, "Y"=1003.7934}, {"X"=353.68472, "Y"=1006.94495}, {"X"=339.45584, "Y"=1029.8553}, {"X"=328.6761, "Y"=1039.4922}, {"X"=321.0887, "Y"=1042.5966}, {"X"=312.15027, "Y"=1039.0823}, {"X"=301.57205, "Y"=1042.1123}, {"X"=293.77866, "Y"=1058.3158}, {"X"=277.13513, "Y"=1070.9421}, {"X"=273.97366, "Y"=1083.8357}, {"X"=269.55017, "Y"=1080.4886}, {"X"=278.204, "Y"=1100.0623}, {"X"=285.1603, "Y"=1128.9933}, {"X"=292.1471, "Y"=1151.3064}, {"X"=325.4649, "Y"=1170.9637}, {"X"=364.36642, "Y"=1190.6223}, {"X"=389.55905, "Y"=1219.0127}, {"X"=425.7288, "Y"=1253.4287}, {"X"=442.31256, "Y"=1238.6799}, {"X"=438.29, "Y"=1201.7767}, {"X"=448.31503, "Y"=1263.0598}, {"X"=426.00516, "Y"=1247.3793}, {"X"=400.41992, "Y"=1237.6166}, {"X"=389.09586, "Y"=1231.2351}, {"X"=369.3667, "Y"=1215.4332}, {"X"=343.60764, "Y"=1202.471}, {"X"=319.10712, "Y"=1192.5785}, {"X"=301.69043, "Y"=1189.0399}, {"X"=285.76227, "Y"=1182.429}, {"X"=268.73434, "Y"=1144.4135}, {"X"=254.84932, "Y"=1060.6143}, {"X"=237.11465, "Y"=1027.3202}, {"X"=205.51903, "Y"=993.2534}, {"X"=185.7553, "Y"=972.5846}, {"X"=175.03316, "Y"=958.77747}, {"X"=167.20715, "Y"=931.2821}, {"X"=159.4536, "Y"=920.7783}, {"X"=151.92302, "Y"=934.3364}, {"X"=163.12627, "Y"=992.20746}, {"X"=166.20648, "Y"=998.9746}, {"X"=169.25446, "Y"=1002.38885}, {"X"=176.8091, "Y"=1002.5755}, {"X"=188.94211, "Y"=1016.18805}, {"X"=205.52156, "Y"=1023.22876}, {"X"=225.11635, "Y"=1017.0831}, {"X"=238.57639, "Y"=1033.9614}, {"X"=247.42906, "Y"=1053.8932}, {"X"=254.97723, "Y"=1047.5271}, {"X"=262.17734, "Y"=1073.819}, {"X"=268.10135, "Y"=1077.2117}, {"X"=271.12405, "Y"=1074.0419}, {"X"=281.46426, "Y"=1080.7856}, {"X"=287.36874, "Y"=1084.1697}, {"X"=301.87967, "Y"=1103.8657}, {"X"=324.8364, "Y"=1136.334}, {"X"=351.80267, "Y"=1171.6273}, {"X"=356.00116, "Y"=1177.975}, {"X"=381.30405, "Y"=1206.5077}, {"X"=409.7283, "Y"=1222.5881}, {"X"=442.96246, "Y"=1283.924}, {"X"=455.37714, "Y"=1293.1852}, {"X"=462.04916, "Y"=1275.4329}, {"X"=461.09195, "Y"=1293.3312}, {"X"=444.5426, "Y"=1280.9755}, {"X"=425.7884, "Y"=1283.4857}, {"X"=412.3797, "Y"=1262.145}, {"X"=396.0868, "Y"=1237.5066}, {"X"=367.71152, "Y"=1221.5234}, {"X"=337.45825, "Y"=1214.6252}, {"X"=316.12408, "Y"=1195.598}, {"X"=298.71686, "Y"=1192.0635}, {"X"=278.51346, "Y"=1179.1357}, {"X"=241.8828, "Y"=1196.8125}, {"X"=208.4326, "Y"=1217.4875}, {"X"=182.3831, "Y"=1216.8274}, {"X"=173.57819, "Y"=1198.1719}, {"X"=167.9369, "Y"=1219.5199}, {"X"=178.16472, "Y"=1238.0497}, {"X"=196.86601, "Y"=1223.308}, {"X"=215.67543, "Y"=1214.6083}, {"X"=220.01144, "Y"=1217.7809}, {"X"=234.5403, "Y"=1208.9486}, {"X"=253.63637, "Y"=1184.7245}, {"X"=266.75726, "Y"=1185.0557}, {"X"=277.28073, "Y"=1163.4935}, {"X"=304.02057, "Y"=1145.2998}, {"X"=338.5238, "Y"=1120.7809}, {"X"=364.01285, "Y"=1063.3291}, {"X"=392.52325, "Y"=1021.2252}, {"X"=415.1639, "Y"=984.98065}, {"X"=425.30273, "Y"=961.52795}, {"X"=425.15674, "Y"=964.92395}, {"X"=428.35736, "Y"=961.60297}, {"X"=430.33298, "Y"=951.42535}, {"X"=422.39233, "Y"=958.05237}, {"X"=410.30267, "Y"=954.34705}, {"X"=399.21207, "Y"=964.2864}, {"X"=386.40375, "Y"=980.89996}, {"X"=376.5997, "Y"=1000.82446}, {"X"=359.82645, "Y"=1053.4106}, {"X"=355.65466, "Y"=1092.3351}, {"X"=361.30078, "Y"=1102.1384}, {"X"=364.47452, "Y"=1095.7802}, {"X"=348.96442, "Y"=1117.8507}, {"X"=344.25873, "Y"=1127.2955}, {"X"=350.25754, "Y"=1124.2623}, {"X"=367.98785, "Y"=1124.7065}, {"X"=377.99878, "Y"=1134.4963}, {"X"=385.2578, "Y"=1137.85}, {"X"=415.54004, "Y"=1154.4081}, {"X"=429.09174, "Y"=1179.8176}, {"X"=439.74573, "Y"=1201.8135}, {"X"=442.80756, "Y"=1198.7988}, {"X"=446.87158, "Y"=1205.0818}, {"X"=431.8936, "Y"=1213.944}, {"X"=411.6974, "Y"=1210.3566}, {"X"=401.77673, "Y"=1203.9417}, {"X"=384.66394, "Y"=1194.2343}, {"X"=364.87164, "Y"=1175.0796}, {"X"=357.84995, "Y"=1165.5217}, {"X"=359.6098, "Y"=1156.1492}, {"X"=360.00436, "Y"=1143.5468}, {"X"=361.5761, "Y"=1140.4231}, {"X"=-423.1004, "Y"=-1143.6017}, {"X"=219.03513, "Y"=1036.7728}, {"X"=223.63219, "Y"=1010.3981}, {"X"=226.70569, "Y"=997.1246}, {"X"=232.70642, "Y"=1007.29156}, {"X"=237.03304, "Y"=1040.511}, {"X"=250.50998, "Y"=1044.1329}, {"X"=258.04303, "Y"=1041.0322}, {"X"=259.50876, "Y"=1044.3562}, {"X"=262.25058, "Y"=1067.318}, {"X"=265.00586, "Y"=1086.8445}, {"X"=266.57178, "Y"=1080.4144}, {"X"=275.55234, "Y"=1077.3973}, {"X"=285.416, "Y"=1113.0647}, {"X"=291.16998, "Y"=1122.7821}, {"X"=302.36465, "Y"=1154.7097}, {"X"=326.61996, "Y"=1183.4597}, {"X"=359.79727, "Y"=1196.7014}, {"X"=379.98038, "Y"=1243.1761}, {"X"=408.6161, "Y"=1283.0475}, {"X"=418.23563, "Y"=1292.2365}, {"X"=421.95117, "Y"=1241.2046}, {"X"=425.51437, "Y"=1289.4448}, {"X"=419.93057, "Y"=1286.321}, {"X"=412.25043, "Y"=1265.1528}, {"X"=402.60754, "Y"=1219.3433}, {"X"=398.38983, "Y"=1179.0436}, {"X"=403.2787, "Y"=1166.6654}, {"X"=400.94064, "Y"=1188.4423}, {"X"=412.08914, "Y"=1201.1145}, {"X"=414.86755, "Y"=1204.2726}, {"X"=421.5935, "Y"=1216.7556}, {"X"=437.5694, "Y"=1186.2588}, {"X"=454.30362, "Y"=1202.1814}, {"X"=471.2695, "Y"=1211.8639}, {"X"=481.38226, "Y"=1263.9016}, {"X"=495.92682, "Y"=1285.2755}, {"X"=488.04114, "Y"=1273.095}, {"X"=466.71088, "Y"=1242.3412}, {"X"=440.3089, "Y"=1220.2982}, {"X"=402.85654, "Y"=1213.209}, {"X"=366.669, "Y"=1209.2173}, {"X"=322.02023, "Y"=1192.6521}, {"X"=292.0368, "Y"=1157.5924}, {"X"=258.61282, "Y"=1128.3276}, {"X"=218.8826, "Y"=1095.3647}, {"X"=188.99785, "Y"=1032.7323}, {"X"=166.28499, "Y"=1008.9802}, {"X"=157.03873, "Y"=988.7051}, {"X"=147.64194, "Y"=961.49664}, {"X"=149.01335, "Y"=947.9341}, {"X"=153.62874, "Y"=951.4533}, {"X"=161.436, "Y"=971.986}, {"X"=172.09772, "Y"=975.623}, {"X"=190.32593, "Y"=976.07184}, {"X"=211.57973, "Y"=990.0503}, {"X"=219.10406, "Y"=1010.2861}, {"X"=229.65427, "Y"=1013.87335}, {"X"=252.22168, "Y"=1021.07166}, {"X"=281.19717, "Y"=998.4696}, {"X"=298.03333, "Y"=988.8246}, {"X"=-423.1004, "Y"=-1143.6017}, {"X"=291.9652, "Y"=988.675}, {"X"=293.5402, "Y"=985.35144}, {"X"=296.33682, "Y"=998.8433}, {"X"=297.85086, "Y"=998.8807}, {"X"=304.89844, "Y"=1025.6896}, {"X"=309.01068, "Y"=1045.585}, {"X"=304.38107, "Y"=1052.0333}, {"X"=287.84732, "Y"=1054.8976}, {"X"=271.20898, "Y"=1067.541}, {"X"=251.85954, "Y"=1060.5399}, {"X"=219.05229, "Y"=1030.1772}, {"X"=190.39807, "Y"=999.57196}, {"X"=170.64899, "Y"=985.6841}, {"X"=162.87015, "Y"=961.87103}, {"X"=158.36478, "Y"=968.5315}, {"X"=161.40646, "Y"=968.6063}, {"X"=168.98637, "Y"=965.40936}, {"X"=185.7419, "Y"=969.2051}, {"X"=194.87595, "Y"=972.8091}, {"X"=210.0699, "Y"=983.29443}, {"X"=237.23788, "Y"=1007.40356}, {"X"=249.06665, "Y"=1037.5177}, {"X"=262.4715, "Y"=1047.7131}, {"X"=269.71588, "Y"=1067.5039}, {"X"=279.9269, "Y"=1083.9841}, {"X"=285.36472, "Y"=1116.2587}, {"X"=304.79358, "Y"=1179.7985}, {"X"=312.56973, "Y"=1158.1089}, {"X"=327.62686, "Y"=1142.7339}, {"X"=344.88504, "Y"=1104.9407}, {"X"=371.02606, "Y"=1209.3275}, {"X"=386.51105, "Y"=1261.4866}, {"X"=394.5425, "Y"=1276.7079}, {"X"=396.2129, "Y"=1270.7549}, {"X"=394.42477, "Y"=1279.6969}, {"X"=387.49298, "Y"=1273.5322}, {"X"=376.988, "Y"=1246.1337}, {"X"=369.88385, "Y"=1242.9197}, {"X"=368.74875, "Y"=1233.7677}, {"X"=373.22012, "Y"=1187.7426}, {"X"=381.0611, "Y"=1131.3976}, {"X"=389.62253, "Y"=1099.6292}, {"X"=396.55225, "Y"=1073.9155}, {"X"=406.82, "Y"=1041.4303}, {"X"=413.51285, "Y"=1025.0641}, {"X"=416.9454, "Y"=1015.17737}, {"X"=-423.1004, "Y"=-1143.6017}, {"X"=312.5695, "Y"=1019.24695}, {"X"=309.0782, "Y"=1042.2985}, {"X"=305.87936, "Y"=1052.0706}, {"X"=301.38455, "Y"=1051.9589}, {"X"=296.83047, "Y"=1055.1208}, {"X"=287.68716, "Y"=1064.6931}, {"X"=281.85883, "Y"=1054.7488}, {"X"=280.21622, "Y"=1064.5073}, {"X"=288.85715, "Y"=1084.2068}, {"X"=299.6695, "Y"=1142.0319}, {"X"=301.32446, "Y"=1132.5734}, {"X"=318.29297, "Y"=1164.526}, {"X"=347.05252, "Y"=1183.9752}, {"X"=369.1602, "Y"=1221.5602}, {"X"=409.91977, "Y"=1286.0656}, {"X"=426.66855, "Y"=1295.4257}, {"X"=422.6332, "Y"=1225.9758}, {"X"=425.51437, "Y"=1289.4448}, {"X"=416.29605, "Y"=1271.2667}, {"X"=410.1451, "Y"=1246.9762}, {"X"=397.53488, "Y"=1200.7466}, {"X"=394.0043, "Y"=1178.933}, {"X"=387.1574, "Y"=1166.2595}, {"X"=373.89838, "Y"=1124.8546}, {"X"=364.16684, "Y"=1105.4226}, {"X"=355.55762, "Y"=1095.5576}, {"X"=352.96658, "Y"=1082.5681}, {"X"=346.6139, "Y"=1043.2299}, {"X"=339.8074, "Y"=1016.5978}, {"X"=335.1091, "Y"=1023.12335}, {"X"=327.41248, "Y"=1029.557}, {"X"=325.67126, "Y"=1039.4176}, {"X"=330.5869, "Y"=1023.0114}, {"X"=336.01788, "Y"=1046.2552}, {"X"=341.04742, "Y"=1082.271}, {"X"=337.8107, "Y"=1091.8898}, {"X"=334.42032, "Y"=1107.8872}, {"X"=327.0826, "Y"=1164.7472}, {"X"=320.63654, "Y"=1189.5183}, {"X"=304.4798, "Y"=1195.3038}, {"X"=273.70233, "Y"=1209.94}, {"X"=244.37643, "Y"=1248.817}, {"X"=221.31331, "Y"=1263.2961}, {"X"=186.92859, "Y"=1268.4196}, {"X"=183.8581, "Y"=1222.9781}, {"X"=185.49684, "Y"=1268.383}, {"X"=201.2467, "Y"=1268.7845}, {"X"=208.40622, "Y"=1268.967}, {"X"=215.59013, "Y"=1257.1356}, {"X"=222.77873, "Y"=1254.3054}, {"X"=225.72623, "Y"=1236.2219}, {"X"=228.71048, "Y"=1214.9385}, {"X"=228.65309, "Y"=1227.1653}, {"X"=238.6224, "Y"=1248.6708}, {"X"=375.47977, "Y"=1034.0538}, {"X"=374.30643, "Y"=1024.0936}, {"X"=368.5963, "Y"=1013.98206}, {"X"=360.94092, "Y"=1017.1205}, {"X"=348.77026, "Y"=1020.14264}, {"X"=330.505, "Y"=1026.3237}, {"X"=316.94812, "Y"=1025.988}, {"X"=308.17944, "Y"=1012.48834}, {"X"=302.07562, "Y"=1015.66455}, {"X"=294.47202, "Y"=1018.7992}, {"X"=283.60953, "Y"=1038.3744}, {"X"=272.87646, "Y"=1054.5256}, {"X"=263.819, "Y"=1060.8373}, {"X"=257.80536, "Y"=1063.9497}, {"X"=253.16965, "Y"=1080.0803}, {"X"=250.19154, "Y"=1080.0061}, {"X"=250.92195, "Y"=997.7223}, {"X"=244.66304, "Y"=1024.198}, {"X"=243.40346, "Y"=990.8352}, {"X"=242.54118, "Y"=898.57715}, {"X"=247.89473, "Y"=997.6476}, {"X"=247.89473, "Y"=997.6476}, {"X"=204.03142, "Y"=1062.6118}, {"X"=210.00017, "Y"=1069.2706}, {"X"=222.03804, "Y"=1036.8473}, {"X"=231.19595, "Y"=1007.2542}, {"X"=241.86415, "Y"=994.1502}, {"X"=253.98094, "Y"=994.44916}, {"X"=267.49136, "Y"=1004.8157}, {"X"=279.6346, "Y"=1001.7755}, {"X"=288.7668, "Y"=998.65643}, {"X"=297.42795, "Y"=1022.1907}, {"X"=302.8828, "Y"=1051.9961}, {"X"=311.59644, "Y"=1065.288}, {"X"=316.15164, "Y"=1062.1388}, {"X"=315.7934, "Y"=1078.4}, {"X"=310.30396, "Y"=1126.4446}, {"X"=295.02692, "Y"=1154.5251}, {"X"=275.37265, "Y"=1194.5684}, {"X"=253.36496, "Y"=1212.496}, {"X"=235.9526, "Y"=1215.122}, {"X"=195.38734, "Y"=1207.9576}, {"X"=165.01901, "Y"=1216.3875}, {"X"=149.28238, "Y"=1231.2417}, {"X"=139.68742, "Y"=1267.2153}, {"X"=133.78181, "Y"=1255.0531}, {"X"=142.31163, "Y"=1249.2416}, {"X"=170.89537, "Y"=1228.7472}, {"X"=195.42728, "Y"=1226.3225}, {"X"=225.86406, "Y"=1202.5762}, {"X"=262.41943, "Y"=1181.84}, {"X"=304.02057, "Y"=1145.2998}, {"X"=337.3845, "Y"=1107.9613}, {"X"=351.829, "Y"=1121.1141}, {"X"=373.28342, "Y"=1099.2211}, {"X"=392.71445, "Y"=1096.4852}, {"X"=400.1468, "Y"=1096.6708}, {"X"=393.68802, "Y"=1070.5895}, {"X"=392.59344, "Y"=1099.7034}, {"X"=385.16626, "Y"=1099.5178}, {"X"=365.75354, "Y"=1102.2498}, {"X"=357.4365, "Y"=1082.6794}, {"X"=357.8313, "Y"=1069.697}, {"X"=366.37665, "Y"=1082.9023}, {"X"=380.3545, "Y"=1066.9987}, {"X"=397.67587, "Y"=1044.4967}, {"X"=425.72275, "Y"=1022.0467}, {"X"=444.30493, "Y"=1012.5209}, {"X"=464.32864, "Y"=976.0594}, {"X"=475.2595, "Y"=942.2591}, {"X"=479.49527, "Y"=949.2132}, {"X"=479.86115, "Y"=942.3718}, {"X"=472.65546, "Y"=962.6911}, {"X"=459.07513, "Y"=958.95306}, {"X"=437.21347, "Y"=968.6154}, {"X"=438.8938, "Y"=965.2615}, {"X"=399.9634, "Y"=984.60626}, {"X"=367.29825, "Y"=1007.28125}, {"X"=371.72696, "Y"=1010.72723}, {"X"=384.74353, "Y"=1027.6667}, {"X"=366.69003, "Y"=1073.172}, {"X"=351.19348, "Y"=1092.2238}, {"X"=332.8562, "Y"=1111.052}, {"X"=318.22122, "Y"=1167.6548}, {"X"=304.29248, "Y"=1204.5598}, {"X"=291.63947, "Y"=1262.0814}, {"X"=277.10855, "Y"=1273.7133}, {"X"=271.13788, "Y"=1291.4513}, {"X"=257.06705, "Y"=1273.2021}, {"X"=255.35788, "Y"=1299.9429}, {"X"=248.31978, "Y"=1290.8683}, {"X"=246.37314, "Y"=1181.4352}, {"X"=245.0139, "Y"=1168.937}, {"X"=244.76624, "Y"=1199.9718}, {"X"=245.69026, "Y"=1263.9171}, {"X"=251.42653, "Y"=1264.0632}, {"X"=250.07527, "Y"=1255.0}, {"X"=253.00784, "Y"=1249.0365}, {"X"=253.66672, "Y"=1181.6191}, {"X"=261.49084, "Y"=1134.7448}, {"X"=268.9769, "Y"=1125.4089}, {"X"=280.7836, "Y"=1125.7048}, {"X"=291.27994, "Y"=1116.4067}, {"X"=306.63852, "Y"=1161.0981}, {"X"=339.66977, "Y"=1186.8959}, {"X"=374.35754, "Y"=1197.0693}, {"X"=398.1364, "Y"=1222.2944}, {"X"=422.84866, "Y"=1253.3555}, {"X"=435.6654, "Y"=1256.704}, {"X"=436.2435, "Y"=1244.6053}, {"X"=438.98267, "Y"=1247.709}, {"X"=426.83847, "Y"=1229.1394}, {"X"=416.0556, "Y"=1210.4668}, {"X"=407.9792, "Y"=1194.8231}, {"X"=401.18912, "Y"=1182.2296}, {"X"=393.61923, "Y"=1150.7057}, {"X"=396.9271, "Y"=1141.3103}, {"X"=395.95062, "Y"=1166.4808}, {"X"=395.70807, "Y"=1172.7334}, {"X"=402.77548, "Y"=1179.1542}, {"X"=407.59476, "Y"=1204.0887}, {"X"=422.08722, "Y"=1238.1665}, {"X"=430.6426, "Y"=1271.6323}, {"X"=434.3752, "Y"=1283.7048}, {"X"=430.6426, "Y"=1271.6323}, {"X"=417.33392, "Y"=1280.2814}, {"X"=403.13846, "Y"=1276.927}, {"X"=386.51105, "Y"=1261.4866}, {"X"=371.32617, "Y"=1242.9564}, {"X"=347.25275, "Y"=1227.1213}, {"X"=328.757, "Y"=1214.4049}, {"X"=311.2227, "Y"=1220.092}, {"X"=291.38095, "Y"=1194.9729}, {"X"=284.4031, "Y"=1176.1699}, {"X"=271.0897, "Y"=1188.2673}, {"X"=247.59329, "Y"=1209.279}, {"X"=230.12831, "Y"=1221.0963}, {"X"=202.64972, "Y"=1226.5057}, {"X"=180.8409, "Y"=1198.3555}, {"X"=168.10406, "Y"=1240.8257}, {"X"=165.6049, "Y"=1285.7831}, {"X"=164.15268, "Y"=1282.7708}, {"X"=158.47394, "Y"=1285.601}, {"X"=161.24283, "Y"=1276.735}, {"X"=163.78506, "Y"=1240.716}, {"X"=164.94133, "Y"=1207.187}, {"X"=161.79057, "Y"=1179.3013}, {"X"=157.26189, "Y"=1163.6013}, {"X"=606.59064, "Y"=833.28534}] {"Y" format="%.2f"; "X" format="%.2f"}
  in  "manual bottom ChenJin vs DuPengYu":T1[](array[typedef])=[{"X"=378.82977, "Y"=1024.2056}, {"X"=381.49908, "Y"=1034.203}, {"X"=379.99423, "Y"=1034.1658}, {"X"=384.50885, "Y"=1034.2776}, {"X"=384.50885, "Y"=1034.2776}, {"X"=381.49908, "Y"=1034.203}, {"X"=388.35666, "Y"=1011.1382}, {"X"=388.95996, "Y"=994.4252}, {"X"=383.127, "Y"=987.5592}, {"X"=381.95795, "Y"=977.4139}, {"X"=371.30542, "Y"=977.1517}, {"X"=360.65356, "Y"=976.88947}, {"X"=354.46854, "Y"=980.11365}, {"X"=345.25293, "Y"=983.2585}, {"X"=325.18466, "Y"=996.206}, {"X"=298.9962, "Y"=1018.91113}, {"X"=288.11563, "Y"=1038.4862}, {"X"=281.90842, "Y"=1051.4751}, {"X"=280.5078, "Y"=1044.8774}, {"X"=280.36172, "Y"=1054.7115}, {"X"=277.32098, "Y"=1057.9067}, {"X"=275.68835, "Y"=1067.6525}, {"X"=272.61523, "Y"=1074.079}, {"X"=272.52863, "Y"=1080.5629}, {"X"=272.4422, "Y"=1087.03}, {"X"=269.34424, "Y"=1096.6251}, {"X"=283.9866, "Y"=1109.8296}, {"X"=326.46472, "Y"=1130.0288}, {"X"=342.25565, "Y"=1146.2601}, {"X"=373.75394, "Y"=1172.1803}, {"X"=404.87845, "Y"=1234.6846}, {"X"=425.7288, "Y"=1253.4287}, {"X"=423.39484, "Y"=1241.2413}, {"X"=417.75354, "Y"=1238.0565}, {"X"=397.65656, "Y"=1197.658}, {"X"=393.4068, "Y"=1194.4551}, {"X"=387.69366, "Y"=1191.2113}, {"X"=375.5422, "Y"=1162.832}, {"X"=365.13525, "Y"=1121.4474}, {"X"=377.2954, "Y"=1112.1636}, {"X"=368.82755, "Y"=1099.1097}, {"X"=364.37183, "Y"=1098.9985}, {"X"=358.92532, "Y"=1130.8425}, {"X"=357.4497, "Y"=1130.8055}, {"X"=328.94055, "Y"=1149.0804}, {"X"=310.50098, "Y"=1186.1597}, {"X"=269.19046, "Y"=1222.0864}, {"X"=248.71892, "Y"=1245.9027}, {"X"=227.06195, "Y"=1260.437}, {"X"=219.87947, "Y"=1263.2596}, {"X"=219.87077, "Y"=1266.2612}, {"X"=229.94656, "Y"=1257.501}, {"X"=253.00784, "Y"=1249.0365}, {"X"=266.1068, "Y"=1237.2473}, {"X"=269.4309, "Y"=1203.6781}, {"X"=272.50446, "Y"=1191.4015}, {"X"=271.5064, "Y"=1157.0759}, {"X"=265.7175, "Y"=1150.6421}, {"X"=256.94122, "Y"=1147.2714}, {"X"=253.88025, "Y"=1159.7705}, {"X"=221.67738, "Y"=1149.535}, {"X"=199.69766, "Y"=1177.148}, {"X"=199.72934, "Y"=1201.9152}, {"X"=189.56694, "Y"=1201.6581}, {"X"=191.06581, "Y"=1217.0475}, {"X"=196.83728, "Y"=1207.9943}, {"X"=202.62035, "Y"=1183.437}, {"X"=214.2904, "Y"=1177.516}, {"X"=221.61717, "Y"=1168.3477}, {"X"=220.2738, "Y"=1127.3666}, {"X"=209.9844, "Y"=1088.6996}, {"X"=201.02844, "Y"=1046.1875}, {"X"=183.06432, "Y"=1049.0197}, {"X"=190.5906, "Y"=1062.2775}, {"X"=187.4957, "Y"=1032.6951}, {"X"=191.96553, "Y"=1019.58014}, {"X"=188.9085, "Y"=1006.20917}, {"X"=184.40671, "Y"=1012.7542}, {"X"=187.44717, "Y"=1019.4683}, {"X"=193.45525, "Y"=1012.978}, {"X"=210.03741, "Y"=1023.34064}, {"X"=223.528, "Y"=1040.1759}, {"X"=229.45316, "Y"=1056.7167}, {"X"=229.42252, "Y"=1063.2435}, {"X"=241.3957, "Y"=1060.2797}, {"X"=259.057, "Y"=1086.696}, {"X"=279.63983, "Y"=1103.3098}, {"X"=275.2819, "Y"=1096.7734}, {"X"=291.72263, "Y"=1090.7395}, {"X"=288.96494, "Y"=1077.7316}, {"X"=268.59003, "Y"=1038.002}, {"X"=250.16281, "Y"=1083.242}, {"X"=242.8905, "Y"=1060.3168}, {"X"=237.09421, "Y"=1030.6244}, {"X"=228.2044, "Y"=1000.50555}, {"X"=217.59473, "Y"=1010.2488}, {"X"=216.0654, "Y"=1020.1767}, {"X"=223.5165, "Y"=1043.4629}, {"X"=223.505, "Y"=1046.7456}, {"X"=238.40616, "Y"=1060.2053}, {"X"=251.82962, "Y"=1063.801}, {"X"=262.14078, "Y"=1077.0631}, {"X"=259.16058, "Y"=1076.9889}, {"X"=269.59152, "Y"=1077.2488}, {"X"=281.56253, "Y"=1074.3019}, {"X"=303.6785, "Y"=1087.8093}, {"X"=309.49454, "Y"=1094.4076}, {"X"=318.62805, "Y"=1084.9492}, {"X"=314.16208, "Y"=1084.8379}, {"X"=322.8664, "Y"=1094.7415}, {"X"=330.3763, "Y"=1091.7042}, {"X"=328.96924, "Y"=1088.4402}, {"X"=331.45618, "Y"=1107.813}, {"X"=327.08838, "Y"=1104.4958}, {"X"=316.70786, "Y"=1104.2363}, {"X"=303.17377, "Y"=1113.509}, {"X"=295.77448, "Y"=1113.3239}, {"X"=293.20914, "Y"=1090.7766}, {"X"=288.96494, "Y"=1077.7316}, {"X"=278.48566, "Y"=1080.7114}, {"X"=279.78308, "Y"=1093.6658}, {"X"=281.46426, "Y"=1080.7856}, {"X"=295.94876, "Y"=1103.7175}, {"X"=332.28488, "Y"=1133.3499}, {"X"=352.7395, "Y"=1140.2013}, {"X"=379.83005, "Y"=1166.0751}, {"X"=413.28146, "Y"=1207.3165}, {"X"=429.7332, "Y"=1229.2128}, {"X"=436.9597, "Y"=1259.7557}, {"X"=440.27734, "Y"=1250.7722}, {"X"=445.59012, "Y"=1259.9753}, {"X"=457.2755, "Y"=1284.2892}, {"X"=453.1357, "Y"=1281.1946}, {"X"=443.79996, "Y"=1295.8634}, {"X"=441.63867, "Y"=1310.6227}, {"X"=433.25308, "Y"=1336.8431}, {"X"=434.8096, "Y"=1333.9603}, {"X"=442.03635, "Y"=1331.2194}, {"X"=284.5364, "Y"=978.3916}, {"X"=286.00327, "Y"=981.79895}, {"X"=288.9862, "Y"=985.2392}, {"X"=290.6163, "Y"=978.5413}, {"X"=291.85153, "Y"=995.38354}, {"X"=299.30325, "Y"=1002.2612}, {"X"=310.92316, "Y"=1025.8387}, {"X"=313.86472, "Y"=1029.2214}, {"X"=319.36453, "Y"=1052.4055}, {"X"=323.70587, "Y"=1059.0598}, {"X"=342.36, "Y"=1088.7743}, {"X"=371.88605, "Y"=1140.6819}, {"X"=399.74884, "Y"=1144.5447}, {"X"=417.2604, "Y"=1182.6349}, {"X"=412.87717, "Y"=1182.5243}, {"X"=408.19272, "Y"=1154.2234}, {"X"=394.10178, "Y"=1138.0719}, {"X"=375.15796, "Y"=1131.2495}, {"X"=362.27902, "Y"=1118.184}, {"X"=355.36392, "Y"=1101.9901}, {"X"=339.47083, "Y"=1085.469}, {"X"=327.10034, "Y"=979.4397}, {"X"=320.8667, "Y"=986.0249}, {"X"=315.01044, "Y"=975.76605}, {"X"=307.1359, "Y"=989.049}, {"X"=310.30832, "Y"=982.3977}, {"X"=304.16663, "Y"=985.61334}, {"X"=290.11404, "Y"=1008.71027}, {"X"=291.39975, "Y"=1022.04144}, {"X"=285.37177, "Y"=1021.8922}, {"X"=281.85883, "Y"=1054.7488}, {"X"=290.1815, "Y"=1093.9254}, {"X"=288.58887, "Y"=1100.3218}, {"X"=264.47424, "Y"=1131.6492}, {"X"=237.74265, "Y"=1162.4983}, {"X"=218.596, "Y"=1205.4706}, {"X"=199.74115, "Y"=1211.1382}, {"X"=193.95258, "Y"=1214.0581}, {"X"=191.11266, "Y"=1232.3035}, {"X"=209.86754, "Y"=1232.7795}, {"X"=240.29803, "Y"=1215.2319}, {"X"=250.46594, "Y"=1212.4226}, {"X"=269.9173, "Y"=1166.4384}, {"X"=269.95816, "Y"=1163.3092}, {"X"=278.9318, "Y"=1150.9742}, {"X"=286.22208, "Y"=1154.3038}, {"X"=280.73544, "Y"=1128.8823}, {"X"=263.18442, "Y"=1115.7034}, {"X"=239.94527, "Y"=1053.7073}, {"X"=202.5133, "Y"=1026.463}, {"X"=187.38618, "Y"=1002.8368}, {"X"=179.64024, "Y"=965.6714}, {"X"=171.84909, "Y"=938.249}, {"X"=167.38762, "Y"=955.1926}, {"X"=178.1367, "Y"=969.018}, {"X"=182.76134, "Y"=982.62146}, {"X"=191.9009, "Y"=996.26544}, {"X"=207.0311, "Y"=1003.3221}, {"X"=232.70642, "Y"=1007.29156}, {"X"=264.39075, "Y"=1011.4057}, {"X"=268.71338, "Y"=1028.1029}, {"X"=279.1515, "Y"=1034.9674}, {"X"=298.14706, "Y"=1064.9534}, {"X"=310.77643, "Y"=1104.0881}, {"X"=303.0484, "Y"=1119.8926}, {"X"=280.6393, "Y"=1135.2251}, {"X"=249.34576, "Y"=1175.2861}, {"X"=217.15913, "Y"=1199.2738}, {"X"=199.74115, "Y"=1211.1382}, {"X"=195.40735, "Y"=1217.1575}, {"X"=198.33063, "Y"=1235.5262}, {"X"=201.20221, "Y"=1223.418}, {"X"=224.3305, "Y"=1224.0044}, {"X"=251.85738, "Y"=1218.5879}, {"X"=274.8912, "Y"=1228.3383}, {"X"=292.28818, "Y"=1225.7277}, {"X"=289.60693, "Y"=1213.4137}, {"X"=292.83633, "Y"=1195.0096}, {"X"=300.53378, "Y"=1173.4581}, {"X"=302.61215, "Y"=1142.1058}, {"X"=291.00558, "Y"=1132.3146}, {"X"=295.8906, "Y"=1106.9237}, {"X"=292.98337, "Y"=1103.6433}, {"X"=299.0346, "Y"=1097.3667}, {"X"=312.39697, "Y"=1097.7004}, {"X"=336.74796, "Y"=1075.6764}, {"X"=369.46307, "Y"=1079.7374}, {"X"=400.1468, "Y"=1096.6708}, {"X"=417.5742, "Y"=1106.7574}, {"X"=411.5062, "Y"=1109.8147}, {"X"=427.24496, "Y"=1123.0027}, {"X"=424.14612, "Y"=1126.1134}, {"X"=412.0561, "Y"=1132.1746}, {"X"=405.0603, "Y"=1122.4471}, {"X"=406.2808, "Y"=1128.8499}, {"X"=403.45407, "Y"=1125.5951}, {"X"=407.75778, "Y"=1128.8868}, {"X"=192.01132, "Y"=1036.1027}, {"X"=208.53893, "Y"=1010.0249}, {"X"=231.32977, "Y"=980.45215}, {"X"=237.40373, "Y"=980.60175}, {"X"=246.59587, "Y"=970.70233}, {"X"=260.25497, "Y"=974.4183}, {"X"=272.64258, "Y"=957.7781}, {"X"=278.553, "Y"=971.4886}, {"X"=275.23322, "Y"=991.62024}, {"X"=287.3604, "Y"=991.9193}, {"X"=297.85086, "Y"=998.8807}, {"X"=313.9356, "Y"=1025.9135}, {"X"=324.16888, "Y"=1039.3804}, {"X"=323.8598, "Y"=1052.5172}, {"X"=325.0469, "Y"=1065.6227}, {"X"=332.76785, "Y"=1056.0139}, {"X"=335.3404, "Y"=1072.3914}, {"X"=351.38214, "Y"=1085.7661}, {"X"=371.0615, "Y"=1076.5311}, {"X"=396.4282, "Y"=1077.163}, {"X"=402.5253, "Y"=1074.0642}, {"X"=400.7783, "Y"=1080.5177}, {"X"=408.23514, "Y"=1080.7035}, {"X"=400.3989, "Y"=1090.2222}, {"X"=403.3758, "Y"=1090.2964}, {"X"=398.41077, "Y"=1103.0657}, {"X"=395.93365, "Y"=1090.1107}, {"X"=384.6261, "Y"=1030.9744}, {"X"=386.01373, "Y"=1034.315}, {"X"=391.2582, "Y"=1014.5423}, {"X"=383.58688, "Y"=1017.6806}, {"X"=374.23724, "Y"=980.6004}, {"X"=355.49326, "Y"=996.95386}, {"X"=350.19385, "Y"=969.8659}, {"X"=337.56842, "Y"=986.43646}, {"X"=329.48566, "Y"=1006.3471}, {"X"=321.8477, "Y"=1009.49457}, {"X"=318.75082, "Y"=1012.7497}, {"X"=296.15808, "Y"=1008.8597}, {"X"=274.68774, "Y"=1031.556}, {"X"=265.58627, "Y"=1037.9274}, {"X"=274.19522, "Y"=1067.6154}, {"X"=272.52863, "Y"=1080.5629}, {"X"=264.8911, "Y"=1096.5139}, {"X"=292.5911, "Y"=1126.0007}, {"X"=331.7993, "Y"=1152.3031}, {"X"=359.31522, "Y"=1165.5586}, {"X"=398.2672, "Y"=1182.1559}, {"X"=432.0367, "Y"=1210.8712}, {"X"=446.64688, "Y"=1238.79}, {"X"=448.39716, "Y"=1232.7394}, {"X"=435.81296, "Y"=1223.249}, {"X"=409.0493, "Y"=1204.1255}, {"X"=392.9315, "Y"=1206.8019}, {"X"=383.98514, "Y"=1212.7313}, {"X"=365.82428, "Y"=1190.6592}, {"X"=343.11047, "Y"=1168.2815}, {"X"=318.8702, "Y"=1139.3512}, {"X"=311.3728, "Y"=1145.4845}, {"X"=298.43564, "Y"=1129.326}, {"X"=284.9046, "Y"=1051.5494}, {"X"=265.86105, "Y"=1014.76886}, {"X"=234.36671, "Y"=980.527}, {"X"=203.98927, "Y"=952.6898}, {"X"=178.0812, "Y"=958.8524}, {"X"=156.48283, "Y"=931.0195}, {"X"=160.95857, "Y"=917.368}, {"X"=164.03088, "Y"=917.44305}, {"X"=154.88257, "Y"=924.109}, {"X"=153.45396, "Y"=934.37396}, {"X"=155.08685, "Y"=944.6727}, {"X"=165.94254, "Y"=965.33453}, {"X"=188.84085, "Y"=986.13257}, {"X"=208.54234, "Y"=1003.3594}, {"X"=228.16043, "Y"=1010.51}, {"X"=240.16873, "Y"=1020.7733}, {"X"=249.12323, "Y"=1030.9225}, {"X"=253.63432, "Y"=1031.0343}, {"X"=267.0481, "Y"=1041.2557}, {"X"=272.87646, "Y"=1054.5256}, {"X"=274.3735, "Y"=1054.5627}, {"X"=277.60156, "Y"=1038.2255}, {"X"=280.26465, "Y"=1061.2463}, {"X"=283.10397, "Y"=1071.0908}, {"X"=308.3406, "Y"=1078.2144}, {"X"=324.12244, "Y"=1104.4216}, {"X"=335.65088, "Y"=1117.5175}, {"X"=354.21225, "Y"=1140.2383}, {"X"=369.98932, "Y"=1196.959}, {"X"=398.25793, "Y"=1219.233}, {"X"=431.77283, "Y"=1247.5258}, {"X"=449.7526, "Y"=1263.0964}, {"X"=455.97318, "Y"=1254.1978}, {"X"=453.0925, "Y"=1254.1245}, {"X"=422.22345, "Y"=1235.1246}, {"X"=407.89645, "Y"=1231.712}, {"X"=403.4331, "Y"=1234.6478}, {"X"=374.46454, "Y"=1193.9767}, {"X"=347.59354, "Y"=1165.2635}, {"X"=325.54123, "Y"=1167.8391}, {"X"=314.10565, "Y"=1155.0049}, {"X"=301.0188, "Y"=1148.3789}, {"X"=264.212, "Y"=1153.7504}, {"X"=236.22043, "Y"=1171.8374}, {"X"=205.53566, "Y"=1189.7101}, {"X"=186.67572, "Y"=1204.663}, {"X"=176.5019, "Y"=1201.3276}, {"X"=166.391, "Y"=1207.2236}, {"X"=173.63963, "Y"=1207.4071}, {"X"=198.27754, "Y"=1201.8784}, {"X"=215.6939, "Y"=1205.3972}, {"X"=224.41202, "Y"=1202.5394}, {"X"=253.758, "Y"=1172.2793}, {"X"=270.0811, "Y"=1153.898}, {"X"=265.83258, "Y"=1141.1824}, {"X"=294.12387, "Y"=1122.8561}, {"X"=330.94373, "Y"=1069.0278}, {"X"=364.84216, "Y"=1037.0918}, {"X"=386.04538, "Y"=990.99445}, {"X"=409.4883, "Y"=974.7101}, {"X"=427.27222, "Y"=951.3503}, {"X"=429.39905, "Y"=937.70386}, {"X"=434.61456, "Y"=924.0593}, {"X"=430.93353, "Y"=937.74146}, {"X"=422.16083, "Y"=927.20465}, {"X"=411.1236, "Y"=933.8203}, {"X"=394.2357, "Y"=933.40686}, {"X"=393.98392, "Y"=940.26764}, {"X"=379.3747, "Y"=963.7989}, {"X"=367.93945, "Y"=987.18494}, {"X"=347.63464, "Y"=1006.7955}, {"X"=348.48892, "Y"=1030.0792}, {"X"=340.69586, "Y"=1039.7903}, {"X"=341.57623, "Y"=1062.7711}, {"X"=339.2112, "Y"=1095.1494}, {"X"=338.78076, "Y"=1111.2002}, {"X"=341.8309, "Y"=1108.0725}, {"X"=378.6653, "Y"=1115.3981}, {"X"=403.83667, "Y"=1116.028}, {"X"=415.54797, "Y"=1119.5175}, {"X"=420.7746, "Y"=1135.5692}, {"X"=422.33307, "Y"=1167.145}, {"X"=441.8003, "Y"=1189.4734}, {"X"=445.87332, "Y"=1195.7802}, {"X"=435.08646, "Y"=1176.849}, {"X"=404.61734, "Y"=1169.8304}, {"X"=399.48157, "Y"=1188.4054}, {"X"=391.0807, "Y"=1178.8594}, {"X"=371.7795, "Y"=1143.8424}, {"X"=356.67368, "Y"=1156.0753}, {"X"=352.45718, "Y"=1149.6714}, {"X"=356.96375, "Y"=1146.6295}, {"X"=361.5761, "Y"=1140.4231}, {"X"=380.72363, "Y"=1140.9037}, {"X"=208.53722, "Y"=1013.3511}, {"X"=223.65552, "Y"=1003.7327}, {"X"=222.24083, "Y"=973.4826}, {"X"=231.38031, "Y"=970.32794}, {"X"=238.98792, "Y"=970.51514}, {"X"=260.32715, "Y"=967.65576}, {"X"=260.00394, "Y"=997.9465}, {"X"=270.47238, "Y"=1008.2249}, {"X"=274.95938, "Y"=1011.667}, {"X"=276.28394, "Y"=1024.9811}, {"X"=280.8017, "Y"=1025.0929}, {"X"=273.31644, "Y"=1021.5938}, {"X"=274.32883, "Y"=1057.8323}, {"X"=277.1815, "Y"=1067.6897}, {"X"=281.31738, "Y"=1090.4799}, {"X"=297.13657, "Y"=1119.7445}, {"X"=337.59012, "Y"=1155.5955}, {"X"=359.21725, "Y"=1168.6871}, {"X"=382.64545, "Y"=1209.6215}, {"X"=408.57596, "Y"=1249.9663}, {"X"=421.13837, "Y"=1259.353}, {"X"=421.13837, "Y"=1259.353}, {"X"=419.83426, "Y"=1256.3013}, {"X"=410.53098, "Y"=1237.8732}, {"X"=399.6048, "Y"=1185.301}, {"X"=379.719, "Y"=1169.2034}, {"X"=389.67972, "Y"=1137.9609}, {"X"=386.73175, "Y"=1137.887}, {"X"=387.97174, "Y"=1144.249}, {"X"=390.44217, "Y"=1156.9244}, {"X"=401.68793, "Y"=1169.7567}, {"X"=412.4824, "Y"=1191.8372}, {"X"=427.3975, "Y"=1216.9026}, {"X"=450.40164, "Y"=1192.7946}, {"X"=467.03964, "Y"=1236.2618}, {"X"=499.89105, "Y"=1267.3845}, {"X"=491.26862, "Y"=1267.1649}, {"X"=496.12518, "Y"=1258.242}, {"X"=481.67285, "Y"=1233.5834}, {"X"=442.0577, "Y"=1214.2012}, {"X"=399.2356, "Y"=1194.6023}, {"X"=351.80267, "Y"=1171.6273}, {"X"=310.10275, "Y"=1135.9644}, {"X"=275.46194, "Y"=1083.8728}, {"X"=239.90092, "Y"=1060.2424}, {"X"=205.52213, "Y"=1029.8419}, {"X"=170.7189, "Y"=995.7426}, {"X"=155.35674, "Y"=971.83636}, {"X"=145.99966, "Y"=951.266}, {"X"=139.72026, "Y"=937.4614}, {"X"=144.14467, "Y"=923.84625}, {"X"=139.54292, "Y"=923.73364}, {"X"=148.7848, "Y"=927.39764}, {"X"=173.4443, "Y"=948.53375}, {"X"=193.3223, "Y"=959.2269}, {"X"=207.03757, "Y"=973.1084}, {"X"=208.55264, "Y"=983.257}, {"X"=228.32251, "Y"=973.6323}, {"X"=261.7387, "Y"=977.83026}, {"X"=279.97662, "Y"=978.27936}, {"X"=292.0792, "Y"=981.9486}, {"X"=287.7934, "Y"=964.9421}, {"X"=285.95026, "Y"=985.1644}, {"X"=289.1515, "Y"=975.1296}, {"X"=289.04123, "Y"=981.8738}, {"X"=295.1764, "Y"=978.6536}, {"X"=305.42126, "Y"=999.06757}, {"X"=306.53677, "Y"=1019.0977}, {"X"=300.13254, "Y"=1038.7842}, {"X"=294.1818, "Y"=1035.34}, {"X"=283.60953, "Y"=1038.3744}, {"X"=264.39075, "Y"=1011.4057}, {"X"=219.15625, "Y"=990.2372}, {"X"=178.1367, "Y"=969.018}, {"X"=164.3654, "Y"=958.5153}, {"X"=149.08911, "Y"=954.74316}, {"X"=152.06702, "Y"=948.00903}, {"X"=153.52402, "Y"=941.21936}, {"X"=190.24263, "Y"=948.946}, {"X"=185.67462, "Y"=952.2401}, {"X"=200.94003, "Y"=956.0168}, {"X"=229.87471, "Y"=966.90686}, {"X"=248.08952, "Y"=974.11884}, {"X"=265.94003, "Y"=1008.11285}, {"X"=270.47238, "Y"=1008.2249}, {"X"=268.63107, "Y"=1034.7065}, {"X"=274.46298, "Y"=1048.0109}, {"X"=291.83398, "Y"=1084.2811}, {"X"=294.46606, "Y"=1103.6804}, {"X"=295.65863, "Y"=1119.7075}, {"X"=308.36618, "Y"=1148.5635}, {"X"=331.63824, "Y"=1158.5885}, {"X"=372.584, "Y"=1206.2871}, {"X"=388.17648, "Y"=1255.496}, {"X"=389.61536, "Y"=1255.5325}, {"X"=389.84613, "Y"=1249.4902}, {"X"=376.0813, "Y"=1230.905}, {"X"=356.7896, "Y"=1199.7168}, {"X"=348.6029, "Y"=1180.9033}, {"X"=356.3847, "Y"=1165.4849}, {"X"=363.1499, "Y"=1137.2953}, {"X"=374.5503, "Y"=1105.6821}, {"X"=389.68442, "Y"=1057.4283}, {"X"=398.79898, "Y"=1054.3787}, {"X"=396.9244, "Y"=1024.6534}, {"X"=412.68454, "Y"=1008.4024}, {"X"=413.91953, "Y"=978.20056}, {"X"=422.53665, "Y"=954.6473}, {"X"=328.5394, "Y"=982.8468}, {"X"=332.7613, "Y"=996.39294}, {"X"=326.8598, "Y"=989.5353}, {"X"=320.63885, "Y"=996.0939}, {"X"=314.43454, "Y"=1002.6349}, {"X"=308.5851, "Y"=992.4428}, {"X"=288.43994, "Y"=1018.6499}, {"X"=285.26746, "Y"=1028.5131}, {"X"=273.00784, "Y"=1044.6913}, {"X"=286.1407, "Y"=1067.9126}, {"X"=278.5328, "Y"=1077.4716}, {"X"=285.5187, "Y"=1106.6644}, {"X"=310.641, "Y"=1110.4963}, {"X"=334.4898, "Y"=1161.799}, {"X"=369.98932, "Y"=1196.959}, {"X"=396.3266, "Y"=1231.4186}, {"X"=416.17657, "Y"=1241.058}, {"X"=413.15894, "Y"=1244.019}, {"X"=408.8309, "Y"=1243.909}, {"X"=402.48328, "Y"=1222.4045}, {"X"=399.85168, "Y"=1179.0804}, {"X"=387.97174, "Y"=1144.249}, {"X"=386.73175, "Y"=1137.887}, {"X"=386.65167, "Y"=1099.5549}, {"X"=380.3545, "Y"=1066.9987}, {"X"=365.05084, "Y"=1030.4895}, {"X"=357.72183, "Y"=1023.6831}, {"X"=346.12213, "Y"=1006.7581}, {"X"=342.8491, "Y"=959.50256}, {"X"=346.1823, "Y"=949.3609}, {"X"=339.5292, "Y"=969.60364}, {"X"=331.99576, "Y"=966.02875}, {"X"=330.3886, "Y"=969.37885}, {"X"=332.7613, "Y"=996.39294}, {"X"=335.62064, "Y"=1003.158}, {"X"=326.93582, "Y"=1049.3138}, {"X"=332.93375, "Y"=1049.4628}, {"X"=340.87207, "Y"=1088.7372}, {"X"=339.82947, "Y"=1127.1846}, {"X"=341.21878, "Y"=1130.3987}, {"X"=308.16962, "Y"=1157.9982}, {"X"=266.79596, "Y"=1181.9504}, {"X"=231.60728, "Y"=1215.0118}, {"X"=208.41856, "Y"=1244.8783}, {"X"=198.3402, "Y"=1241.594}, {"X"=189.70074, "Y"=1241.3745}, {"X"=192.58052, "Y"=1241.4476}, {"X"=196.88316, "Y"=1232.45}, {"X"=211.30356, "Y"=1238.8915}, {"X"=220.00256, "Y"=1220.8396}, {"X"=237.36137, "Y"=1221.2797}, {"X"=241.70134, "Y"=1221.3896}, {"X"=235.97157, "Y"=1212.0555}, {"X"=231.62352, "Y"=1211.9454}, {"X"=389.02356, "Y"=1034.3895}, {"X"=387.39957, "Y"=1037.6511}, {"X"=388.11642, "Y"=1017.7926}, {"X"=381.6082, "Y"=987.5218}, {"X"=375.8707, "Y"=977.26404}, {"X"=362.07162, "Y"=980.30084}, {"X"=340.6053, "Y"=986.5113}, {"X"=326.93988, "Y"=986.17456}, {"X"=322.30792, "Y"=989.42303}, {"X"=316.16602, "Y"=992.62976}, {"X"=302.26584, "Y"=1005.6747}, {"X"=277.88437, "Y"=1018.38873}, {"X"=265.66452, "Y"=1031.3324}, {"X"=260.9726, "Y"=1047.6759}, {"X"=253.29268, "Y"=1067.0951}, {"X"=259.36896, "Y"=1057.4604}, {"X"=257.80536, "Y"=1063.9497}, {"X"=256.34424, "Y"=1060.6514}, {"X"=262.25058, "Y"=1067.318}, {"X"=262.25058, "Y"=1067.318}, {"X"=259.3341, "Y"=1060.7258}, {"X"=265.15952, "Y"=1073.8933}, {"X"=196.49641, "Y"=1026.314}, {"X"=194.97781, "Y"=1019.6547}, {"X"=200.97972, "Y"=996.48956}, {"X"=225.19228, "Y"=997.0872}, {"X"=239.05385, "Y"=960.3507}, {"X"=254.36487, "Y"=953.9267}, {"X"=268.1477, "Y"=950.85803}, {"X"=280.47073, "Y"=944.3325}, {"X"=294.30075, "Y"=941.2507}, {"X"=306.28275, "Y"=955.2015}, {"X"=316.3851, "Y"=982.54736}, {"X"=322.23096, "Y"=992.77936}, {"X"=326.38156, "Y"=1009.60657}, {"X"=336.78857, "Y"=1016.52313}, {"X"=328.75656, "Y"=1036.1971}, {"X"=308.3406, "Y"=1078.2144}, {"X"=292.53537, "Y"=1129.1781}, {"X"=278.6988, "Y"=1166.6594}, {"X"=269.79498, "Y"=1175.8016}, {"X"=227.39763, "Y"=1184.0623}, {"X"=189.54616, "Y"=1195.4897}, {"X"=166.3409, "Y"=1201.0706}, {"X"=142.07132, "Y"=1231.0586}, {"X"=129.23701, "Y"=1239.838}, {"X"=134.94994, "Y"=1236.9519}, {"X"=151.82625, "Y"=1200.7035}, {"X"=182.30846, "Y"=1201.4745}, {"X"=189.4835, "Y"=1176.8904}, {"X"=226.08089, "Y"=1149.6458}, {"X"=267.66003, "Y"=1112.6204}, {"X"=313.88174, "Y"=1097.7374}, {"X"=355.65466, "Y"=1092.3351}, {"X"=378.07388, "Y"=1089.6652}, {"X"=386.21725, "Y"=1070.4034}, {"X"=396.67642, "Y"=1070.6638}, {"X"=402.26962, "Y"=1080.5549}, {"X"=407.97235, "Y"=1087.1772}, {"X"=402.0146, "Y"=1087.0287}, {"X"=383.1136, "Y"=1073.5809}, {"X"=358.12875, "Y"=1059.9156}, {"X"=356.53363, "Y"=1063.1431}, {"X"=357.8313, "Y"=1069.697}, {"X"=369.03253, "Y"=1047.0748}, {"X"=384.97882, "Y"=1021.0386}, {"X"=410.06244, "Y"=998.30023}, {"X"=446.36594, "Y"=968.8404}, {"X"=465.1897, "Y"=959.1032}, {"X"=480.228, "Y"=935.5122}, {"X"=488.66534, "Y"=921.9258}, {"X"=494.63226, "Y"=925.52686}, {"X"=488.66534, "Y"=921.9258}, {"X"=476.163, "Y"=925.07526}, {"X"=465.91348, "Y"=914.44586}, {"X"=466.57938, "Y"=931.73694}, {"X"=448.3003, "Y"=927.8441}, {"X"=413.9158, "Y"=940.756}, {"X"=401.12778, "Y"=954.1218}, {"X"=400.0921, "Y"=981.23706}, {"X"=384.40942, "Y"=994.3129}, {"X"=354.41376, "Y"=1033.5317}, {"X"=335.3404, "Y"=1072.3914}, {"X"=315.15436, "Y"=1107.4054}, {"X"=303.9577, "Y"=1148.4528}, {"X"=282.84424, "Y"=1182.3553}, {"X"=272.1261, "Y"=1219.1014}, {"X"=257.453, "Y"=1237.0275}, {"X"=248.55836, "Y"=1263.9902}, {"X"=245.6406, "Y"=1269.9163}, {"X"=245.6406, "Y"=1269.9163}, {"X"=235.74547, "Y"=1248.5975}, {"X"=241.29971, "Y"=1275.7909}, {"X"=239.93292, "Y"=1266.7725}, {"X"=241.36603, "Y"=1266.809}, {"X"=262.971, "Y"=1258.3417}, {"X"=261.7097, "Y"=1243.2043}, {"X"=260.4061, "Y"=1231.0186}, {"X"=249.48448, "Y"=1159.6599}, {"X"=254.2197, "Y"=1125.0391}, {"X"=260.15732, "Y"=1122.0052}, {"X"=266.25833, "Y"=1106.1829}, {"X"=272.14157, "Y"=1109.5333}, {"X"=279.44968, "Y"=1116.1106}, {"X"=316.27966, "Y"=1123.4111}, {"X"=342.25565, "Y"=1146.2601}, {"X"=378.14453, "Y"=1172.2909}, {"X"=410.24466, "Y"=1210.3198}, {"X"=424.21927, "Y"=1222.9553}, {"X"=434.3637, "Y"=1223.2123}, {"X"=442.61075, "Y"=1232.5925}, {"X"=437.40848, "Y"=1220.2247}, {"X"=424.42682, "Y"=1185.9272}, {"X"=409.5317, "Y"=1157.4044}, {"X"=403.45407, "Y"=1125.5951}, {"X"=395.07437, "Y"=1112.6083}, {"X"=389.50363, "Y"=1102.8431}, {"X"=387.66623, "Y"=1112.423}, {"X"=383.10706, "Y"=1115.5093}, {"X"=382.3099, "Y"=1137.776}, {"X"=392.7807, "Y"=1172.6597}, {"X"=403.9849, "Y"=1185.4115}, {"X"=412.6264, "Y"=1222.6615}, {"X"=426.56, "Y"=1235.2347}, {"X"=432.92935, "Y"=1253.6118}, {"X"=428.32968, "Y"=1259.5361}, {"X"=407.76917, "Y"=1234.7578}, {"X"=383.08807, "Y"=1237.1766}, {"X"=377.2033, "Y"=1240.0684}, {"X"=359.4075, "Y"=1209.0334}, {"X"=342.67392, "Y"=1183.8647}, {"X"=324.30392, "Y"=1158.404}, {"X"=318.8702, "Y"=1139.3512}, {"X"=295.19833, "Y"=1145.0781}, {"X"=276.13007, "Y"=1141.4409}, {"X"=246.68422, "Y"=1143.8596}, {"X"=221.6072, "Y"=1171.4691}, {"X"=212.83546, "Y"=1174.3657}, {"X"=193.93741, "Y"=1207.9209}, {"X"=182.36821, "Y"=1213.7646}, {"X"=173.80232, "Y"=1231.8641}, {"X"=173.84274, "Y"=1237.9398}, {"X"=173.94334, "Y"=1253.0627}, {"X"=170.93947, "Y"=1234.8307}, {"X"=160.62102, "Y"=1210.1476}, {"X"=170.42552, "Y"=1163.9329}, {"X"=164.44243, "Y"=1148.0964}, {"X"=162.78163, "Y"=1125.9252}, {"X"=165.4953, "Y"=1097.2462}, {"X"=-423.1004, "Y"=-1143.6017}] {"Y" format="%.2f"; "X" format="%.2f"}
  in  "auto top huyun vs chen jin":T1[](array[typedef])=[{"X"=282.4219, "Y"=278.37894}, {"X"=283.99814, "Y"=270.1361}, {"X"=285.7254, "Y"=282.59555}, {"X"=288.99704, "Y"=282.67883}, {"X"=289.18375, "Y"=311.44147}, {"X"=303.93893, "Y"=340.27393}, {"X"=310.41287, "Y"=340.4338}, {"X"=321.69785, "Y"=283.5111}, {"X"=329.84244, "Y"=320.61963}, {"X"=336.37338, "Y"=300.34323}, {"X"=334.69302, "Y"=332.93396}, {"X"=341.27118, "Y"=296.3614}, {"X"=354.49554, "Y"=259.48352}, {"X"=376.17816, "Y"=218.1293}, {"X"=388.05508, "Y"=188.73854}, {"X"=394.7934, "Y"=180.37607}, {"X"=396.45474, "Y"=180.42064}, {"X"=403.04236, "Y"=184.87138}, {"X"=408.38773, "Y"=159.2772}, {"X"=406.30237, "Y"=189.22614}, {"X"=379.5199, "Y"=213.99222}, {"X"=359.61276, "Y"=226.12688}, {"X"=356.33603, "Y"=221.82701}, {"X"=351.45844, "Y"=204.7798}, {"X"=344.6675, "Y"=255.0647}, {"X"=341.2936, "Y"=288.13318}, {"X"=339.6212, "Y"=304.52475}, {"X"=336.37338, "Y"=300.34323}, {"X"=344.4903, "Y"=308.74072}, {"X"=344.5853, "Y"=279.96445}, {"X"=341.3726, "Y"=259.14523}, {"X"=339.74207, "Y"=254.93745}, {"X"=343.06354, "Y"=242.48997}, {"X"=361.31433, "Y"=217.73795}, {"X"=386.48544, "Y"=180.15314}, {"X"=401.8321, "Y"=150.46849}, {"X"=405.17145, "Y"=150.55942}, {"X"=427.32297, "Y"=125.12354}, {"X"=429.30823, "Y"=107.689125}, {"X"=420.97324, "Y"=103.0682}, {"X"=415.3876, "Y"=137.84518}, {"X"=388.37863, "Y"=158.73463}, {"X"=361.52432, "Y"=183.75963}, {"X"=351.59134, "Y"=174.9336}, {"X"=344.9044, "Y"=183.31459}, {"X"=344.8903, "Y"=187.58513}, {"X"=339.8033, "Y"=229.81618}, {"X"=333.16312, "Y"=263.0936}, {"X"=328.26282, "Y"=216.86769}, {"X"=333.15778, "Y"=267.2474}, {"X"=331.5067, "Y"=279.63086}, {"X"=347.98315, "Y"=246.80148}, {"X"=348.0808, "Y"=221.6101}, {"X"=343.03833, "Y"=250.85095}, {"X"=347.98315, "Y"=246.80148}, {"X"=369.5406, "Y"=222.17397}, {"X"=381.49982, "Y"=180.01935}, {"X"=391.6653, "Y"=163.13019}, {"X"=391.91055, "Y"=141.54048}, {"X"=389.9037, "Y"=171.67642}, {"X"=393.4321, "Y"=154.55891}, {"X"=395.2041, "Y"=145.9625}, {"X"=391.76318, "Y"=154.51357}, {"X"=386.21732, "Y"=205.70082}, {"X"=372.63467, "Y"=247.44101}, {"X"=367.61395, "Y"=259.8217}, {"X"=362.93887, "Y"=222.0005}, {"X"=362.69507, "Y"=259.6949}, {"X"=369.44446, "Y"=234.79256}, {"X"=369.63715, "Y"=209.49959}, {"X"=369.44446, "Y"=234.79256}, {"X"=384.4333, "Y"=218.34666}, {"X"=401.10422, "Y"=206.09529}, {"X"=409.86743, "Y"=172.21437}, {"X"=411.72156, "Y"=159.3676}, {"X"=408.88113, "Y"=124.61504}, {"X"=415.18777, "Y"=150.83215}, {"X"=391.6165, "Y"=167.42891}, {"X"=379.71814, "Y"=192.77841}, {"X"=354.79153, "Y"=200.62294}, {"X"=328.26462, "Y"=212.6398}, {"X"=319.9825, "Y"=203.94577}, {"X"=308.40527, "Y"=212.1158}, {"X"=298.53207, "Y"=224.52539}, {"X"=287.1076, "Y"=245.22218}, {"X"=282.32684, "Y"=265.94263}, {"X"=269.03226, "Y"=248.93507}, {"X"=262.49335, "Y"=252.94186}, {"X"=262.6782, "Y"=269.59}, {"X"=242.98763, "Y"=269.08566}, {"X"=226.3532, "Y"=256.1802}, {"X"=199.4593, "Y"=230.3545}, {"X"=183.7344, "Y"=196.08083}, {"X"=162.91177, "Y"=165.55975}, {"X"=159.06755, "Y"=148.19046}, {"X"=153.38657, "Y"=126.307274}, {"X"=148.19608, "Y"=121.7992}, {"X"=147.66214, "Y"=104.25673}, {"X"=158.44339, "Y"=126.44613}, {"X"=161.56833, "Y"=117.79584}, {"X"=161.69138, "Y"=122.17053}, {"X"=170.1235, "Y"=122.40255}, {"X"=191.45981, "Y"=170.62762}, {"X"=200.00354, "Y"=179.43451}, {"X"=220.49126, "Y"=205.55595}, {"X"=232.04329, "Y"=201.61563}, {"X"=253.95053, "Y"=227.56995}, {"X"=265.73975, "Y"=248.84984}, {"X"=265.73975, "Y"=248.84984}, {"X"=262.354, "Y"=240.39168}, {"X"=262.26074, "Y"=231.99416}, {"X"=260.7528, "Y"=244.53845}, {"X"=240.7877, "Y"=231.43353}, {"X"=204.06311, "Y"=213.59749}, {"X"=180.40529, "Y"=195.99243}, {"X"=162.05942, "Y"=135.2554}, {"X"=158.44339, "Y"=126.44613}, {"X"=153.38657, "Y"=126.307274}, {"X"=149.61922, "Y"=113.087814}, {"X"=163.62096, "Y"=130.94644}, {"X"=187.2934, "Y"=135.9454}, {"X"=202.24112, "Y"=127.64875}, {"X"=210.83005, "Y"=136.58899}, {"X"=227.92549, "Y"=154.3837}, {"X"=262.02646, "Y"=210.89206}, {"X"=277.1196, "Y"=232.3821}, {"X"=288.50806, "Y"=207.35442}, {"X"=315.0421, "Y"=220.74203}, {"X"=320.0126, "Y"=233.50197}, {"X"=326.60892, "Y"=221.04594}, {"X"=358.24887, "Y"=175.11261}, {"X"=393.2817, "Y"=167.47388}, {"X"=406.66068, "Y"=163.53596}, {"X"=413.4534, "Y"=155.10297}, {"X"=428.84518, "Y"=133.87096}, {"X"=431.8758, "Y"=151.28658}, {"X"=426.87018, "Y"=151.15027}, {"X"=418.1142, "Y"=176.7224}, {"X"=399.4504, "Y"=206.05147}, {"X"=384.34726, "Y"=226.7754}, {"X"=379.55942, "Y"=209.76195}, {"X"=377.86758, "Y"=213.94862}, {"X"=374.45538, "Y"=226.51604}, {"X"=369.22177, "Y"=264.02118}, {"X"=370.76166, "Y"=276.4983}, {"X"=367.67505, "Y"=251.48875}, {"X"=378.70294, "Y"=301.41138}, {"X"=403.2145, "Y"=293.8198}, {"X"=406.706, "Y"=277.41702}, {"X"=420.18, "Y"=252.848}, {"X"=420.31805, "Y"=244.49844}, {"X"=435.4142, "Y"=228.11433}, {"X"=447.74084, "Y"=190.33342}, {"X"=451.42493, "Y"=173.33421}, {"X"=458.36435, "Y"=160.6324}, {"X"=469.41733, "Y"=117.55736}, {"X"=493.7635, "Y"=87.490295}, {"X"=488.46515, "Y"=96.15827}, {"X"=428.51633, "Y"=335.26126}, {"X"=399.31772, "Y"=342.62964}, {"X"=396.139, "Y"=338.50754}, {"X"=392.66663, "Y"=358.58237}, {"X"=397.29193, "Y"=374.71936}, {"X"=397.65146, "Y"=346.62616}, {"X"=391.1501, "Y"=350.49817}, {"X"=379.977, "Y"=338.1075}, {"X"=363.75345, "Y"=345.79074}, {"X"=357.00192, "Y"=397.61826}, {"X"=350.53006, "Y"=413.26935}, {"X"=345.71365, "Y"=421.02487}, {"X"=339.36636, "Y"=409.0605}, {"X"=350.3386, "Y"=456.272}, {"X"=339.21417, "Y"=471.49036}, {"X"=329.73, "Y"=478.97888}, {"X"=332.8854, "Y"=479.05106}, {"X"=329.73, "Y"=478.97888}, {"X"=328.14572, "Y"=494.29117}, {"X"=321.85715, "Y"=501.79123}, {"X"=323.4252, "Y"=494.1841}, {"X"=326.57126, "Y"=501.89767}, {"X"=207.04022, "Y"=354.03705}, {"X"=202.13083, "Y"=200.82303}, {"X"=204.90033, "Y"=329.71442}, {"X"=202.00755, "Y"=345.8467}, {"X"=197.69905, "Y"=369.87418}, {"X"=195.03401, "Y"=393.73734}, {"X"=191.6058, "Y"=317.1685}, {"X"=191.7029, "Y"=321.24884}, {"X"=194.8642, "Y"=317.24982}, {"X"=211.48306, "Y"=333.93698}, {"X"=213.10675, "Y"=333.97717}, {"X"=217.89954, "Y"=330.03687}, {"X"=227.21884, "Y"=305.79407}, {"X"=233.81015, "Y"=310.0531}, {"X"=233.9433, "Y"=318.22546}, {"X"=233.9433, "Y"=318.22546}, {"X"=240.39078, "Y"=314.3052}, {"X"=241.77568, "Y"=297.9561}, {"X"=246.38605, "Y"=277.4598}, {"X"=258.29852, "Y"=314.75323}, {"X"=264.94055, "Y"=327.14148}, {"X"=286.3292, "Y"=368.02255}, {"X"=318.55096, "Y"=376.80365}, {"X"=336.20798, "Y"=389.18158}, {"X"=369.77032, "Y"=401.88318}, {"X"=372.0264, "Y"=321.6728}, {"X"=381.79492, "Y"=317.84305}, {"X"=376.67053, "Y"=346.1091}, {"X"=390.59192, "Y"=398.4231}, {"X"=383.989, "Y"=417.99988}, {"X"=380.8802, "Y"=410.0487}, {"X"=378.43613, "Y"=329.9628}, {"X"=375.5205, "Y"=293.11795}, {"X"=378.8952, "Y"=280.8395}, {"X"=378.55014, "Y"=317.76184}, {"X"=373.75174, "Y"=309.47598}, {"X"=377.15015, "Y"=293.15927}, {"X"=377.15015, "Y"=293.15927}, {"X"=387.05966, "Y"=281.04776}, {"X"=395.42474, "Y"=264.6952}, {"X"=424.17764, "Y"=210.94173}, {"X"=434.40524, "Y"=194.23665}, {"X"=449.2152, "Y"=198.88402}, {"X"=467.92996, "Y"=178.06195}, {"X"=485.942, "Y"=126.73985}, {"X"=495.70325, "Y"=78.70221}, {"X"=468.08447, "Y"=33.290745}, {"X"=501.78864, "Y"=100.928734}, {"X"=499.3382, "Y"=69.93588}, {"X"=506.5585, "Y"=109.83696}, {"X"=507.6917, "Y"=127.33956}, {"X"=495.19348, "Y"=96.34651}, {"X"=475.00858, "Y"=161.08372}, {"X"=470.01608, "Y"=160.94835}, {"X"=198.94891, "Y"=353.83893}, {"X"=200.5673, "Y"=353.87857}, {"X"=199.22208, "Y"=365.9034}, {"X"=192.28253, "Y"=345.60754}, {"X"=192.37866, "Y"=349.64688}, {"X"=191.216, "Y"=300.7878}, {"X"=182.91536, "Y"=229.92258}, {"X"=191.6058, "Y"=317.1685}, {"X"=194.37694, "Y"=365.78552}, {"X"=203.89159, "Y"=357.98474}, {"X"=215.68417, "Y"=382.2971}, {"X"=220.05876, "Y"=358.37976}, {"X"=242.74097, "Y"=362.95093}, {"X"=271.70877, "Y"=355.62054}, {"X"=281.39957, "Y"=355.85785}, {"X"=290.96265, "Y"=335.90424}, {"X"=312.06094, "Y"=352.5838}, {"X"=312.07083, "Y"=356.6089}, {"X"=331.44553, "Y"=340.95328}, {"X"=349.06613, "Y"=381.53125}, {"X"=371.36884, "Y"=401.9214}, {"X"=393.5483, "Y"=418.22644}, {"X"=409.41583, "Y"=422.53137}, {"X"=430.28235, "Y"=327.19235}, {"X"=447.86548, "Y"=261.89044}, {"X"=428.37732, "Y"=253.06021}, {"X"=436.00955, "Y"=282.29626}, {"X"=442.53143, "Y"=282.4626}, {"X"=412.414, "Y"=434.35504}, {"X"=406.06262, "Y"=434.2058}, {"X"=402.71255, "Y"=330.56628}, {"X"=401.94455, "Y"=386.78928}, {"X"=404.866, "Y"=406.6738}, {"X"=403.215, "Y"=410.58038}, {"X"=396.88544, "Y"=406.4834}, {"X"=389.49173, "Y"=354.4839}, {"X"=380.40915, "Y"=293.24185}, {"X"=369.4125, "Y"=238.98643}, {"X"=344.8201, "Y"=208.8434}, {"X"=341.4639, "Y"=225.65103}, {"X"=305.06378, "Y"=203.55048}, {"X"=296.557, "Y"=160.55658}, {"X"=256.07693, "Y"=129.127}, {"X"=238.60919, "Y"=84.74836}, {"X"=231.90092, "Y"=88.98029}, {"X"=225.04991, "Y"=84.368225}, {"X"=207.64864, "Y"=61.673153}, {"X"=179.40323, "Y"=20.459467}, {"X"=149.32233, "Y"=46.605637}, {"X"=136.08093, "Y"=59.645847}, {"X"=168.35425, "Y"=56.096165}, {"X"=142.34697, "Y"=41.92109}, {"X"=150.89842, "Y"=42.165337}, {"X"=190.2515, "Y"=118.58672}, {"X"=206.05612, "Y"=149.4673}, {"X"=236.23245, "Y"=150.2873}, {"X"=278.31668, "Y"=177.25055}, {"X"=288.4253, "Y"=194.60553}, {"X"=306.76392, "Y"=216.30162}, {"X"=329.89816, "Y"=242.14769}, {"X"=361.05533, "Y"=259.65262}, {"X"=380.17258, "Y"=317.80246}, {"X"=396.29117, "Y"=326.34555}, {"X"=394.17877, "Y"=366.6431}, {"X"=387.9694, "Y"=346.38754}, {"X"=371.56412, "Y"=378.08777}, {"X"=369.89575, "Y"=386.01633}, {"X"=360.34976, "Y"=373.82257}, {"X"=344.36957, "Y"=345.31302}, {"X"=333.03186, "Y"=365.15228}, {"X"=329.79105, "Y"=392.99954}, {"X"=324.98624, "Y"=412.6626}, {"X"=318.56656, "Y"=388.75702}, {"X"=307.243, "Y"=360.50998}, {"X"=297.8271, "Y"=412.0175}, {"X"=280.30792, "Y"=419.47806}, {"X"=262.87506, "Y"=430.84167}, {"X"=265.49557, "Y"=523.3359}, {"X"=245.28468, "Y"=534.2259}, {"X"=226.77835, "Y"=548.86707}, {"X"=192.15302, "Y"=600.1579}, {"X"=152.96416, "Y"=632.278}, {"X"=138.99051, "Y"=539.418}, {"X"=142.05908, "Y"=628.40906}, {"X"=132.94286, "Y"=631.86127}, {"X"=132.94286, "Y"=631.86127}, {"X"=280.81744, "Y"=282.47064}, {"X"=282.4219, "Y"=278.37894}, {"X"=285.66693, "Y"=274.3233}, {"X"=288.9702, "Y"=278.54593}, {"X"=292.58295, "Y"=335.94434}, {"X"=303.92316, "Y"=336.22504}, {"X"=310.39062, "Y"=332.33112}, {"X"=326.59888, "Y"=295.99036}, {"X"=329.85114, "Y"=308.3729}, {"X"=336.2006, "Y"=393.15344}, {"X"=353.74167, "Y"=409.40268}, {"X"=377.39526, "Y"=441.34335}, {"X"=407.13293, "Y"=469.1939}, {"X"=421.13022, "Y"=481.07028}, {"X"=430.49945, "Y"=485.12473}, {"X"=425.71173, "Y"=488.85028}, {"X"=423.11353, "Y"=457.95944}, {"X"=421.39832, "Y"=465.66034}, {"X"=415.20996, "Y"=457.77618}, {"X"=407.82455, "Y"=422.49374}, {"X"=397.03735, "Y"=394.61432}, {"X"=381.43338, "Y"=354.28616}, {"X"=375.05615, "Y"=346.0693}, {"X"=368.75217, "Y"=325.6595}, {"X"=359.12384, "Y"=309.10843}, {"X"=354.34982, "Y"=288.46478}, {"X"=344.5717, "Y"=284.09326}, {"X"=341.33865, "Y"=271.60486}, {"X"=346.2793, "Y"=263.431}, {"X"=359.36652, "Y"=267.92017}, {"X"=372.77203, "Y"=230.67876}, {"X"=370.92578, "Y"=255.74303}, {"X"=378.58826, "Y"=313.6831}, {"X"=386.61765, "Y"=322.03708}, {"X"=393.63925, "Y"=277.08304}, {"X"=385.0822, "Y"=313.84592}, {"X"=370.5016, "Y"=309.39432}, {"X"=361.00397, "Y"=267.9622}, {"X"=353.03415, "Y"=221.74026}, {"X"=354.53745, "Y"=251.14865}, {"X"=356.06937, "Y"=271.98218}, {"X"=362.61453, "Y"=272.1498}, {"X"=372.5322, "Y"=259.94846}, {"X"=372.49814, "Y"=264.10544}, {"X"=390.6549, "Y"=252.08365}, {"X"=420.94437, "Y"=206.62099}, {"X"=432.7492, "Y"=194.19249}, {"X"=437.7997, "Y"=190.06778}, {"X"=448.102, "Y"=173.24466}, {"X"=448.2834, "Y"=164.66226}, {"X"=442.0579, "Y"=142.91173}, {"X"=434.88818, "Y"=168.59738}, {"X"=407.96075, "Y"=189.27045}, {"X"=384.60614, "Y"=201.41461}, {"X"=366.359, "Y"=205.17462}, {"X"=359.7873, "Y"=196.50441}, {"X"=353.15463, "Y"=196.32793}, {"X"=344.69507, "Y"=246.71617}, {"X"=329.88336, "Y"=263.00925}, {"X"=315.08954, "Y"=245.94812}, {"X"=311.84985, "Y"=266.70047}, {"X"=305.27615, "Y"=262.37625}, {"X"=293.74045, "Y"=253.74908}, {"X"=260.94302, "Y"=261.23584}, {"X"=232.52562, "Y"=231.21782}, {"X"=212.02019, "Y"=196.83191}, {"X"=199.62923, "Y"=162.24464}, {"X"=197.76501, "Y"=153.56586}, {"X"=181.92535, "Y"=122.72729}, {"X"=190.5556, "Y"=131.6845}, {"X"=178.33284, "Y"=113.881195}, {"X"=191.83765, "Y"=114.25434}, {"X"=190.2515, "Y"=118.58672}, {"X"=200.09677, "Y"=183.71605}, {"X"=215.75339, "Y"=218.13326}, {"X"=220.80133, "Y"=222.48737}, {"X"=239.0717, "Y"=227.18065}, {"X"=255.91173, "Y"=252.77185}, {"X"=267.55673, "Y"=265.5635}, {"X"=265.78372, "Y"=253.02687}, {"X"=260.6573, "Y"=236.153}, {"X"=262.44696, "Y"=248.7646}, {"X"=260.84805, "Y"=252.89937}, {"X"=232.59412, "Y"=235.42188}, {"X"=205.63318, "Y"=209.40407}, {"X"=199.34702, "Y"=149.28499}, {"X"=185.5068, "Y"=131.54614}, {"X"=183.82373, "Y"=131.50003}, {"X"=183.3977, "Y"=114.02114}, {"X"=176.64441, "Y"=113.83454}, {"X"=182.24794, "Y"=135.80743}, {"X"=191.05943, "Y"=153.38403}, {"X"=201.58008, "Y"=175.19142}, {"X"=208.34615, "Y"=179.6579}, {"X"=214.93669, "Y"=175.54982}, {"X"=221.33957, "Y"=251.87874}, {"X"=232.04437, "Y"=301.8159}, {"X"=234.07608, "Y"=326.3742}, {"X"=239.8304, "Y"=277.2926}, {"X"=245.21718, "Y"=310.33908}, {"X"=253.31044, "Y"=306.44968}, {"X"=272.36362, "Y"=253.19685}, {"X"=278.73566, "Y"=228.21841}, {"X"=278.77023, "Y"=232.4252}, {"X"=303.4223, "Y"=207.74876}, {"X"=341.5912, "Y"=178.94844}, {"X"=361.68344, "Y"=158.01074}, {"X"=373.43564, "Y"=149.69524}, {"X"=383.5462, "Y"=141.31177}, {"X"=398.65494, "Y"=137.38669}, {"X"=397.14078, "Y"=124.29132}, {"X"=391.56772, "Y"=171.72125}, {"X"=369.76657, "Y"=192.51305}, {"X"=359.81238, "Y"=192.24762}, {"X"=358.20093, "Y"=183.67064}, {"X"=351.36435, "Y"=225.91061}, {"X"=339.75223, "Y"=250.76588}, {"X"=324.96512, "Y"=275.32776}, {"X"=313.48935, "Y"=266.74255}, {"X"=284.15015, "Y"=290.8024}, {"X"=242.3214, "Y"=334.7003}, {"X"=230.75703, "Y"=322.22174}, {"X"=213.18805, "Y"=338.0325}, {"X"=193.99849, "Y"=349.6866}, {"X"=190.75874, "Y"=349.60712}, {"X"=192.18628, "Y"=341.56238}, {"X"=191.79985, "Y"=325.3233}, {"X"=194.8642, "Y"=317.24982}, {"X"=198.12233, "Y"=317.33118}, {"X"=208.91049, "Y"=366.1391}, {"X"=225.51477, "Y"=301.6515}, {"X"=240.08035, "Y"=293.8024}, {"X"=249.77428, "Y"=285.8089}, {"X"=254.6827, "Y"=285.93353}, {"X"=244.80627, "Y"=281.5541}, {"X"=238.76237, "Y"=314.26447}, {"X"=219.29333, "Y"=317.8597}, {"X"=195.33652, "Y"=337.59158}, {"X"=180.93355, "Y"=345.32846}, {"X"=169.2427, "Y"=332.89145}, {"X"=175.52725, "Y"=324.9188}, {"X"=183.56157, "Y"=321.04602}, {"X"=180.09367, "Y"=312.79663}, {"X"=200.29648, "Y"=341.76227}, {"X"=203.09782, "Y"=321.5327}, {"X"=209.8593, "Y"=333.8968}, {"X"=220.43738, "Y"=378.42224}, {"X"=223.00485, "Y"=429.90494}, {"X"=221.6309, "Y"=441.60498}, {"X"=215.4174, "Y"=449.25455}, {"X"=207.96484, "Y"=472.33594}, {"X"=193.98523, "Y"=483.57135}, {"X"=188.24002, "Y"=506.40897}, {"X"=157.78967, "Y"=539.8322}, {"X"=149.83539, "Y"=535.8879}, {"X"=145.13222, "Y"=535.78406}, {"X"=145.13222, "Y"=535.78406}, {"X"=127.74437, "Y"=531.6247}, {"X"=133.52489, "Y"=561.80756}, {"X"=125.72054, "Y"=561.63794}, {"X"=125.72054, "Y"=561.63794}] {"Y" format="%.2f"; "X" format="%.2f"}
  in  "manual top huyun vs chen jin":T1[](array[typedef])=[{"X"=282.4219, "Y"=278.37894}, {"X"=284.08948, "Y"=282.55392}, {"X"=282.548, "Y"=294.87637}, {"X"=282.4219, "Y"=278.37894}, {"X"=289.02383, "Y"=286.8057}, {"X"=298.77084, "Y"=274.65823}, {"X"=308.63342, "Y"=287.3037}, {"X"=311.95117, "Y"=307.92313}, {"X"=326.6022, "Y"=271.2274}, {"X"=334.82254, "Y"=250.63826}, {"X"=333.20612, "Y"=229.64357}, {"X"=341.52148, "Y"=204.5165}, {"X"=354.8987, "Y"=179.30554}, {"X"=379.63867, "Y"=201.2827}, {"X"=388.05508, "Y"=188.73854}, {"X"=405.05362, "Y"=159.1868}, {"X"=414.98886, "Y"=163.76132}, {"X"=413.58383, "Y"=146.46404}, {"X"=404.9361, "Y"=167.78857}, {"X"=391.76318, "Y"=154.51357}, {"X"=376.51352, "Y"=179.88554}, {"X"=358.1531, "Y"=192.20337}, {"X"=351.45844, "Y"=204.7798}, {"X"=349.71445, "Y"=225.86736}, {"X"=338.12704, "Y"=242.36163}, {"X"=334.8029, "Y"=263.13577}, {"X"=329.8745, "Y"=275.45322}, {"X"=323.33032, "Y"=279.4223}, {"X"=328.23987, "Y"=271.26935}, {"X"=341.39532, "Y"=250.80843}, {"X"=333.20612, "Y"=229.64357}, {"X"=341.4984, "Y"=212.98898}, {"X"=348.19586, "Y"=191.93787}, {"X"=365.02136, "Y"=158.10126}, {"X"=395.2041, "Y"=145.9625}, {"X"=410.49478, "Y"=129.01656}, {"X"=419.43088, "Y"=94.226875}, {"X"=429.69727, "Y"=85.690445}, {"X"=424.70917, "Y"=81.12822}, {"X"=419.36063, "Y"=98.627396}, {"X"=402.45908, "Y"=102.55237}, {"X"=377.00595, "Y"=123.73614}, {"X"=361.7101, "Y"=153.69693}, {"X"=353.33734, "Y"=157.78444}, {"X"=341.62625, "Y"=166.07901}, {"X"=336.56787, "Y"=195.88657}, {"X"=339.85477, "Y"=208.7121}, {"X"=328.2504, "Y"=246.28955}, {"X"=334.82913, "Y"=246.46022}, {"X"=336.4814, "Y"=242.31885}, {"X"=341.42953, "Y"=238.25739}, {"X"=341.44098, "Y"=234.06143}, {"X"=346.38425, "Y"=234.19049}, {"X"=346.4599, "Y"=213.1199}, {"X"=359.93835, "Y"=170.86896}, {"X"=383.1194, "Y"=184.33789}, {"X"=398.49243, "Y"=150.37755}, {"X"=400.4955, "Y"=124.38382}, {"X"=405.28964, "Y"=141.90633}, {"X"=407.08276, "Y"=133.27339}, {"X"=402.2299, "Y"=120.06762}, {"X"=395.51535, "Y"=119.88209}, {"X"=393.73495, "Y"=128.5554}, {"X"=380.0787, "Y"=154.19606}, {"X"=359.8375, "Y"=187.98453}, {"X"=349.8556, "Y"=191.98212}, {"X"=348.16287, "Y"=200.44693}, {"X"=354.70633, "Y"=217.56395}, {"X"=363.0757, "Y"=200.84291}, {"X"=368.13898, "Y"=188.20636}, {"X"=374.81503, "Y"=184.11552}, {"X"=386.57538, "Y"=171.58673}, {"X"=404.9361, "Y"=167.78857}, {"X"=415.3876, "Y"=137.84518}, {"X"=418.73325, "Y"=137.93686}, {"X"=413.71466, "Y"=137.79933}, {"X"=411.97745, "Y"=142.0892}, {"X"=400.1623, "Y"=150.42302}, {"X"=373.40024, "Y"=154.01459}, {"X"=343.25488, "Y"=178.99309}, {"X"=323.2838, "Y"=174.1724}, {"X"=315.00226, "Y"=199.5664}, {"X"=310.04898, "Y"=207.924}, {"X"=293.52777, "Y"=215.95311}, {"X"=295.22763, "Y"=224.43875}, {"X"=277.3687, "Y"=261.65836}, {"X"=275.65314, "Y"=253.28183}, {"X"=270.75906, "Y"=257.32492}, {"X"=265.60745, "Y"=236.28198}, {"X"=232.45702, "Y"=227.00758}, {"X"=198.89954, "Y"=204.98503}, {"X"=184.66817, "Y"=166.14601}, {"X"=164.10481, "Y"=148.32735}, {"X"=149.88326, "Y"=121.84563}, {"X"=149.75133, "Y"=117.47}, {"X"=146.23972, "Y"=112.99444}, {"X"=146.23972, "Y"=112.99444}, {"X"=140.89235, "Y"=104.06889}, {"X"=152.60852, "Y"=99.99587}, {"X"=152.60852, "Y"=99.99587}, {"X"=164.94394, "Y"=117.88891}, {"X"=183.50446, "Y"=118.40069}, {"X"=202.79343, "Y"=153.70221}, {"X"=214.93669, "Y"=175.54982}, {"X"=224.95108, "Y"=175.81856}, {"X"=241.88492, "Y"=193.36713}, {"X"=260.36902, "Y"=210.84833}, {"X"=272.08838, "Y"=223.83206}, {"X"=280.5206, "Y"=245.0513}, {"X"=275.5428, "Y"=240.73456}, {"X"=277.1196, "Y"=232.3821}, {"X"=253.52534, "Y"=193.67688}, {"X"=221.92159, "Y"=192.83592}, {"X"=186.13354, "Y"=157.56854}, {"X"=173.7237, "Y"=131.22328}, {"X"=166.27283, "Y"=104.7731}, {"X"=152.73868, "Y"=104.39758}, {"X"=146.10486, "Y"=108.60541}, {"X"=145.29144, "Y"=82.132164}, {"X"=174.50186, "Y"=96.20116}, {"X"=198.49278, "Y"=110.05593}, {"X"=206.9357, "Y"=110.2897}, {"X"=222.43848, "Y"=128.20334}, {"X"=242.81136, "Y"=141.80414}, {"X"=266.64935, "Y"=176.93747}, {"X"=280.11868, "Y"=194.3845}, {"X"=290.03348, "Y"=186.11928}, {"X"=311.69507, "Y"=203.72618}, {"X"=323.29514, "Y"=199.7866}, {"X"=340.00082, "Y"=148.7848}, {"X"=368.4223, "Y"=149.55873}, {"X"=398.6007, "Y"=141.72342}, {"X"=420.54715, "Y"=129.29317}, {"X"=432.351, "Y"=125.26218}, {"X"=442.31808, "Y"=129.89221}, {"X"=435.7848, "Y"=120.99476}, {"X"=428.84518, "Y"=133.87096}, {"X"=410.11725, "Y"=155.01231}, {"X"=393.2317, "Y"=171.7661}, {"X"=378.1757, "Y"=179.93015}, {"X"=373.08405, "Y"=192.60152}, {"X"=376.28946, "Y"=205.43776}, {"X"=382.65707, "Y"=230.9374}, {"X"=369.22177, "Y"=264.02118}, {"X"=374.17148, "Y"=259.99072}, {"X"=375.66516, "Y"=276.62363}, {"X"=395.47556, "Y"=260.53992}, {"X"=408.64023, "Y"=256.71732}, {"X"=412.17014, "Y"=240.10042}, {"X"=418.88022, "Y"=231.88513}, {"X"=426.49588, "Y"=172.66246}, {"X"=446.61935, "Y"=164.61723}, {"X"=453.94016, "Y"=134.56003}, {"X"=457.4812, "Y"=125.9551}, {"X"=461.7439, "Y"=86.59075}, {"X"=472.51974, "Y"=60.277336}, {"X"=478.17383, "Y"=38.074444}, {"X"=488.98636, "Y"=15.85421}, {"X"=409.66702, "Y"=298.09103}, {"X"=404.38705, "Y"=326.54724}, {"X"=392.95547, "Y"=334.37915}, {"X"=391.05637, "Y"=358.54294}, {"X"=386.22525, "Y"=358.42465}, {"X"=378.28488, "Y"=346.14886}, {"X"=374.98547, "Y"=354.12793}, {"X"=357.20303, "Y"=361.73068}, {"X"=345.95633, "Y"=353.41556}, {"X"=345.9275, "Y"=361.45517}, {"X"=337.87146, "Y"=361.25833}, {"X"=329.81088, "Y"=365.07376}, {"X"=324.97827, "Y"=360.9433}, {"X"=328.19186, "Y"=385.01053}, {"X"=326.5875, "Y"=380.9879}, {"X"=320.1707, "Y"=388.79562}, {"X"=329.75198, "Y"=448.02277}, {"X"=323.4099, "Y"=459.52567}, {"X"=323.4099, "Y"=459.52567}, {"X"=320.2544, "Y"=471.0546}, {"X"=315.49844, "Y"=463.21564}, {"X"=312.32318, "Y"=459.26917}, {"X"=203.00899, "Y"=317.45316}, {"X"=206.35289, "Y"=321.6138}, {"X"=202.74171, "Y"=305.17905}, {"X"=203.36356, "Y"=333.736}, {"X"=202.00755, "Y"=345.8467}, {"X"=203.80391, "Y"=353.95782}, {"X"=205.42209, "Y"=353.99744}, {"X"=208.40495, "Y"=341.9621}, {"X"=213.10675, "Y"=333.97717}, {"X"=216.74751, "Y"=354.27475}, {"X"=208.40495, "Y"=341.9621}, {"X"=213.18805, "Y"=338.0325}, {"X"=222.32468, "Y"=305.67108}, {"X"=237.0053, "Y"=306.03998}, {"X"=235.57072, "Y"=318.26608}, {"X"=244.86523, "Y"=285.6842}, {"X"=256.06488, "Y"=265.26852}, {"X"=249.38492, "Y"=256.77393}, {"X"=254.37074, "Y"=261.06677}, {"X"=244.86523, "Y"=285.6842}, {"X"=246.38605, "Y"=277.4598}, {"X"=271.2776, "Y"=310.9925}, {"X"=303.92316, "Y"=336.22504}, {"X"=329.8166, "Y"=357.0434}, {"X"=344.28995, "Y"=369.43262}, {"X"=349.09937, "Y"=373.54947}, {"X"=358.83722, "Y"=357.75403}, {"X"=378.28488, "Y"=346.14886}, {"X"=386.39902, "Y"=342.31058}, {"X"=384.5726, "Y"=362.3994}, {"X"=381.63367, "Y"=334.09833}, {"X"=372.05978, "Y"=317.59946}, {"X"=368.84528, "Y"=313.4388}, {"X"=375.34088, "Y"=313.60168}, {"X"=372.1938, "Y"=301.24713}, {"X"=378.62643, "Y"=309.59845}, {"X"=375.5205, "Y"=293.11795}, {"X"=375.62894, "Y"=280.75623}, {"X"=392.53955, "Y"=231.19595}, {"X"=409.49548, "Y"=197.8271}, {"X"=429.8978, "Y"=168.46263}, {"X"=443.64062, "Y"=147.2842}, {"X"=465.95886, "Y"=121.82849}, {"X"=484.8619, "Y"=104.84823}, {"X"=495.70325, "Y"=78.70221}, {"X"=515.1099, "Y"=52.567978}, {"X"=516.80365, "Y"=52.616356}, {"X"=516.22815, "Y"=70.41432}, {"X"=515.79877, "Y"=83.69256}, {"X"=519.3137, "Y"=79.36826}, {"X"=510.32788, "Y"=96.769936}, {"X"=494.93976, "Y"=105.12901}, {"X"=480.57452, "Y"=139.63138}, {"X"=189.6808, "Y"=304.85086}, {"X"=194.8642, "Y"=317.24982}, {"X"=194.8642, "Y"=317.24982}, {"X"=194.0933, "Y"=353.72003}, {"X"=189.62894, "Y"=369.67828}, {"X"=186.40042, "Y"=369.59988}, {"X"=187.9158, "Y"=365.62833}, {"X"=189.53119, "Y"=365.66763}, {"X"=197.69905, "Y"=369.87418}, {"X"=197.79086, "Y"=373.8785}, {"X"=206.02516, "Y"=382.06412}, {"X"=220.21054, "Y"=366.414}, {"X"=231.0312, "Y"=338.4732}, {"X"=247.13155, "Y"=330.76196}, {"X"=276.3768, "Y"=335.5432}, {"X"=276.3054, "Y"=327.42398}, {"X"=297.34076, "Y"=315.73004}, {"X"=316.84683, "Y"=316.21808}, {"X"=321.7218, "Y"=316.34006}, {"X"=329.84534, "Y"=316.5433}, {"X"=336.31265, "Y"=332.97412}, {"X"=370.21255, "Y"=345.94992}, {"X"=382.96317, "Y"=362.36008}, {"X"=381.35367, "Y"=362.32077}, {"X"=392.5709, "Y"=366.60388}, {"X"=387.52594, "Y"=386.44153}, {"X"=393.98352, "Y"=382.6169}, {"X"=400.34277, "Y"=386.75064}, {"X"=394.03223, "Y"=378.63202}, {"X"=398.7409, "Y"=386.712}, {"X"=392.6187, "Y"=362.596}, {"X"=395.7365, "Y"=370.6842}, {"X"=395.8869, "Y"=358.66122}, {"X"=399.00195, "Y"=366.76068}, {"X"=408.8248, "Y"=354.9583}, {"X"=397.85852, "Y"=330.44562}, {"X"=388.51004, "Y"=297.556}, {"X"=385.60077, "Y"=264.4425}, {"X"=377.90588, "Y"=209.71823}, {"X"=348.22894, "Y"=183.40361}, {"X"=316.60648, "Y"=165.4034}, {"X"=299.7625, "Y"=130.32654}, {"X"=267.53833, "Y"=98.79328}, {"X"=247.08128, "Y"=84.985886}, {"X"=231.54597, "Y"=66.80355}, {"X"=217.61603, "Y"=48.552227}, {"X"=206.92899, "Y"=25.769863}, {"X"=204.75536, "Y"=3.0574033}, {"X"=161.49467, "Y"=-7.314883}, {"X"=129.4768, "Y"=14.49116}, {"X"=119.63426, "Y"=27.770283}, {"X"=137.07181, "Y"=37.277576}, {"X"=148.91959, "Y"=33.117714}, {"X"=166.2862, "Y"=42.604843}, {"X"=199.99265, "Y"=101.313324}, {"X"=209.78993, "Y"=83.94041}, {"X"=244.24585, "Y"=124.442085}, {"X"=283.1259, "Y"=151.56154}, {"X"=301.6406, "Y"=177.87642}, {"X"=321.62427, "Y"=182.69121}, {"X"=344.86215, "Y"=196.10727}, {"X"=366.23987, "Y"=222.08723}, {"X"=399.74298, "Y"=310.12906}, {"X"=399.6362, "Y"=318.2894}, {"X"=394.42438, "Y"=346.54663}, {"X"=381.43338, "Y"=354.28616}, {"X"=381.23453, "Y"=374.32956}, {"X"=376.4522, "Y"=370.21506}, {"X"=373.27115, "Y"=366.13333}, {"X"=357.1357, "Y"=373.74457}, {"X"=342.69318, "Y"=365.38782}, {"X"=334.6171, "Y"=381.182}, {"X"=316.92422, "Y"=364.75955}, {"X"=302.52182, "Y"=388.3709}, {"X"=304.0644, "Y"=372.45624}, {"X"=281.59027, "Y"=379.90033}, {"X"=257.85187, "Y"=411.06793}, {"X"=253.20705, "Y"=422.7685}, {"X"=239.14238, "Y"=442.0137}, {"X"=208.62488, "Y"=503.05353}, {"X"=198.1343, "Y"=525.6228}, {"X"=178.45244, "Y"=551.55914}, {"X"=176.05566, "Y"=577.6269}, {"X"=160.96132, "Y"=592.1177}, {"X"=150.58563, "Y"=606.6329}, {"X"=143.3505, "Y"=621.13727}, {"X"=276.12592, "Y"=307.02295}, {"X"=275.9814, "Y"=290.59537}, {"X"=279.38416, "Y"=307.10483}, {"X"=282.51654, "Y"=290.761}, {"X"=280.88287, "Y"=290.71957}, {"X"=289.13058, "Y"=303.25336}, {"X"=302.13248, "Y"=295.3716}, {"X"=298.88867, "Y"=299.3973}, {"X"=305.4104, "Y"=299.5619}, {"X"=302.14966, "Y"=299.4796}, {"X"=315.29037, "Y"=352.66306}, {"X"=342.68112, "Y"=369.39346}, {"X"=374.56567, "Y"=401.99783}, {"X"=393.5483, "Y"=418.22644}, {"X"=399.76248, "Y"=430.1451}, {"X"=413.81497, "Y"=446.09067}, {"X"=415.71643, "Y"=426.60336}, {"X"=423.7341, "Y"=422.87}, {"X"=411.4928, "Y"=390.99335}, {"X"=405.2613, "Y"=378.90402}, {"X"=403.88043, "Y"=362.87115}, {"X"=384.78387, "Y"=342.27066}, {"X"=376.74374, "Y"=338.02747}, {"X"=362.2958, "Y"=321.42987}, {"X"=359.05173, "Y"=321.34888}, {"X"=357.54407, "Y"=300.87744}, {"X"=352.67902, "Y"=296.64987}, {"X"=352.73758, "Y"=284.3011}, {"X"=346.1754, "Y"=292.37427}, {"X"=349.48862, "Y"=280.0895}, {"X"=354.45377, "Y"=267.79407}, {"X"=351.21524, "Y"=259.39896}, {"X"=365.94513, "Y"=263.9369}, {"X"=385.47028, "Y"=276.87424}, {"X"=387.1935, "Y"=268.63446}, {"X"=385.64438, "Y"=260.28647}, {"X"=380.64783, "Y"=268.46643}, {"X"=362.66818, "Y"=263.85257}, {"X"=356.20212, "Y"=247.01471}, {"X"=361.13263, "Y"=247.14262}, {"X"=357.82227, "Y"=251.23369}, {"X"=369.19012, "Y"=268.17233}, {"X"=369.4125, "Y"=238.98643}, {"X"=367.79776, "Y"=234.74957}, {"X"=377.90588, "Y"=209.71823}, {"X"=401.2153, "Y"=197.60678}, {"X"=431.63977, "Y"=164.21188}, {"X"=450.13174, "Y"=156.09962}, {"X"=460.32855, "Y"=147.73956}, {"X"=459.0565, "Y"=130.35278}, {"X"=452.36203, "Y"=130.16858}, {"X"=447.522, "Y"=121.31907}, {"X"=422.07858, "Y"=138.02852}, {"X"=391.7142, "Y"=158.82507}, {"X"=374.9604, "Y"=166.97914}, {"X"=368.17026, "Y"=183.93759}, {"X"=356.5391, "Y"=183.62614}, {"X"=348.17935, "Y"=196.19554}, {"X"=333.21695, "Y"=221.21957}, {"X"=320.02115, "Y"=241.89091}, {"X"=313.4532, "Y"=250.08505}, {"X"=308.482, "Y"=237.399}, {"X"=301.8715, "Y"=233.02834}, {"X"=275.13385, "Y"=194.25186}, {"X"=245.0917, "Y"=184.91838}, {"X"=211.08717, "Y"=149.604}, {"X"=197.47821, "Y"=140.56712}, {"X"=185.29665, "Y"=122.82005}, {"X"=183.61104, "Y"=122.773674}, {"X"=181.7095, "Y"=113.974495}, {"X"=176.19547, "Y"=96.248344}, {"X"=183.3977, "Y"=114.02114}, {"X"=185.19133, "Y"=118.4472}, {"X"=193.52542, "Y"=114.30097}, {"X"=209.5835, "Y"=158.2031}, {"X"=216.60594, "Y"=175.59462}, {"X"=226.76686, "Y"=184.42871}, {"X"=247.04887, "Y"=206.25818}, {"X"=265.47458, "Y"=223.65866}, {"X"=270.6784, "Y"=248.97769}, {"X"=272.28528, "Y"=244.83765}, {"X"=270.5975, "Y"=240.60599}, {"X"=268.90723, "Y"=236.36795}, {"X"=248.53703, "Y"=193.54414}, {"X"=219.70802, "Y"=162.78683}, {"X"=205.69797, "Y"=132.09941}, {"X"=190.45438, "Y"=127.3251}, {"X"=185.08585, "Y"=114.06778}, {"X"=176.42027, "Y"=105.05465}, {"X"=177.77762, "Y"=91.88256}, {"X"=176.08281, "Y"=91.83524}, {"X"=193.32669, "Y"=105.523735}, {"X"=193.8224, "Y"=127.41758}, {"X"=200.9313, "Y"=144.99792}, {"X"=204.64992, "Y"=162.38022}, {"X"=223.43413, "Y"=184.33966}, {"X"=232.25061, "Y"=214.33968}, {"X"=237.80643, "Y"=252.30412}, {"X"=244.68811, "Y"=273.27588}, {"X"=246.4439, "Y"=281.5958}, {"X"=252.99362, "Y"=281.7625}, {"X"=255.91173, "Y"=252.77185}, {"X"=273.7033, "Y"=219.65587}, {"X"=283.62872, "Y"=219.91666}, {"X"=291.74744, "Y"=194.69392}, {"X"=316.59274, "Y"=156.78804}, {"X"=355.0284, "Y"=153.51537}, {"X"=386.89218, "Y"=141.40326}, {"X"=393.83652, "Y"=119.8357}, {"X"=400.7755, "Y"=102.50546}, {"X"=402.45908, "Y"=102.55237}, {"X"=400.60727, "Y"=115.65212}, {"X"=383.50323, "Y"=145.64322}, {"X"=363.4643, "Y"=140.76265}, {"X"=360.0398, "Y"=153.65154}, {"X"=359.88785, "Y"=179.43942}, {"X"=354.7276, "Y"=213.33804}, {"X"=347.99936, "Y"=242.6183}, {"X"=334.81598, "Y"=254.8102}, {"X"=310.21027, "Y"=266.6584}, {"X"=267.6417, "Y"=273.86258}, {"X"=235.43993, "Y"=310.09396}, {"X"=212.8622, "Y"=321.77597}, {"X"=211.56552, "Y"=337.99243}, {"X"=200.11526, "Y"=333.6556}, {"X"=206.35289, "Y"=321.6138}, {"X"=203.18652, "Y"=325.60635}, {"X"=206.35289, "Y"=321.6138}, {"X"=210.98581, "Y"=309.4808}, {"X"=213.43265, "Y"=268.3286}, {"X"=216.79727, "Y"=272.563}, {"X"=226.64343, "Y"=272.81467}, {"X"=251.51862, "Y"=294.09167}, {"X"=251.24768, "Y"=273.44354}, {"X"=258.15155, "Y"=302.4733}, {"X"=256.47006, "Y"=298.3269}, {"X"=232.18028, "Y"=310.0122}, {"X"=212.61656, "Y"=309.5217}, {"X"=198.12233, "Y"=317.33118}, {"X"=184.98619, "Y"=312.91904}, {"X"=195.92911, "Y"=292.68588}, {"X"=193.13898, "Y"=313.12302}, {"X"=194.67432, "Y"=309.07184}, {"X"=184.98619, "Y"=312.91904}, {"X"=201.47018, "Y"=321.49216}, {"X"=214.56981, "Y"=325.8893}, {"X"=219.98273, "Y"=354.35397}, {"X"=226.38083, "Y"=350.48126}, {"X"=231.57484, "Y"=370.69653}, {"X"=233.51807, "Y"=390.6877}, {"X"=225.91255, "Y"=414.25327}, {"X"=197.19217, "Y"=417.5124}, {"X"=177.33533, "Y"=452.2606}, {"X"=173.83134, "Y"=440.48932}, {"X"=162.46326, "Y"=486.69604}, {"X"=169.11844, "Y"=498.34247}, {"X"=170.5874, "Y"=494.54938}, {"X"=167.98312, "Y"=513.5691}, {"X"=149.46707, "Y"=524.54095}, {"X"=135.32622, "Y"=524.2266}, {"X"=130.74756, "Y"=527.9106}, {"X"=-459.3773, "Y"=-967.1659}] {"Y" format="%.2f"; "X" format="%.2f"}
  in  "auto bottom huyun vs chen jin":T1[](array[typedef])=[{"X"=378.4836, "Y"=1076.3296}, {"X"=378.31952, "Y"=1091.547}, {"X"=377.0474, "Y"=1079.3596}, {"X"=377.532, "Y"=1033.1877}, {"X"=379.11667, "Y"=1017.6248}, {"X"=382.38806, "Y"=979.86176}, {"X"=387.9911, "Y"=872.9198}, {"X"=384.9125, "Y"=1008.317}, {"X"=377.49942, "Y"=1036.2931}, {"X"=367.56186, "Y"=1039.2407}, {"X"=358.88235, "Y"=1066.8547}, {"X"=356.16223, "Y"=1051.4358}, {"X"=354.8963, "Y"=1026.6094}, {"X"=348.956, "Y"=1081.9874}, {"X"=341.90778, "Y"=1091.007}, {"X"=336.3094, "Y"=1087.8859}, {"X"=333.49533, "Y"=1093.9166}, {"X"=325.09058, "Y"=1090.7576}, {"X"=323.6834, "Y"=1078.5596}, {"X"=326.4935, "Y"=1081.6516}, {"X"=333.47153, "Y"=1109.0316}, {"X"=351.36417, "Y"=1157.0256}, {"X"=370.4849, "Y"=1180.8024}, {"X"=379.64313, "Y"=1221.5149}, {"X"=398.44678, "Y"=1238.9417}, {"X"=403.59134, "Y"=1256.0625}, {"X"=400.84616, "Y"=1172.4313}, {"X"=411.4425, "Y"=1270.2786}, {"X"=403.59134, "Y"=1256.0625}, {"X"=388.91043, "Y"=1241.6702}, {"X"=384.94864, "Y"=1233.0537}, {"X"=378.60092, "Y"=1192.5806}, {"X"=368.95218, "Y"=1198.2634}, {"X"=359.46793, "Y"=1183.5748}, {"X"=355.32794, "Y"=1186.438}, {"X"=353.98914, "Y"=1180.577}, {"X"=345.96033, "Y"=1127.2258}, {"X"=346.07306, "Y"=1100.159}, {"X"=344.7571, "Y"=1078.8755}, {"X"=343.40747, "Y"=1063.552}, {"X"=349.04297, "Y"=1063.6376}, {"X"=354.67764, "Y"=1063.7231}, {"X"=362.84958, "Y"=1100.4059}, {"X"=376.10492, "Y"=1169.1539}, {"X"=391.01474, "Y"=1186.9226}, {"X"=395.94513, "Y"=1224.601}, {"X"=411.64856, "Y"=1258.9946}, {"X"=414.24313, "Y"=1264.6772}, {"X"=412.78976, "Y"=1270.2954}, {"X"=410.0952, "Y"=1270.2618}, {"X"=392.65604, "Y"=1264.4062}, {"X"=384.66382, "Y"=1255.8226}, {"X"=375.46558, "Y"=1230.0684}, {"X"=364.74893, "Y"=1209.7914}, {"X"=358.0546, "Y"=1189.3909}, {"X"=349.79077, "Y"=1195.1007}, {"X"=345.71423, "Y"=1186.3075}, {"X"=338.94196, "Y"=1150.936}, {"X"=337.60873, "Y"=1130.0952}, {"X"=333.4479, "Y"=1124.053}, {"X"=333.43848, "Y"=1130.0355}, {"X"=345.98526, "Y"=1121.237}, {"X"=360.0327, "Y"=1103.3865}, {"X"=378.58255, "Y"=1067.1533}, {"X"=388.66498, "Y"=1048.8491}, {"X"=393.11145, "Y"=1033.4308}, {"X"=394.96344, "Y"=1002.1918}, {"X"=394.74475, "Y"=1017.8718}, {"X"=387.25323, "Y"=1048.8274}, {"X"=382.8384, "Y"=1064.151}, {"X"=383.27048, "Y"=1027.0543}, {"X"=372.86658, "Y"=1076.2451}, {"X"=365.81912, "Y"=1079.1913}, {"X"=360.18225, "Y"=1082.1553}, {"X"=354.60547, "Y"=1075.9706}, {"X"=344.81644, "Y"=1063.5734}, {"X"=333.50967, "Y"=1084.8022}, {"X"=315.3491, "Y"=1123.7925}, {"X"=284.82785, "Y"=1138.2916}, {"X"=260.1361, "Y"=1161.6593}, {"X"=236.88428, "Y"=1176.0468}, {"X"=217.89015, "Y"=1190.4108}, {"X"=183.72298, "Y"=1198.685}, {"X"=163.08911, "Y"=1198.4088}, {"X"=146.73007, "Y"=1238.5565}, {"X"=140.35464, "Y"=1249.8835}, {"X"=135.3676, "Y"=1261.175}, {"X"=128.55386, "Y"=1195.036}, {"X"=129.81401, "Y"=1258.2716}, {"X"=138.76656, "Y"=1244.1656}, {"X"=151.237, "Y"=1212.7449}, {"X"=174.92511, "Y"=1224.5863}, {"X"=189.39015, "Y"=1204.5664}, {"X"=196.09793, "Y"=1198.8507}, {"X"=209.41655, "Y"=1181.5316}, {"X"=222.76524, "Y"=1161.1404}, {"X"=233.38675, "Y"=1137.5612}, {"X"=238.89754, "Y"=1134.6573}, {"X"=238.62772, "Y"=1119.6874}, {"X"=238.24713, "Y"=1098.5728}, {"X"=225.34917, "Y"=1152.3052}, {"X"=207.96494, "Y"=1178.5831}, {"X"=189.05634, "Y"=1192.9366}, {"X"=175.7459, "Y"=1207.2828}, {"X"=154.60732, "Y"=1230.0663}, {"X"=137.97043, "Y"=1224.1042}, {"X"=129.93227, "Y"=1261.1068}, {"X"=134.5857, "Y"=1275.2823}, {"X"=134.35536, "Y"=1269.6428}, {"X"=131.64262, "Y"=1269.6091}, {"X"=133.69322, "Y"=1286.5044}, {"X"=140.57867, "Y"=1255.5703}, {"X"=159.11325, "Y"=1241.5724}, {"X"=180.13123, "Y"=1216.0134}, {"X"=188.10083, "Y"=1207.4468}, {"X"=198.53635, "Y"=1187.2311}, {"X"=216.17819, "Y"=1175.7632}, {"X"=232.28477, "Y"=1152.4023}, {"X"=245.7573, "Y"=1128.7803}, {"X"=255.55318, "Y"=1131.9093}, {"X"=283.2013, "Y"=1111.3119}, {"X"=323.678, "Y"=1066.3213}, {"X"=351.97516, "Y"=1042.0979}, {"X"=371.98166, "Y"=1020.63776}, {"X"=396.29892, "Y"=1008.4984}, {"X"=403.90857, "Y"=977.03613}, {"X"=408.0467, "Y"=986.6206}, {"X"=405.1381, "Y"=989.73773}, {"X"=400.85327, "Y"=989.6684}, {"X"=391.90375, "Y"=1017.8269}, {"X"=378.9151, "Y"=1036.3151}, {"X"=371.77823, "Y"=1042.4044}, {"X"=366.24854, "Y"=1026.7875}, {"X"=354.60547, "Y"=1075.9706}, {"X"=350.26788, "Y"=1100.2208}, {"X"=350.20718, "Y"=1112.287}, {"X"=354.3734, "Y"=1115.3549}, {"X"=364.24728, "Y"=1100.4265}, {"X"=372.3143, "Y"=1133.5763}, {"X"=396.9365, "Y"=1157.662}, {"X"=421.01068, "Y"=1196.0596}, {"X"=432.86688, "Y"=1216.4614}, {"X"=451.095, "Y"=1248.1578}, {"X"=460.2619, "Y"=1211.0591}, {"X"=455.77863, "Y"=1225.3838}, {"X"=451.3978, "Y"=1236.7717}, {"X"=436.14935, "Y"=1250.8063}, {"X"=414.7239, "Y"=1239.1515}, {"X"=405.42215, "Y"=1227.5931}, {"X"=397.3928, "Y"=1218.8723}, {"X"=382.852, "Y"=1180.9712}, {"X"=373.2625, "Y"=1177.9143}, {"X"=366.561, "Y"=1157.2378}, {"X"=362.37207, "Y"=1163.0791}, {"X"=358.31253, "Y"=1151.208}, {"X"=352.9797, "Y"=1115.3346}, {"X"=346.12357, "Y"=1088.0319}, {"X"=344.7571, "Y"=1078.8755}, {"X"=315.2771, "Y"=1090.6119}, {"X"=291.4553, "Y"=1093.2948}, {"X"=292.87793, "Y"=1096.348}, {"X"=291.26117, "Y"=1065.8301}, {"X"=291.51953, "Y"=1102.3812}, {"X"=284.6752, "Y"=1120.352}, {"X"=284.7771, "Y"=1132.3265}, {"X"=281.99484, "Y"=1132.2869}, {"X"=282.02194, "Y"=1135.2714}, {"X"=291.49814, "Y"=1099.3562}, {"X"=293.84027, "Y"=1028.769}, {"X"=290.50763, "Y"=959.21533}, {"X"=290.755, "Y"=994.21326}, {"X"=307.90787, "Y"=991.32904}, {"X"=316.4447, "Y"=966.0417}, {"X"=304.85883, "Y"=946.60767}, {"X"=316.35977, "Y"=920.91437}, {"X"=313.36108, "Y"=881.52795}, {"X"=297.1594, "Y"=861.33997}, {"X"=292.7529, "Y"=861.26135}, {"X"=296.98972, "Y"=831.1879}, {"X"=296.8755, "Y"=810.88763}, {"X"=310.98715, "Y"=1063.0593}, {"X"=312.16562, "Y"=978.7169}, {"X"=312.12186, "Y"=962.77386}, {"X"=315.07562, "Y"=997.7607}, {"X"=310.89334, "Y"=1032.1482}, {"X"=308.0887, "Y"=1041.4186}, {"X"=308.23297, "Y"=1081.3785}, {"X"=299.89938, "Y"=1099.4797}, {"X"=297.1706, "Y"=1111.5151}, {"X"=297.11707, "Y"=1102.4634}, {"X"=290.23087, "Y"=1117.4299}, {"X"=268.1875, "Y"=1141.0326}, {"X"=264.17236, "Y"=1152.8489}, {"X"=253.21834, "Y"=1161.5632}, {"X"=218.87401, "Y"=1172.8645}, {"X"=191.01025, "Y"=1213.2697}, {"X"=171.1029, "Y"=1233.1469}, {"X"=161.14227, "Y"=1221.529}, {"X"=159.77289, "Y"=1221.5111}, {"X"=168.84761, "Y"=1247.3997}, {"X"=188.15555, "Y"=1256.1714}, {"X"=209.53432, "Y"=1242.2188}, {"X"=223.08801, "Y"=1239.5382}, {"X"=240.48207, "Y"=1222.567}, {"X"=260.81613, "Y"=1211.3032}, {"X"=274.50464, "Y"=1211.4844}, {"X"=281.07455, "Y"=1182.5074}, {"X"=290.341, "Y"=1132.406}, {"X"=301.48148, "Y"=1135.5483}, {"X"=312.63754, "Y"=1150.5667}, {"X"=336.10437, "Y"=1183.2567}, {"X"=375.73758, "Y"=1204.153}, {"X"=401.2057, "Y"=1236.1227}, {"X"=421.10107, "Y"=1259.1141}, {"X"=434.5352, "Y"=1262.1096}, {"X"=438.11035, "Y"=1225.1526}, {"X"=439.72504, "Y"=1270.6317}, {"X"=428.70627, "Y"=1281.724}, {"X"=420.64474, "Y"=1281.6245}, {"X"=408.8475, "Y"=1264.6095}, {"X"=399.66962, "Y"=1247.5005}, {"X"=385.12805, "Y"=1218.7109}, {"X"=373.00256, "Y"=1204.1165}, {"X"=366.18875, "Y"=1201.1277}, {"X"=358.11374, "Y"=1180.6334}, {"X"=347.2845, "Y"=1142.1526}, {"X"=343.22214, "Y"=1115.193}, {"X"=329.29343, "Y"=1093.8545}, {"X"=306.86353, "Y"=1090.4872}, {"X"=282.6918, "Y"=1053.3939}, {"X"=238.78107, "Y"=1049.6334}, {"X"=217.86893, "Y"=1064.718}, {"X"=203.43129, "Y"=1052.18}, {"X"=177.064, "Y"=1070.2383}, {"X"=315.07562, "Y"=997.7607}, {"X"=316.52222, "Y"=1007.22766}, {"X"=310.1399, "Y"=783.82227}, {"X"=316.55756, "Y"=1026.0082}, {"X"=312.20044, "Y"=991.3983}, {"X"=311.02432, "Y"=1075.3156}, {"X"=304.07217, "Y"=1093.4813}, {"X"=299.86703, "Y"=1093.4192}, {"X"=297.06332, "Y"=1093.3777}, {"X"=294.23972, "Y"=1090.2999}, {"X"=301.28412, "Y"=1096.472}, {"X"=309.75858, "Y"=1117.7126}, {"X"=326.48465, "Y"=1147.7971}, {"X"=347.06183, "Y"=1192.1548}, {"X"=367.27954, "Y"=1232.8246}, {"X"=388.5317, "Y"=1269.9926}, {"X"=400.9332, "Y"=1253.1948}, {"X"=402.1019, "Y"=1264.5248}, {"X"=393.67932, "Y"=1286.8892}, {"X"=384.2068, "Y"=1292.3577}, {"X"=378.9344, "Y"=1283.9109}, {"X"=366.78378, "Y"=1289.354}, {"X"=358.88174, "Y"=1266.804}, {"X"=347.023, "Y"=1200.8711}, {"X"=338.90173, "Y"=1165.6985}, {"X"=343.16837, "Y"=1130.1748}, {"X"=359.7794, "Y"=1139.3558}, {"X"=382.4833, "Y"=1094.6412}, {"X"=401.65442, "Y"=1030.4553}, {"X"=419.35788, "Y"=993.12744}, {"X"=430.77017, "Y"=993.3116}, {"X"=443.07318, "Y"=955.3383}, {"X"=459.0597, "Y"=893.9619}, {"X"=479.8087, "Y"=881.15594}, {"X"=484.4885, "Y"=871.3179}, {"X"=456.32086, "Y"=887.3366}, {"X"=443.21506, "Y"=887.10675}, {"X"=429.3197, "Y"=853.7054}, {"X"=416.11874, "Y"=853.4681}, {"X"=403.7693, "Y"=892.997}, {"X"=382.971, "Y"=928.5418}, {"X"=358.20505, "Y"=953.92615}, {"X"=343.76733, "Y"=963.29645}, {"X"=316.51038, "Y"=1000.9356}, {"X"=296.6814, "Y"=1028.8135}, {"X"=286.88425, "Y"=1047.2821}, {"X"=279.806, "Y"=1047.1731}, {"X"=271.4132, "Y"=1056.3041}, {"X"=267.39316, "Y"=1074.6597}, {"X"=268.97946, "Y"=1089.9253}, {"X"=268.97946, "Y"=1089.9253}, {"X"=275.99786, "Y"=1090.0294}, {"X"=287.1764, "Y"=1084.1113}, {"X"=295.60483, "Y"=1084.237}, {"X"=320.8727, "Y"=1078.5175}, {"X"=340.48834, "Y"=1097.0504}, {"X"=350.2375, "Y"=1106.2614}, {"X"=354.51578, "Y"=1091.194}, {"X"=358.55432, "Y"=1115.4155}, {"X"=364.1757, "Y"=1109.4797}, {"X"=371.17862, "Y"=1106.5679}, {"X"=326.4915, "Y"=1096.8439}, {"X"=286.672, "Y"=834.3677}, {"X"=288.51126, "Y"=1074.977}, {"X"=288.65097, "Y"=1093.2533}, {"X"=287.03085, "Y"=1065.766}, {"X"=287.24875, "Y"=1093.2325}, {"X"=290.07547, "Y"=1096.3066}, {"X"=285.5448, "Y"=1056.5199}, {"X"=282.4736, "Y"=1028.5913}, {"X"=277.93768, "Y"=1000.318}, {"X"=264.8387, "Y"=981.1236}, {"X"=248.40437, "Y"=939.2113}, {"X"=231.8687, "Y"=906.41473}, {"X"=214.07964, "Y"=892.97943}, {"X"=186.84355, "Y"=859.3715}, {"X"=177.53662, "Y"=791.6139}, {"X"=242.23543, "Y"=916.3918}, {"X"=234.90233, "Y"=913.00415}, {"X"=246.59932, "Y"=916.46643}, {"X"=256.7351, "Y"=913.37854}, {"X"=241.19531, "Y"=853.66736}, {"X"=233.04042, "Y"=809.70624}, {"X"=196.93904, "Y"=791.97736}, {"X"=198.3466, "Y"=788.57806}, {"X"=198.3466, "Y"=788.57806}, {"X"=389.95572, "Y"=1058.1147}, {"X"=391.03735, "Y"=1082.6166}, {"X"=390.0767, "Y"=1048.8708}, {"X"=387.52475, "Y"=1027.1211}, {"X"=389.26324, "Y"=1002.1005}, {"X"=394.5708, "Y"=1030.3446}, {"X"=396.1207, "Y"=1021.01825}, {"X"=393.1539, "Y"=1030.3224}, {"X"=387.33057, "Y"=1042.6451}, {"X"=382.87418, "Y"=1061.0809}, {"X"=375.8629, "Y"=1057.8994}, {"X"=370.11313, "Y"=1070.0884}, {"X"=365.84412, "Y"=1076.1395}, {"X"=358.79974, "Y"=1079.086}, {"X"=350.45172, "Y"=1063.6589}, {"X"=347.6342, "Y"=1063.6162}, {"X"=347.51184, "Y"=1091.0901}, {"X"=348.6707, "Y"=1142.1722}, {"X"=349.86407, "Y"=1180.5208}, {"X"=359.22287, "Y"=1218.37}, {"X"=369.86514, "Y"=1247.1195}, {"X"=377.74536, "Y"=1269.8579}, {"X"=381.7906, "Y"=1269.9084}, {"X"=387.25735, "Y"=1264.3384}, {"X"=400.208, "Y"=1213.148}, {"X"=418.568, "Y"=1250.5822}, {"X"=438.70905, "Y"=1312.4495}, {"X"=437.1761, "Y"=1320.708}, {"X"=438.57495, "Y"=1317.9689}, {"X"=438.2411, "Y"=1331.7102}, {"X"=432.29025, "Y"=1301.2904}, {"X"=418.51212, "Y"=1253.4182}, {"X"=408.09174, "Y"=1230.4927}, {"X"=403.0299, "Y"=1207.4102}, {"X"=406.29956, "Y"=1175.4384}, {"X"=414.20084, "Y"=1119.2244}, {"X"=416.0948, "Y"=1092.1073}, {"X"=422.5922, "Y"=1046.2831}, {"X"=418.9495, "Y"=1089.1149}, {"X"=406.20465, "Y"=1098.0198}, {"X"=399.5862, "Y"=1073.5922}, {"X"=396.55637, "Y"=1088.7819}, {"X"=394.6142, "Y"=1027.2323}, {"X"=386.10672, "Y"=1027.0989}, {"X"=378.7816, "Y"=1048.6969}, {"X"=371.17862, "Y"=1106.5679}, {"X"=366.94022, "Y"=1112.5305}, {"X"=360.054, "Y"=1100.3647}, {"X"=355.84158, "Y"=1103.325}, {"X"=353.06418, "Y"=1100.262}, {"X"=357.3563, "Y"=1085.1578}, {"X"=357.41544, "Y"=1076.0128}, {"X"=363.93903, "Y"=1139.4149}, {"X"=377.8012, "Y"=1139.6117}, {"X"=380.20392, "Y"=1172.1471}, {"X"=373.2625, "Y"=1177.9143}, {"X"=376.5186, "Y"=1258.5509}, {"X"=382.96738, "Y"=1283.9604}, {"X"=380.44223, "Y"=1269.8916}, {"X"=378.9344, "Y"=1283.9109}, {"X"=358.763, "Y"=1283.6627}, {"X"=333.19278, "Y"=1286.1475}, {"X"=322.42133, "Y"=1274.7968}, {"X"=314.25797, "Y"=1246.4088}, {"X"=301.89597, "Y"=1217.6157}, {"X"=296.19754, "Y"=1179.788}, {"X"=292.02478, "Y"=1173.8691}, {"X"=286.46057, "Y"=1167.916}, {"X"=283.386, "Y"=1132.3066}, {"X"=279.06766, "Y"=1117.2684}, {"X"=272.0556, "Y"=1114.1602}, {"X"=261.24133, "Y"=1140.9342}, {"X"=236.44554, "Y"=1152.4606}, {"X"=211.61502, "Y"=1158.0316}, {"X"=194.81741, "Y"=1151.8776}, {"X"=174.45331, "Y"=1166.3693}, {"X"=160.33708, "Y"=1198.372}, {"X"=158.30157, "Y"=1218.6107}, {"X"=159.77289, "Y"=1221.5111}, {"X"=153.56902, "Y"=1163.132}, {"X"=154.39915, "Y"=1224.3185}, {"X"=161.24237, "Y"=1224.4078}, {"X"=168.6886, "Y"=1201.3892}, {"X"=190.9281, "Y"=1210.3783}, {"X"=205.49962, "Y"=1190.2434}, {"X"=213.62312, "Y"=1184.5139}, {"X"=226.85844, "Y"=1158.2439}, {"X"=240.55327, "Y"=1149.5544}, {"X"=246.15222, "Y"=1152.5964}, {"X"=251.65205, "Y"=1149.7102}, {"X"=255.64009, "Y"=1137.8772}, {"X"=252.31361, "Y"=1101.806}, {"X"=242.61084, "Y"=1024.8486}, {"X"=223.32297, "Y"=986.7963}, {"X"=201.55334, "Y"=976.91364}, {"X"=185.36604, "Y"=963.88275}, {"X"=176.81331, "Y"=918.5331}, {"X"=175.16206, "Y"=911.9796}, {"X"=179.34671, "Y"=905.50946}, {"X"=184.36852, "Y"=928.4173}, {"X"=193.59872, "Y"=947.9692}, {"X"=206.77463, "Y"=954.6199}, {"X"=217.0968, "Y"=964.4054}, {"X"=240.26675, "Y"=971.174}, {"X"=265.11005, "Y"=1003.26263}, {"X"=276.7269, "Y"=1022.26184}, {"X"=286.687, "Y"=1022.41846}, {"X"=303.86664, "Y"=1047.5436}, {"X"=316.64474, "Y"=1072.342}, {"X"=323.68475, "Y"=1081.6096}, {"X"=341.83792, "Y"=1112.1652}, {"X"=361.20966, "Y"=1133.4178}, {"X"=372.25693, "Y"=1139.533}, {"X"=387.19876, "Y"=1163.4238}, {"X"=419.1272, "Y"=1152.062}, {"X"=437.4271, "Y"=1196.2805}, {"X"=451.32196, "Y"=1239.6234}, {"X"=457.69733, "Y"=1253.9161}, {"X"=464.61642, "Y"=1248.3307}, {"X"=459.04782, "Y"=1253.9333}, {"X"=448.6864, "Y"=1236.7367}, {"X"=426.05588, "Y"=1216.3715}, {"X"=396.2439, "Y"=1204.4266}, {"X"=376.10492, "Y"=1169.1539}, {"X"=355.36404, "Y"=1180.5958}, {"X"=319.6076, "Y"=1185.953}, {"X"=304.4981, "Y"=1188.6658}, {"X"=290.73203, "Y"=1185.5609}, {"X"=278.32098, "Y"=1182.4698}, {"X"=256.49753, "Y"=1196.7538}, {"X"=233.36804, "Y"=1208.0476}, {"X"=227.88397, "Y"=1207.9749}, {"X"=230.56804, "Y"=1205.1145}, {"X"=221.09161, "Y"=1210.7775}, {"X"=221.02777, "Y"=1207.8838}, {"X"=230.10098, "Y"=1181.8132}, {"X"=238.58546, "Y"=1193.6035}, {"X"=245.55754, "Y"=1199.5128}, {"X"=249.53656, "Y"=1190.838}, {"X"=246.73737, "Y"=1187.8837}, {"X"=246.73737, "Y"=1187.8837}, {"X"=246.68893, "Y"=1184.9629}, {"X"=246.00458, "Y"=1143.693}, {"X"=240.51979, "Y"=1068.1299}, {"X"=235.1486, "Y"=1005.93146}, {"X"=224.04378, "Y"=951.69385}, {"X"=210.2182, "Y"=915.84406}, {"X"=198.23862, "Y"=902.5586}, {"X"=187.56743, "Y"=885.92566}, {"X"=173.8825, "Y"=869.12744}, {"X"=172.21114, "Y"=862.4439}, {"X"=211.45209, "Y"=906.06287}, {"X"=208.15308, "Y"=889.5832}, {"X"=211.3779, "Y"=902.78564}, {"X"=218.81438, "Y"=909.4611}, {"X"=208.15308, "Y"=889.5832}, {"X"=218.81438, "Y"=909.4611}, {"X"=220.27184, "Y"=909.48615}, {"X"=257.5718, "Y"=867.2887}, {"X"=279.62097, "Y"=871.0003}, {"X"=302.52512, "Y"=1062.9308}, {"X"=314.61902, "Y"=787.33624}, {"X"=317.95828, "Y"=1013.52625}, {"X"=317.99805, "Y"=1038.4716}, {"X"=313.79227, "Y"=1056.9513}, {"X"=311.07056, "Y"=1090.5496}, {"X"=306.86353, "Y"=1090.4872}, {"X"=303.96304, "Y"=1069.0887}, {"X"=302.62708, "Y"=1084.3418}, {"X"=303.97675, "Y"=1072.1511}, {"X"=319.3537, "Y"=991.51373}, {"X"=333.71124, "Y"=956.7266}, {"X"=359.88522, "Y"=918.4044}, {"X"=370.06396, "Y"=915.32214}, {"X"=386.60785, "Y"=866.26013}, {"X"=404.0229, "Y"=876.51416}, {"X"=420.08832, "Y"=876.798}, {"X"=420.08832, "Y"=876.798}, {"X"=405.27686, "Y"=889.7345}, {"X"=395.03186, "Y"=892.8445}, {"X"=388.52188, "Y"=829.4896}, {"X"=380.71426, "Y"=869.4752}, {"X"=371.7222, "Y"=892.43774}, {"X"=362.45453, "Y"=963.605}, {"X"=353.47705, "Y"=1026.5872}, {"X"=351.84412, "Y"=1066.7482}, {"X"=350.4209, "Y"=1069.7908}, {"X"=351.81155, "Y"=1072.8721}, {"X"=348.86966, "Y"=1100.2002}, {"X"=347.39087, "Y"=1118.2573}, {"X"=347.36417, "Y"=1124.2533}, {"X"=334.83975, "Y"=1124.073}, {"X"=304.2339, "Y"=1129.6174}, {"X"=269.43723, "Y"=1129.1193}, {"X"=244.3134, "Y"=1125.7666}, {"X"=208.19061, "Y"=1131.2332}, {"X"=170.72937, "Y"=1136.6715}, {"X"=160.87128, "Y"=1133.5464}, {"X"=150.99843, "Y"=1130.4166}, {"X"=151.85513, "Y"=1115.4271}, {"X"=147.8754, "Y"=1121.3816}, {"X"=209.82857, "Y"=1082.958}, {"X"=151.10674, "Y"=1133.4073}, {"X"=185.53802, "Y"=1070.366}, {"X"=186.06416, "Y"=1088.6956}, {"X"=189.6034, "Y"=1064.2897}, {"X"=192.84216, "Y"=1027.1893}, {"X"=191.58768, "Y"=1033.4005}, {"X"=195.69086, "Y"=1027.2339}, {"X"=201.1509, "Y"=1017.94476}, {"X"=211.06438, "Y"=1014.9687}, {"X"=219.0857, "Y"=989.8958}, {"X"=232.23076, "Y"=1002.73755}, {"X"=245.09996, "Y"=1002.9431}, {"X"=265.18713, "Y"=1009.552}, {"X"=283.89462, "Y"=1028.6135}, {"X"=295.29947, "Y"=1035.0142}, {"X"=306.6963, "Y"=1047.5872}, {"X"=316.61008, "Y"=1053.9133}, {"X"=325.08728, "Y"=1069.408}, {"X"=332.11038, "Y"=1081.7356}, {"X"=333.51447, "Y"=1081.7566}, {"X"=336.40836, "Y"=1041.8569}, {"X"=344.92416, "Y"=1035.7863}, {"X"=340.6919, "Y"=1029.5018}, {"X"=326.49762, "Y"=1050.9803}, {"X"=326.4915, "Y"=1096.8439}, {"X"=325.0929, "Y"=1105.8934}, {"X"=327.916, "Y"=1038.6255}, {"X"=312.51437, "Y"=1105.7094}, {"X"=312.53918, "Y"=1114.7477}, {"X"=306.9695, "Y"=1117.6722}, {"X"=290.341, "Y"=1132.406}, {"X"=273.71133, "Y"=1138.1338}, {"X"=255.50964, "Y"=1128.9198}, {"X"=227.51732, "Y"=1122.5281}, {"X"=216.41745, "Y"=1125.3661}, {"X"=216.553, "Y"=1131.3525}, {"X"=206.72292, "Y"=1128.2214}, {"X"=215.02211, "Y"=1125.3461}, {"X"=230.78053, "Y"=1146.4495}, {"X"=249.06708, "Y"=1161.5056}, {"X"=257.41125, "Y"=1164.57}, {"X"=258.5041, "Y"=1143.8695}, {"X"=258.71136, "Y"=1158.6874}, {"X"=250.9119, "Y"=1190.8566}, {"X"=233.19867, "Y"=1199.3474}, {"X"=214.86548, "Y"=1178.6774}, {"X"=210.86633, "Y"=1184.4764}, {"X"=207.52806, "Y"=1216.3739}, {"X"=208.52745, "Y"=1256.4287}, {"X"=209.4639, "Y"=1239.363}, {"X"=215.18214, "Y"=1250.8345}, {"X"=217.63895, "Y"=1239.4681}, {"X"=214.44196, "Y"=1219.3474}, {"X"=211.96573, "Y"=1172.7697}, {"X"=201.61427, "Y"=1091.9658}, {"X"=183.39325, "Y"=995.6468}, {"X"=171.4702, "Y"=1026.8551}, {"X"=181.62784, "Y"=1033.2455}, {"X"=169.7909, "Y"=973.20953}, {"X"=169.7909, "Y"=973.20953}, {"X"=189.47546, "Y"=1008.3491}, {"X"=208.43304, "Y"=1024.3126}, {"X"=234.01115, "Y"=1021.5902}, {"X"=248.49991, "Y"=1037.3931}, {"X"=261.31512, "Y"=1040.6947}, {"X"=284.15808, "Y"=1059.5771}, {"X"=301.1765, "Y"=1075.1675}, {"X"=313.91217, "Y"=1105.7299}, {"X"=326.48624, "Y"=1135.9044}, {"X"=348.61444, "Y"=1154.0314}, {"X"=373.17554, "Y"=1186.6803}, {"X"=385.56314, "Y"=1183.9302}, {"X"=388.11856, "Y"=1198.5208}, {"X"=395.34265, "Y"=1172.3556}, {"X"=410.9448, "Y"=1146.022}, {"X"=417.93695, "Y"=1213.3826}, {"X"=428.21588, "Y"=1304.017}, {"X"=442.7117, "Y"=1312.4973}, {"X"=445.87964, "Y"=1293.1094}, {"X"=441.4463, "Y"=1309.7168}, {"X"=437.50757, "Y"=1306.9009}, {"X"=436.83255, "Y"=1279.0221}, {"X"=439.53864, "Y"=1222.3008}, {"X"=287.2968, "Y"=1099.2943}, {"X"=287.20053, "Y"=1087.1555}, {"X"=287.0795, "Y"=1071.8965}, {"X"=283.09503, "Y"=1099.2325}, {"X"=281.74927, "Y"=1105.2593}, {"X"=277.28015, "Y"=1077.8639}, {"X"=278.95123, "Y"=1105.2183}, {"X"=283.01498, "Y"=1090.1335}, {"X"=287.84518, "Y"=987.84015}, {"X"=309.24368, "Y"=962.7263}, {"X"=319.31213, "Y"=959.6922}, {"X"=312.09546, "Y"=953.15894}, {"X"=303.3281, "Y"=927.1896}, {"X"=298.8748, "Y"=907.56964}, {"X"=291.46365, "Y"=887.7433}, {"X"=285.6962, "Y"=897.5116}, {"X"=267.10944, "Y"=929.81866}, {"X"=261.47498, "Y"=942.6586}, {"X"=260.15518, "Y"=952.2947}, {"X"=265.81424, "Y"=942.7314}, {"X"=266.04498, "Y"=962.013}, {"X"=269.28876, "Y"=993.8678}, {"X"=270.7903, "Y"=1000.20355}, {"X"=270.92996, "Y"=1012.78107}, {"X"=271.2416, "Y"=1040.8484}, {"X"=271.5497, "Y"=1068.5989}, {"X"=270.3486, "Y"=1086.9049}, {"X"=267.61197, "Y"=1092.942}, {"X"=263.59695, "Y"=1108.012}, {"X"=258.54565, "Y"=1146.8403}, {"X"=241.12808, "Y"=1181.9635}, {"X"=227.52446, "Y"=1190.5409}, {"X"=212.86757, "Y"=1210.6686}, {"X"=198.61424, "Y"=1190.1505}, {"X"=196.92146, "Y"=1178.4323}, {"X"=196.80728, "Y"=1224.8717}, {"X"=200.37999, "Y"=1256.3258}, {"X"=201.51297, "Y"=1247.8159}, {"X"=205.8842, "Y"=1259.2297}, {"X"=219.19499, "Y"=1248.0413}, {"X"=236.38234, "Y"=1222.5134}, {"X"=267.55453, "Y"=1202.7089}, {"X"=304.44577, "Y"=1176.9719}, {"X"=334.77884, "Y"=1156.794}, {"X"=364.05698, "Y"=1124.4937}, {"X"=372.40063, "Y"=1124.6138}, {"X"=369.59253, "Y"=1127.5651}, {"X"=373.91016, "Y"=1112.632}, {"X"=375.15094, "Y"=1127.6449}, {"X"=372.37183, "Y"=1127.605}, {"X"=368.97702, "Y"=1039.2627}, {"X"=367.48312, "Y"=1048.523}, {"X"=359.8634, "Y"=1127.4254}, {"X"=357.10254, "Y"=1124.3936}, {"X"=352.96286, "Y"=1118.338}, {"X"=348.81244, "Y"=1112.2667}, {"X"=347.40424, "Y"=1115.2537}, {"X"=347.39087, "Y"=1118.2573}, {"X"=353.01343, "Y"=1109.3168}, {"X"=366.96576, "Y"=1109.5204}, {"X"=368.86856, "Y"=1051.631}, {"X"=383.63556, "Y"=995.7081}, {"X"=411.3948, "Y"=958.0159}, {"X"=424.77, "Y"=935.722}, {"X"=425.41034, "Y"=903.21295}, {"X"=411.83533, "Y"=932.2698}, {"X"=407.60684, "Y"=925.71783}, {"X"=428.58105, "Y"=890.14215}, {"X"=413.5621, "Y"=916.0682}, {"X"=403.267, "Y"=925.644}, {"X"=407.29187, "Y"=945.10345}, {"X"=425.28162, "Y"=909.7484}, {"X"=417.67203, "Y"=929.131}, {"X"=416.0525, "Y"=938.8041}, {"X"=409.52893, "Y"=983.47644}, {"X"=403.36456, "Y"=1011.74725}, {"X"=397.4044, "Y"=1030.3889}, {"X"=397.58554, "Y"=1017.9167}, {"X"=392.11346, "Y"=1002.1462}, {"X"=384.50336, "Y"=1042.6013}, {"X"=379.88773, "Y"=1076.3507}, {"X"=378.38504, "Y"=1085.4714}, {"X"=380.91296, "Y"=1109.7239}, {"X"=392.837, "Y"=1154.6506}, {"X"=403.59763, "Y"=1172.4692}, {"X"=405.11905, "Y"=1163.6727}, {"X"=400.617, "Y"=1187.053}, {"X"=410.37177, "Y"=1178.4225}, {"X"=415.81128, "Y"=1181.4213}, {"X"=423.27377, "Y"=1284.4562}, {"X"=432.60944, "Y"=1345.3094}, {"X"=432.54642, "Y"=1348.032}, {"X"=433.93445, "Y"=1345.3247}, {"X"=433.93445, "Y"=1345.3247}, {"X"=425.48233, "Y"=1306.7566}, {"X"=422.97726, "Y"=1233.547}, {"X"=420.04443, "Y"=1175.6271}, {"X"=417.63315, "Y"=1157.951}] {"Y" format="%.2f"; "X" format="%.2f"}
  in  "manual bottom huyun vs chen jin":T1[](array[typedef])=[{"X"=377.4669, "Y"=1039.3944}, {"X"=374.69873, "Y"=1033.1436}, {"X"=384.94998, "Y"=1005.1765}, {"X"=392.32446, "Y"=986.3656}, {"X"=390.85345, "Y"=989.5066}, {"X"=390.85345, "Y"=989.5066}, {"X"=389.223, "Y"=1005.24475}, {"X"=386.4128, "Y"=1002.0549}, {"X"=380.7113, "Y"=1001.9636}, {"X"=369.14075, "Y"=1020.59296}, {"X"=369.16815, "Y"=1017.4675}, {"X"=364.7805, "Y"=1032.9889}, {"X"=354.75015, "Y"=1051.4142}, {"X"=353.28625, "Y"=1060.6302}, {"X"=342.03912, "Y"=1051.219}, {"X"=332.11823, "Y"=1075.6326}, {"X"=329.29773, "Y"=1087.7816}, {"X"=322.28476, "Y"=1087.6774}, {"X"=312.44772, "Y"=1081.4415}, {"X"=306.79224, "Y"=1072.1936}, {"X"=329.29343, "Y"=1093.8545}, {"X"=355.74854, "Y"=1118.3783}, {"X"=363.82178, "Y"=1154.2443}, {"X"=380.03775, "Y"=1186.7736}, {"X"=378.5366, "Y"=1198.3921}, {"X"=396.07288, "Y"=1215.9758}, {"X"=398.71106, "Y"=1221.7651}, {"X"=396.11554, "Y"=1213.0939}, {"X"=385.30856, "Y"=1204.2808}, {"X"=381.1733, "Y"=1207.1193}, {"X"=377.2616, "Y"=1189.651}, {"X"=371.94385, "Y"=1172.0333}, {"X"=366.61118, "Y"=1151.3246}, {"X"=358.43298, "Y"=1133.3782}, {"X"=358.47333, "Y"=1127.4054}, {"X"=348.86966, "Y"=1100.2002}, {"X"=339.13028, "Y"=1081.8406}, {"X"=337.76367, "Y"=1066.5348}, {"X"=340.63583, "Y"=1048.1096}, {"X"=342.03912, "Y"=1051.219}, {"X"=340.61722, "Y"=1054.281}, {"X"=340.5617, "Y"=1072.7025}, {"X"=357.27777, "Y"=1097.2981}, {"X"=373.7614, "Y"=1127.6249}, {"X"=385.7831, "Y"=1166.3477}, {"X"=389.6428, "Y"=1186.9039}, {"X"=396.1583, "Y"=1210.2083}, {"X"=401.38843, "Y"=1224.6721}, {"X"=403.9677, "Y"=1233.3004}, {"X"=393.46918, "Y"=1207.2828}, {"X"=372.85938, "Y"=1218.5494}, {"X"=377.07382, "Y"=1207.0647}, {"X"=363.52026, "Y"=1192.377}, {"X"=360.97076, "Y"=1166.004}, {"X"=352.8623, "Y"=1136.2799}, {"X"=347.32425, "Y"=1133.2196}, {"X"=337.6599, "Y"=1109.0928}, {"X"=327.8914, "Y"=1096.8645}, {"X"=330.68805, "Y"=1099.9327}, {"X"=323.6928, "Y"=1099.8298}, {"X"=333.51447, "Y"=1081.7566}, {"X"=350.35947, "Y"=1082.0084}, {"X"=374.51447, "Y"=1051.7177}, {"X"=381.8169, "Y"=1030.145}, {"X"=387.56375, "Y"=1024.0045}, {"X"=401.9426, "Y"=1011.7247}, {"X"=400.5206, "Y"=1011.7021}, {"X"=399.33136, "Y"=995.96075}, {"X"=394.65765, "Y"=1024.1161}, {"X"=387.4081, "Y"=1036.4473}, {"X"=375.92578, "Y"=1051.7393}, {"X"=367.32657, "Y"=1066.9828}, {"X"=361.85532, "Y"=1045.3455}, {"X"=356.23868, "Y"=1039.0651}, {"X"=347.70276, "Y"=1048.2184}, {"X"=346.2766, "Y"=1051.284}, {"X"=330.7215, "Y"=1066.4281}, {"X"=302.5835, "Y"=1075.1886}, {"X"=262.0394, "Y"=1095.8931}, {"X"=245.60818, "Y"=1119.7882}, {"X"=230.48622, "Y"=1131.5514}, {"X"=206.21782, "Y"=1163.861}, {"X"=174.54639, "Y"=1169.315}, {"X"=155.47987, "Y"=1177.8665}, {"X"=144.37534, "Y"=1212.6543}, {"X"=133.62842, "Y"=1218.287}, {"X"=124.51923, "Y"=1229.676}, {"X"=123.88695, "Y"=1246.8265}, {"X"=121.53461, "Y"=1223.8898}, {"X"=138.77112, "Y"=1209.688}, {"X"=154.83243, "Y"=1198.2982}, {"X"=178.78851, "Y"=1172.3141}, {"X"=195.13991, "Y"=1163.7076}, {"X"=204.53471, "Y"=1152.0137}, {"X"=213.69627, "Y"=1128.3213}, {"X"=231.41148, "Y"=1107.5422}, {"X"=247.86772, "Y"=1086.5706}, {"X"=253.48918, "Y"=1086.6542}, {"X"=253.30789, "Y"=1074.4479}, {"X"=244.90494, "Y"=1077.3785}, {"X"=214.60825, "Y"=1107.2971}, {"X"=192.6898, "Y"=1125.0255}, {"X"=181.10983, "Y"=1157.6068}, {"X"=162.49019, "Y"=1180.8927}, {"X"=150.8104, "Y"=1201.1505}, {"X"=132.68779, "Y"=1195.0916}, {"X"=131.00456, "Y"=1221.1348}, {"X"=134.5599, "Y"=1241.2577}, {"X"=132.65002, "Y"=1261.141}, {"X"=128.335, "Y"=1255.4156}, {"X"=133.0786, "Y"=1238.381}, {"X"=144.37534, "Y"=1212.6543}, {"X"=160.43816, "Y"=1201.2789}, {"X"=185.87477, "Y"=1178.2815}, {"X"=191.0678, "Y"=1166.5986}, {"X"=205.40274, "Y"=1131.1934}, {"X"=221.93385, "Y"=1122.4478}, {"X"=241.36763, "Y"=1116.7227}, {"X"=248.06213, "Y"=1098.7172}, {"X"=257.70474, "Y"=1086.7169}, {"X"=295.33798, "Y"=1041.2213}, {"X"=335.0218, "Y"=1026.2977}, {"X"=370.73163, "Y"=1001.80383}, {"X"=390.9363, "Y"=983.17413}, {"X"=403.8091, "Y"=983.3834}, {"X"=411.17624, "Y"=970.7904}, {"X"=412.6651, "Y"=967.6265}, {"X"=409.95767, "Y"=957.99207}, {"X"=401.14078, "Y"=970.6255}, {"X"=383.7091, "Y"=989.39105}, {"X"=372.2754, "Y"=989.20605}, {"X"=363.62567, "Y"=998.5401}, {"X"=354.9515, "Y"=1017.24286}, {"X"=340.65448, "Y"=1041.9226}, {"X"=333.5822, "Y"=1038.7134}, {"X"=330.73376, "Y"=1054.1296}, {"X"=333.55786, "Y"=1054.173}, {"X"=337.71158, "Y"=1087.9067}, {"X"=361.38544, "Y"=1109.439}, {"X"=387.5398, "Y"=1136.7737}, {"X"=407.87524, "Y"=1163.7109}, {"X"=432.34534, "Y"=1178.7233}, {"X"=444.12094, "Y"=1202.1709}, {"X"=454.8889, "Y"=1208.1005}, {"X"=450.9495, "Y"=1202.2623}, {"X"=440.02325, "Y"=1202.1161}, {"X"=415.70135, "Y"=1187.2578}, {"X"=396.4158, "Y"=1192.8212}, {"X"=388.27078, "Y"=1186.8854}, {"X"=380.27066, "Y"=1166.2714}, {"X"=373.46667, "Y"=1157.3342}, {"X"=364.03333, "Y"=1127.4852}, {"X"=358.55432, "Y"=1115.4155}, {"X"=354.42664, "Y"=1106.3228}, {"X"=353.14917, "Y"=1085.0951}, {"X"=343.38547, "Y"=1069.6844}, {"X"=346.32816, "Y"=1038.9113}, {"X"=346.34106, "Y"=1035.8082}, {"X"=291.15237, "Y"=1050.4376}, {"X"=292.60864, "Y"=1056.6278}, {"X"=296.8281, "Y"=1053.6105}, {"X"=291.19598, "Y"=1056.6062}, {"X"=292.56683, "Y"=1050.4594}, {"X"=289.78326, "Y"=1056.5846}, {"X"=296.99133, "Y"=1081.2104}, {"X"=298.39673, "Y"=1081.2314}, {"X"=299.60522, "Y"=1044.3845}, {"X"=323.6464, "Y"=994.7427}, {"X"=322.19373, "Y"=962.9402}, {"X"=303.29904, "Y"=920.69147}, {"X"=306.07416, "Y"=887.9989}, {"X"=306.04843, "Y"=881.39935}, {"X"=313.35297, "Y"=878.2221}, {"X"=305.89267, "Y"=841.43835}, {"X"=308.77374, "Y"=821.2754}, {"X"=305.84018, "Y"=827.97784}, {"X"=301.34128, "Y"=814.36426}, {"X"=293.9509, "Y"=817.6177}, {"X"=293.90878, "Y"=810.8327}, {"X"=293.8031, "Y"=793.7917}, {"X"=323.66025, "Y"=1026.1196}, {"X"=317.95328, "Y"=1010.3903}, {"X"=319.38657, "Y"=1016.6807}, {"X"=319.3988, "Y"=1026.0527}, {"X"=310.89334, "Y"=1032.1482}, {"X"=309.5052, "Y"=1041.4406}, {"X"=300.98984, "Y"=1038.2076}, {"X"=306.63586, "Y"=1032.0818}, {"X"=303.90805, "Y"=1056.8004}, {"X"=308.14447, "Y"=1056.8651}, {"X"=299.7368, "Y"=1069.0248}, {"X"=285.89627, "Y"=1099.2738}, {"X"=276.02896, "Y"=1093.0665}, {"X"=248.30379, "Y"=1113.8154}, {"X"=219.66882, "Y"=1146.293}, {"X"=190.35014, "Y"=1190.039}, {"X"=170.15855, "Y"=1204.3104}, {"X"=166.3283, "Y"=1212.944}, {"X"=170.25351, "Y"=1207.21}, {"X"=177.39046, "Y"=1215.9773}, {"X"=204.27141, "Y"=1196.0526}, {"X"=222.1463, "Y"=1196.2926}, {"X"=242.70998, "Y"=1193.659}, {"X"=257.24255, "Y"=1152.7518}, {"X"=283.4908, "Y"=1144.2223}, {"X"=290.29703, "Y"=1126.4268}, {"X"=276.24554, "Y"=1114.221}, {"X"=284.64966, "Y"=1117.3492}, {"X"=287.48798, "Y"=1123.3914}, {"X"=309.838, "Y"=1141.6223}, {"X"=344.47742, "Y"=1151.0138}, {"X"=367.83893, "Y"=1169.0398}, {"X"=399.11108, "Y"=1195.7646}, {"X"=417.54694, "Y"=1233.4766}, {"X"=441.41806, "Y"=1256.5417}, {"X"=440.13657, "Y"=1253.693}, {"X"=431.12128, "Y"=1233.6526}, {"X"=412.16806, "Y"=1230.5458}, {"X"=399.93784, "Y"=1230.3866}, {"X"=394.70944, "Y"=1215.9579}, {"X"=386.82422, "Y"=1192.6917}, {"X"=376.10492, "Y"=1169.1539}, {"X"=362.50723, "Y"=1145.338}, {"X"=359.9267, "Y"=1118.4387}, {"X"=350.26788, "Y"=1100.2208}, {"X"=340.52493, "Y"=1084.9069}, {"X"=336.32904, "Y"=1078.7491}, {"X"=319.4553, "Y"=1069.3229}, {"X"=302.52512, "Y"=1062.9308}, {"X"=299.6876, "Y"=1059.8137}, {"X"=262.73334, "Y"=1040.7167}, {"X"=218.33669, "Y"=1021.34375}, {"X"=181.26227, "Y"=1020.76086}, {"X"=325.08157, "Y"=1032.3695}, {"X"=320.813, "Y"=1019.8311}, {"X"=323.66437, "Y"=1035.4554}, {"X"=322.2489, "Y"=1038.5376}, {"X"=323.66162, "Y"=1029.2355}, {"X"=320.81616, "Y"=1022.9551}, {"X"=313.69308, "Y"=1016.59076}, {"X"=309.4639, "Y"=1029.0134}, {"X"=312.27817, "Y"=1019.6966}, {"X"=300.91122, "Y"=1022.6421}, {"X"=294.02127, "Y"=1056.6494}, {"X"=289.8737, "Y"=1068.8757}, {"X"=306.8398, "Y"=1084.4045}, {"X"=327.87994, "Y"=1123.9729}, {"X"=348.60043, "Y"=1156.9869}, {"X"=367.60828, "Y"=1195.3406}, {"X"=383.76508, "Y"=1218.693}, {"X"=390.38364, "Y"=1233.1243}, {"X"=393.01953, "Y"=1238.8716}, {"X"=378.24896, "Y"=1224.3694}, {"X"=361.92865, "Y"=1221.2825}, {"X"=360.5446, "Y"=1224.1378}, {"X"=353.86902, "Y"=1200.9628}, {"X"=348.53064, "Y"=1171.7109}, {"X"=338.99872, "Y"=1130.1151}, {"X"=332.09085, "Y"=1096.9265}, {"X"=334.92987, "Y"=1075.6748}, {"X"=354.75015, "Y"=1051.4142}, {"X"=385.21368, "Y"=983.08105}, {"X"=408.7328, "Y"=945.12756}, {"X"=431.49307, "Y"=890.1931}, {"X"=450.5776, "Y"=883.9404}, {"X"=455.6231, "Y"=857.5123}, {"X"=464.86316, "Y"=840.96564}, {"X"=477.30765, "Y"=817.613}, {"X"=464.39243, "Y"=803.80084}, {"X"=452.63672, "Y"=800.1765}, {"X"=428.52432, "Y"=820.0962}, {"X"=417.82626, "Y"=840.1119}, {"X"=413.2417, "Y"=850.076}, {"X"=401.10117, "Y"=876.4625}, {"X"=370.20728, "Y"=898.9792}, {"X"=352.61612, "Y"=921.5331}, {"X"=327.95737, "Y"=940.5485}, {"X"=310.70218, "Y"=969.1397}, {"X"=283.7082, "Y"=1006.70496}, {"X"=285.4178, "Y"=1041.0677}, {"X"=271.276, "Y"=1043.9473}, {"X"=265.60764, "Y"=1043.8597}, {"X"=267.0248, "Y"=1043.8816}, {"X"=264.4997, "Y"=1068.4923}, {"X"=268.8371, "Y"=1077.7373}, {"X"=270.1747, "Y"=1071.6417}, {"X"=281.50098, "Y"=1077.9272}, {"X"=302.45172, "Y"=1047.5217}, {"X"=319.41504, "Y"=1038.4935}, {"X"=350.4363, "Y"=1066.7268}, {"X"=348.97043, "Y"=1078.9387}, {"X"=351.82782, "Y"=1069.812}, {"X"=351.87674, "Y"=1060.6088}, {"X"=361.81003, "Y"=1051.5226}, {"X"=361.76486, "Y"=1057.6841}, {"X"=288.34695, "Y"=1053.4806}, {"X"=292.62952, "Y"=1059.7062}, {"X"=286.8351, "Y"=1041.0897}, {"X"=286.85968, "Y"=1044.1879}, {"X"=286.93323, "Y"=1053.4589}, {"X"=296.80984, "Y"=1050.5244}, {"X"=309.49487, "Y"=1038.3396}, {"X"=316.58682, "Y"=1041.5502}, {"X"=317.99805, "Y"=1038.4716}, {"X"=307.90787, "Y"=991.32904}, {"X"=280.27487, "Y"=942.9738}, {"X"=250.71983, "Y"=900.18695}, {"X"=231.07027, "Y"=863.4916}, {"X"=202.88234, "Y"=852.98035}, {"X"=201.32643, "Y"=849.6072}, {"X"=199.35353, "Y"=829.40704}, {"X"=197.6191, "Y"=819.2331}, {"X"=196.3057, "Y"=825.9751}, {"X"=203.71661, "Y"=826.1106}, {"X"=218.816, "Y"=839.86163}, {"X"=216.2924, "Y"=859.89703}, {"X"=217.62267, "Y"=853.2447}, {"X"=215.78847, "Y"=836.4446}, {"X"=213.05342, "Y"=846.4688}, {"X"=393.1539, "Y"=1030.3224}, {"X"=391.82025, "Y"=1024.0714}, {"X"=394.9196, "Y"=1005.33575}, {"X"=397.81323, "Y"=1002.2374}, {"X"=400.71033, "Y"=999.1354}, {"X"=400.7579, "Y"=995.98376}, {"X"=399.1915, "Y"=1005.404}, {"X"=396.29892, "Y"=1008.4984}, {"X"=393.45264, "Y"=1008.45306}, {"X"=391.90375, "Y"=1017.8269}, {"X"=383.48895, "Y"=1008.2944}, {"X"=383.30676, "Y"=1023.93756}, {"X"=374.79138, "Y"=1023.8037}, {"X"=370.56122, "Y"=1020.61536}, {"X"=359.11176, "Y"=1032.9004}, {"X"=359.15378, "Y"=1026.6761}, {"X"=357.57425, "Y"=1051.4575}, {"X"=354.5875, "Y"=1079.023}, {"X"=347.40424, "Y"=1115.2537}, {"X"=345.8735, "Y"=1148.0701}, {"X"=349.9083, "Y"=1171.7299}, {"X"=355.23807, "Y"=1200.9811}, {"X"=362.03848, "Y"=1206.8645}, {"X"=366.04172, "Y"=1218.4597}, {"X"=375.34564, "Y"=1241.4958}, {"X"=394.12875, "Y"=1255.9425}, {"X"=414.50958, "Y"=1250.5305}, {"X"=443.41092, "Y"=1284.7039}, {"X"=440.4523, "Y"=1295.8285}, {"X"=436.6997, "Y"=1284.6213}, {"X"=433.12177, "Y"=1264.9144}, {"X"=420.37656, "Y"=1227.7883}, {"X"=394.91922, "Y"=1201.5123}, {"X"=388.50058, "Y"=1169.3251}, {"X"=398.49533, "Y"=1145.8462}, {"X"=408.94684, "Y"=1101.0841}, {"X"=423.5121, "Y"=1070.8954}, {"X"=426.44638, "Y"=1064.8136}, {"X"=430.86127, "Y"=1055.6631}, {"X"=429.71365, "Y"=1043.301}, {"X"=416.83188, "Y"=1052.3674}, {"X"=408.1137, "Y"=1067.6008}, {"X"=395.50397, "Y"=1064.3435}, {"X"=391.24158, "Y"=1067.3451}, {"X"=382.69583, "Y"=1076.3928}, {"X"=377.14362, "Y"=1070.1946}, {"X"=374.33157, "Y"=1070.1521}, {"X"=367.4047, "Y"=1057.7703}, {"X"=353.3035, "Y"=1057.5548}, {"X"=348.98492, "Y"=1075.8861}, {"X"=344.81644, "Y"=1063.5734}, {"X"=340.60794, "Y"=1057.361}, {"X"=356.0294, "Y"=1072.9357}, {"X"=365.79413, "Y"=1082.2393}, {"X"=373.8208, "Y"=1121.6389}, {"X"=374.93823, "Y"=1148.4794}, {"X"=372.1141, "Y"=1154.3605}, {"X"=366.23798, "Y"=1195.3221}, {"X"=367.17944, "Y"=1244.2397}, {"X"=373.90176, "Y"=1250.013}, {"X"=365.84738, "Y"=1241.3737}, {"X"=331.92404, "Y"=1226.6344}, {"X"=307.39304, "Y"=1226.3143}, {"X"=304.5761, "Y"=1206.0996}, {"X"=297.60916, "Y"=1185.6543}, {"X"=294.6869, "Y"=1159.1885}, {"X"=290.4068, "Y"=1141.3472}, {"X"=290.20874, "Y"=1114.4236}, {"X"=280.29358, "Y"=1099.1913}, {"X"=287.2968, "Y"=1099.2943}, {"X"=275.96674, "Y"=1086.9885}, {"X"=271.7532, "Y"=1086.9258}, {"X"=243.65108, "Y"=1086.5079}, {"X"=214.67744, "Y"=1110.3146}, {"X"=201.22055, "Y"=1131.1335}, {"X"=177.42082, "Y"=1127.8019}, {"X"=171.01686, "Y"=1145.6078}, {"X"=163.57263, "Y"=1172.1051}, {"X"=162.6903, "Y"=1186.7457}, {"X"=159.26639, "Y"=1207.0641}, {"X"=152.71468, "Y"=1215.6526}, {"X"=152.18594, "Y"=1201.1688}, {"X"=163.1885, "Y"=1201.3157}, {"X"=176.38971, "Y"=1184.0083}, {"X"=189.51585, "Y"=1160.6786}, {"X"=215.7051, "Y"=1155.1311}, {"X"=216.48526, "Y"=1128.3612}, {"X"=237.17642, "Y"=1116.662}, {"X"=256.64548, "Y"=1110.9254}, {"X"=276.15295, "Y"=1105.1774}, {"X"=274.75375, "Y"=1105.1569}, {"X"=285.6962, "Y"=1074.9348}, {"X"=282.4187, "Y"=1022.3513}, {"X"=257.92163, "Y"=999.9975}, {"X"=236.12173, "Y"=980.6566}, {"X"=204.9416, "Y"=938.4808}, {"X"=179.8202, "Y"=921.8406}, {"X"=181.08826, "Y"=915.34576}, {"X"=176.71684, "Y"=915.27094}, {"X"=185.45917, "Y"=915.42053}, {"X"=195.4873, "Y"=909.06006}, {"X"=207.91663, "Y"=941.7607}, {"X"=213.8545, "Y"=948.30707}, {"X"=231.20802, "Y"=948.59656}, {"X"=260.6158, "Y"=987.39966}, {"X"=276.41406, "Y"=990.82086}, {"X"=289.3939, "Y"=1003.65045}, {"X"=295.14447, "Y"=1010.0279}, {"X"=309.45355, "Y"=1025.8969}, {"X"=319.4272, "Y"=1047.7831}, {"X"=320.83832, "Y"=1044.7124}, {"X"=339.1469, "Y"=1075.7383}, {"X"=348.98492, "Y"=1075.8861}, {"X"=360.1394, "Y"=1088.2402}, {"X"=379.58524, "Y"=1103.6733}, {"X"=406.69577, "Y"=1151.8875}, {"X"=432.21515, "Y"=1184.5654}, {"X"=446.48526, "Y"=1216.6411}, {"X"=467.4909, "Y"=1242.6805}, {"X"=464.78394, "Y"=1242.6458}, {"X"=470.37213, "Y"=1237.0171}, {"X"=454.5758, "Y"=1219.6248}, {"X"=425.35815, "Y"=1184.472}, {"X"=390.1934, "Y"=1145.729}, {"X"=364.1519, "Y"=1112.49}, {"X"=353.0303, "Y"=1106.3022}, {"X"=323.70612, "Y"=1129.8962}, {"X"=297.41785, "Y"=1153.3145}, {"X"=286.3149, "Y"=1150.197}, {"X"=272.55212, "Y"=1158.8801}, {"X"=248.0184, "Y"=1182.0573}, {"X"=227.52446, "Y"=1190.5409}, {"X"=220.89986, "Y"=1202.086}, {"X"=219.46187, "Y"=1199.1635}, {"X"=216.58047, "Y"=1193.3073}, {"X"=220.1257, "Y"=1166.9999}, {"X"=247.6351, "Y"=1158.5332}, {"X"=253.21834, "Y"=1161.5632}, {"X"=259.93338, "Y"=1146.86}, {"X"=265.2595, "Y"=1129.0594}, {"X"=269.43723, "Y"=1129.1193}, {"X"=270.8297, "Y"=1129.1392}, {"X"=274.72192, "Y"=1102.1348}, {"X"=267.31985, "Y"=1068.5349}, {"X"=260.82306, "Y"=1003.1942}, {"X"=253.21544, "Y"=971.3862}, {"X"=230.96413, "Y"=935.6851}, {"X"=206.45651, "Y"=879.6484}, {"X"=200.26268, "Y"=866.2711}, {"X"=186.47876, "Y"=845.9899}, {"X"=189.1634, "Y"=835.9613}, {"X"=185.55836, "Y"=812.2266}, {"X"=182.67949, "Y"=815.5683}, {"X"=190.37592, "Y"=825.86664}, {"X"=190.55414, "Y"=832.6188}, {"X"=205.7522, "Y"=849.6867}, {"X"=225.18845, "Y"=863.3869}, {"X"=241.52655, "Y"=873.643}, {"X"=245.87534, "Y"=870.4026}, {"X"=256.01224, "Y"=860.6058}, {"X"=280.91165, "Y"=851.0377}, {"X"=327.91467, "Y"=1041.7255}, {"X"=325.0835, "Y"=1044.7778}, {"X"=322.24435, "Y"=1032.3253}, {"X"=325.08206, "Y"=1035.4775}, {"X"=317.99307, "Y"=1035.3672}, {"X"=316.56927, "Y"=1032.2368}, {"X"=312.32095, "Y"=1035.2789}, {"X"=300.94272, "Y"=1028.8801}, {"X"=292.29242, "Y"=1009.9826}, {"X"=294.909, "Y"=972.06946}, {"X"=310.59494, "Y"=933.79315}, {"X"=329.42764, "Y"=904.82544}, {"X"=368.9193, "Y"=879.2015}, {"X"=394.15158, "Y"=849.73206}, {"X"=398.60547, "Y"=846.4669}, {"X"=413.58612, "Y"=829.94794}, {"X"=421.64685, "Y"=792.77075}, {"X"=415.23608, "Y"=819.85144}, {"X"=401.89316, "Y"=822.98627}, {"X"=375.01968, "Y"=852.7293}, {"X"=369.28683, "Y"=835.8709}, {"X"=367.64853, "Y"=855.9348}, {"X"=355.7662, "Y"=878.96967}, {"X"=351.16653, "Y"=921.5083}, {"X"=343.76733, "Y"=963.29645}, {"X"=342.21417, "Y"=998.19635}, {"X"=339.3241, "Y"=1010.72986}, {"X"=337.87686, "Y"=1020.1001}, {"X"=337.8087, "Y"=1048.0662}, {"X"=337.69678, "Y"=1093.9788}, {"X"=340.50662, "Y"=1090.9862}, {"X"=332.08694, "Y"=1099.9534}, {"X"=319.49506, "Y"=1099.7681}, {"X"=280.2652, "Y"=1096.162}, {"X"=229.71239, "Y"=1092.3815}, {"X"=179.30391, "Y"=1097.7056}, {"X"=150.01752, "Y"=1103.3317}, {"X"=131.15643, "Y"=1087.8812}, {"X"=126.14495, "Y"=1102.9823}, {"X"=114.90562, "Y"=1102.8179}, {"X"=116.83209, "Y"=1114.9202}, {"X"=116.44131, "Y"=1105.8645}, {"X"=175.74556, "Y"=1026.9219}, {"X"=184.56308, "Y"=1036.4009}, {"X"=188.65556, "Y"=1030.2413}, {"X"=194.94536, "Y"=998.9892}, {"X"=198.43167, "Y"=967.2953}, {"X"=196.99014, "Y"=967.2716}, {"X"=202.59804, "Y"=960.96533}, {"X"=206.77463, "Y"=954.6199}, {"X"=215.37195, "Y"=951.5495}, {"X"=222.79718, "Y"=961.2989}, {"X"=233.07114, "Y"=971.05615}, {"X"=257.61795, "Y"=977.82764}, {"X"=276.50833, "Y"=1000.2951}, {"X"=289.3939, "Y"=1003.65045}, {"X"=296.589, "Y"=1013.1876}, {"X"=305.16434, "Y"=1019.5845}, {"X"=312.3124, "Y"=1032.1704}, {"X"=322.2489, "Y"=1038.5376}, {"X"=330.73685, "Y"=1051.0454}, {"X"=334.95267, "Y"=1063.4235}, {"X"=333.55786, "Y"=1054.173}, {"X"=332.13397, "Y"=1063.3806}, {"X"=332.13794, "Y"=1060.3081}, {"X"=332.13004, "Y"=1066.4495}, {"X"=339.1469, "Y"=1075.7383}, {"X"=326.49475, "Y"=1072.4906}, {"X"=318.04718, "Y"=1069.3015}, {"X"=323.68207, "Y"=1075.5057}, {"X"=316.67346, "Y"=1087.5939}, {"X"=313.84503, "Y"=1078.4121}, {"X"=311.07977, "Y"=1093.5851}, {"X"=288.58124, "Y"=1084.1323}, {"X"=253.53436, "Y"=1089.6963}, {"X"=222.62537, "Y"=1089.2378}, {"X"=207.23555, "Y"=1092.049}, {"X"=198.88261, "Y"=1094.9614}, {"X"=201.84657, "Y"=1101.0656}, {"X"=219.81421, "Y"=1089.1962}, {"X"=246.61075, "Y"=1095.6655}, {"X"=276.09103, "Y"=1099.1295}, {"X"=277.37112, "Y"=1087.0094}, {"X"=269.01492, "Y"=1092.9628}, {"X"=259.4417, "Y"=1110.9661}, {"X"=236.27989, "Y"=1143.5557}, {"X"=221.25168, "Y"=1155.2086}, {"X"=211.40356, "Y"=1149.145}, {"X"=210.1577, "Y"=1155.0537}, {"X"=210.93672, "Y"=1187.3989}, {"X"=219.5268, "Y"=1202.0677}, {"X"=214.17035, "Y"=1207.7928}, {"X"=212.45312, "Y"=1193.2517}, {"X"=216.24544, "Y"=1178.6962}, {"X"=215.63718, "Y"=1152.1692}, {"X"=237.17642, "Y"=1116.662}, {"X"=241.8254, "Y"=1062.0085}, {"X"=222.80795, "Y"=1030.774}, {"X"=200.59508, "Y"=995.9229}, {"X"=181.7759, "Y"=989.29376}, {"X"=174.5002, "Y"=986.0065}, {"X"=181.31502, "Y"=973.3979}, {"X"=193.25972, "Y"=989.47906}, {"X"=225.07932, "Y"=1002.62335}, {"X"=250.86584, "Y"=1006.1818}, {"X"=262.49365, "Y"=1022.038}, {"X"=273.88068, "Y"=1022.2171}, {"X"=299.57214, "Y"=1038.1857}, {"X"=313.79227, "Y"=1056.9513}, {"X"=312.43094, "Y"=1075.3367}, {"X"=326.49393, "Y"=1078.6017}, {"X"=358.61533, "Y"=1106.384}, {"X"=377.8976, "Y"=1130.672}, {"X"=373.6136, "Y"=1142.5254}, {"X"=384.5492, "Y"=1154.5345}, {"X"=393.717, "Y"=1189.8738}, {"X"=422.6742, "Y"=1181.515}, {"X"=447.14792, "Y"=1190.5972}, {"X"=472.90427, "Y"=1242.7501}, {"X"=470.85092, "Y"=1265.3882}, {"X"=474.5339, "Y"=1276.6844}, {"X"=455.22995, "Y"=1245.3685}, {"X"=446.339, "Y"=1222.39}, {"X"=452.62378, "Y"=1190.6714}, {"X"=288.441, "Y"=1065.7874}, {"X"=285.5954, "Y"=1062.6736}, {"X"=287.03085, "Y"=1065.766}, {"X"=288.41754, "Y"=1062.7164}, {"X"=293.92096, "Y"=1041.1993}, {"X"=293.77948, "Y"=1019.40497}, {"X"=289.62396, "Y"=1034.9258}, {"X"=298.1369, "Y"=1035.0582}, {"X"=300.65625, "Y"=972.16364}, {"X"=301.81653, "Y"=914.15173}, {"X"=294.30423, "Y"=874.57556}, {"X"=295.6906, "Y"=861.3137}, {"X"=291.26135, "Y"=857.9021}, {"X"=285.22177, "Y"=837.7049}, {"X"=286.8513, "Y"=857.8232}, {"X"=289.72052, "Y"=847.8503}, {"X"=273.3088, "Y"=827.38306}, {"X"=266.3032, "Y"=860.78937}, {"X"=264.87308, "Y"=864.09326}, {"X"=265.07156, "Y"=880.6789}, {"X"=268.2624, "Y"=903.76855}, {"X"=270.08127, "Y"=936.3443}, {"X"=267.44833, "Y"=958.83356}, {"X"=269.1082, "Y"=978.01495}, {"X"=269.28876, "Y"=993.8678}, {"X"=270.8951, "Y"=1009.64264}, {"X"=273.94638, "Y"=1028.4579}, {"X"=275.62167, "Y"=1053.2856}, {"X"=275.62167, "Y"=1053.2856}, {"X"=263.0895, "Y"=1068.471}, {"X"=242.29764, "Y"=1089.5295}, {"X"=220.66837, "Y"=1128.421}, {"X"=207.16425, "Y"=1146.1168}, {"X"=202.84323, "Y"=1140.1073}, {"X"=191.70963, "Y"=1139.9497}, {"X"=194.81741, "Y"=1151.8776}, {"X"=208.25342, "Y"=1190.2806}, {"X"=207.67186, "Y"=1222.1378}, {"X"=207.74364, "Y"=1225.0144}, {"X"=206.30415, "Y"=1222.1199}, {"X"=216.71391, "Y"=1199.1267}, {"X"=232.80104, "Y"=1178.9222}, {"X"=266.76187, "Y"=1138.035}, {"X"=298.6011, "Y"=1117.5511}, {"X"=336.27682, "Y"=1103.038}, {"X"=362.87262, "Y"=1097.3806}, {"X"=375.4271, "Y"=1100.591}, {"X"=383.88205, "Y"=1094.6619}, {"X"=382.44803, "Y"=1097.6693}, {"X"=380.98148, "Y"=1103.6938}, {"X"=374.0598, "Y"=1097.5457}, {"X"=369.89243, "Y"=1094.455}, {"X"=365.7194, "Y"=1091.3601}, {"X"=361.563, "Y"=1085.2206}, {"X"=358.841, "Y"=1072.978}, {"X"=349.01392, "Y"=1069.7695}, {"X"=340.51578, "Y"=1087.9485}, {"X"=329.30637, "Y"=1075.5903}, {"X"=346.23813, "Y"=1060.5228}, {"X"=366.1975, "Y"=1033.011}, {"X"=373.52267, "Y"=1008.1356}, {"X"=386.91687, "Y"=960.81134}, {"X"=397.61856, "Y"=915.79474}, {"X"=428.98264, "Y"=870.3323}, {"X"=433.86023, "Y"=847.1037}, {"X"=433.86023, "Y"=847.1037}, {"X"=436.79663, "Y"=847.15674}, {"X"=437.0149, "Y"=837.1033}, {"X"=437.08783, "Y"=833.74335}, {"X"=434.1437, "Y"=833.68964}, {"X"=423.1352, "Y"=870.22845}, {"X"=423.1352, "Y"=870.22845}, {"X"=427.2566, "Y"=883.5304}, {"X"=425.47482, "Y"=899.9389}, {"X"=412.0573, "Y"=919.29694}, {"X"=404.51083, "Y"=938.60956}, {"X"=398.13446, "Y"=980.11847}, {"X"=392.2399, "Y"=992.6899}, {"X"=393.75403, "Y"=986.38873}, {"X"=386.4898, "Y"=995.7541}, {"X"=373.52267, "Y"=1008.1356}, {"X"=366.1975, "Y"=1033.011}, {"X"=367.53558, "Y"=1042.3387}, {"X"=382.90997, "Y"=1058.0071}, {"X"=392.31473, "Y"=1091.7546}, {"X"=390.7536, "Y"=1103.8373}, {"X"=393.29352, "Y"=1121.9199}, {"X"=398.40585, "Y"=1151.771}, {"X"=407.9761, "Y"=1157.8162}, {"X"=426.79135, "Y"=1181.5712}, {"X"=452.83017, "Y"=1233.9342}, {"X"=463.45508, "Y"=1287.7449}, {"X"=456.98663, "Y"=1279.2715}, {"X"=447.8751, "Y"=1267.9182}, {"X"=444.18976, "Y"=1253.7445}, {"X"=439.67667, "Y"=1216.5513}, {"X"=429.98172, "Y"=1161.0725}, {"X"=427.91507, "Y"=1128.4023}, {"X"=-459.3773, "Y"=-967.1659}] {"Y" format="%.2f"; "X" format="%.2f"}
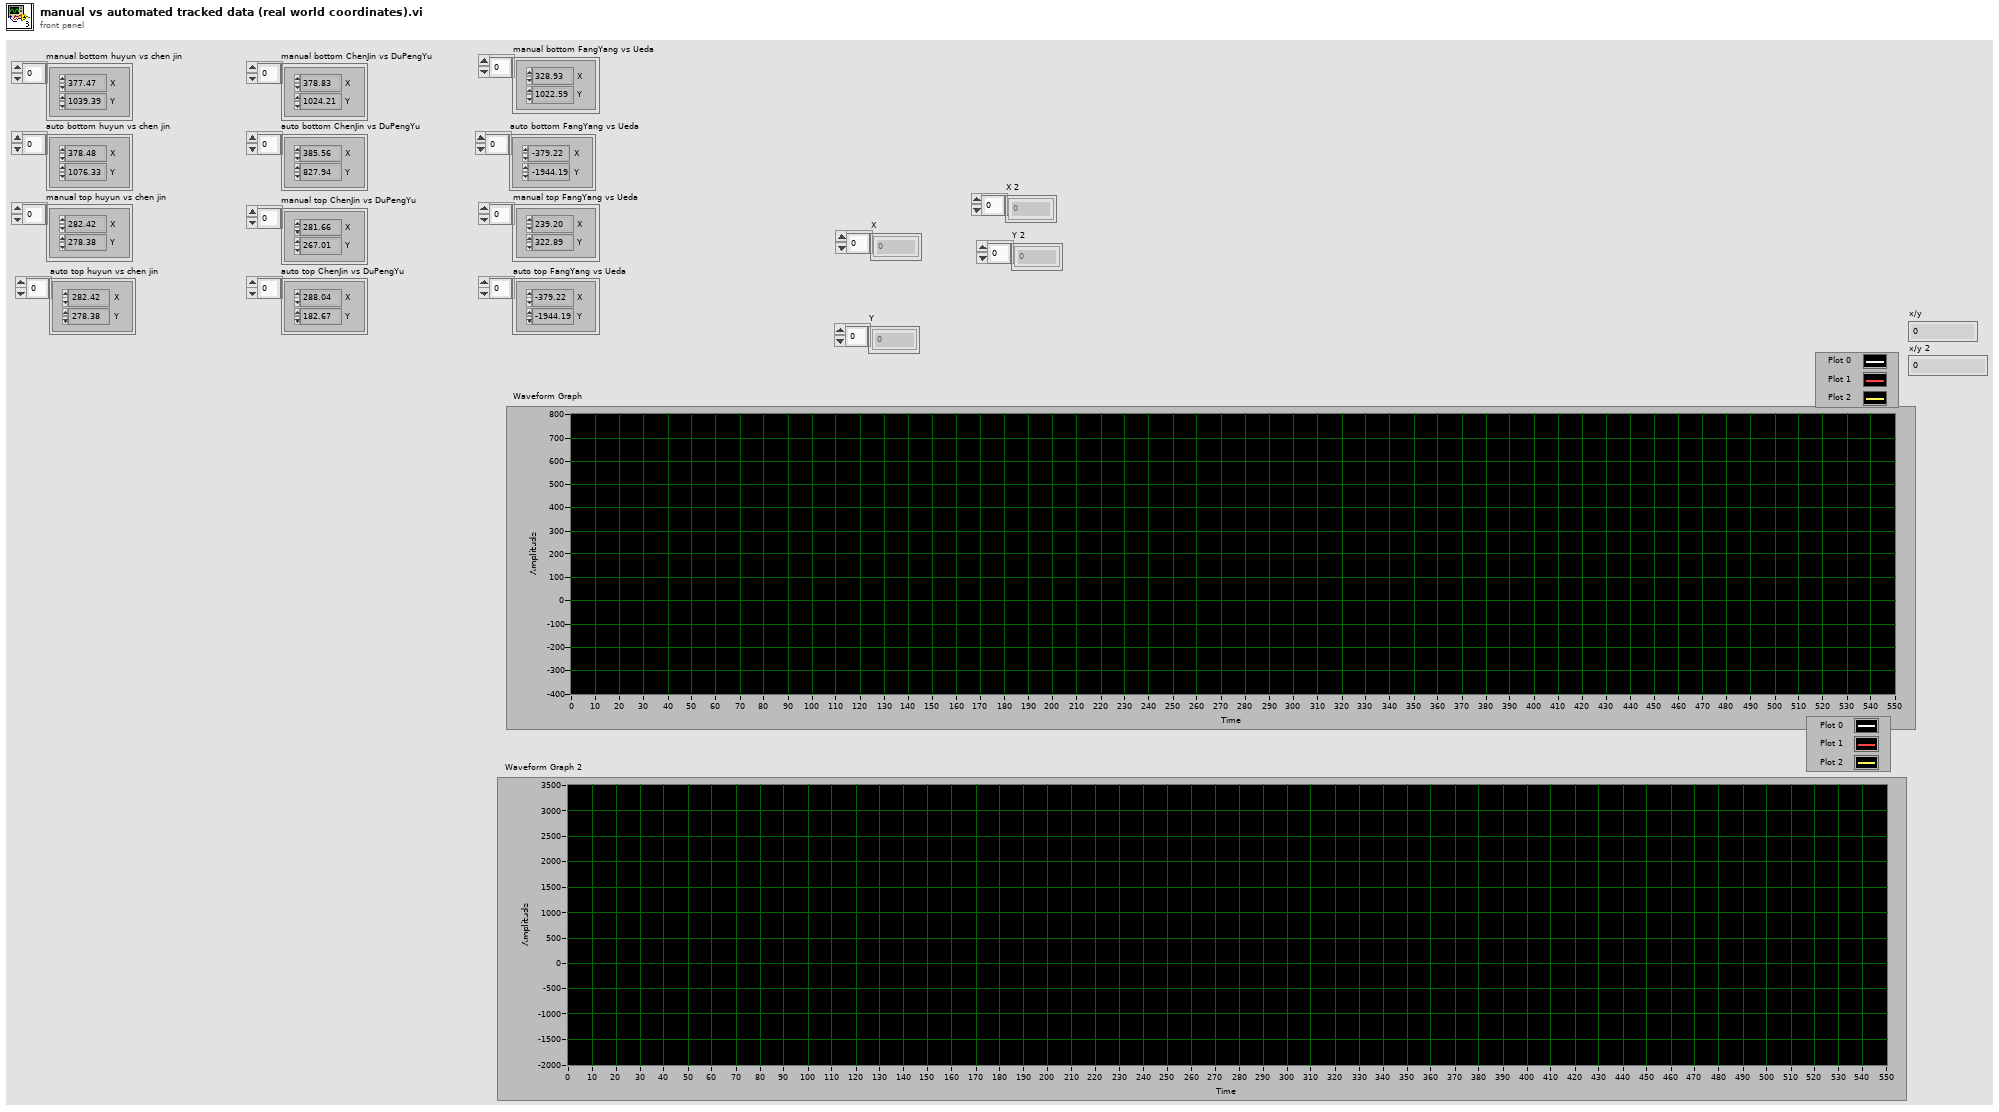
[diagram p1: front panel]
types:
  T1 = typedef "IMAQ Point" = cluster{"X":sgl, "Y":sgl}
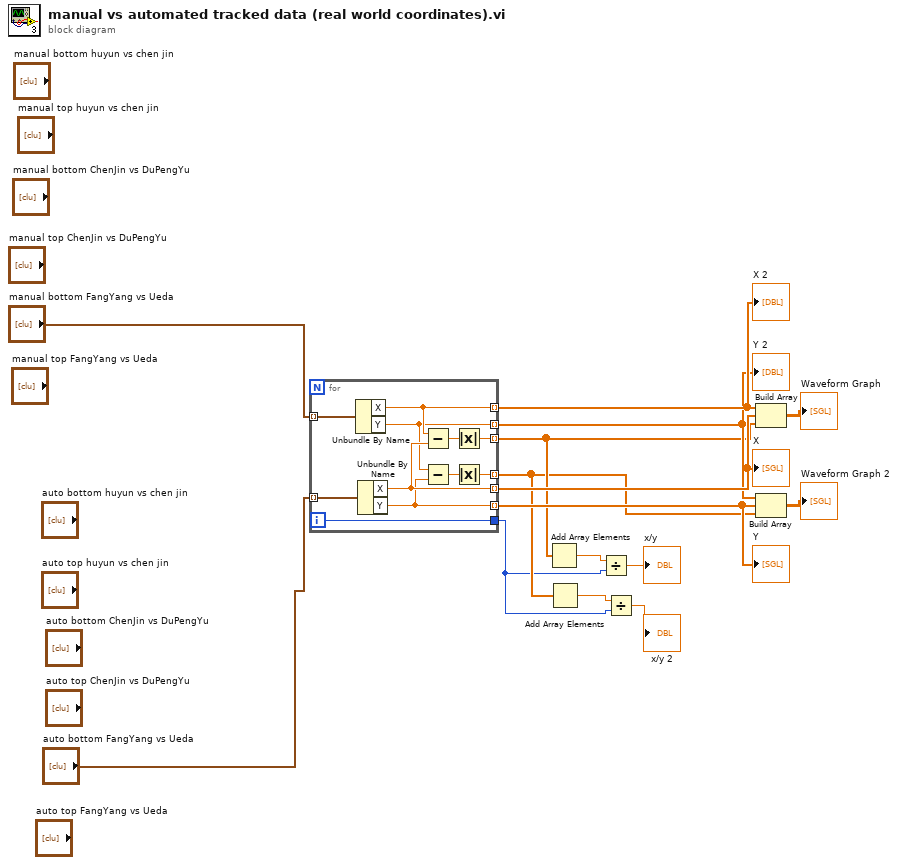
[diagram p0: block diagram]
diagram:
  n1 = for {
    tunnel: "manual bottom FangYang vs Ueda" -> [w26] mode=indexing
    tunnel: [w24] -> w15 mode=indexing
    tunnel: [w21] -> w12 mode=indexing
    tunnel: "auto bottom FangYang vs Ueda" -> [w25] mode=indexing
    tunnel: [w23] -> w13 mode=indexing
    tunnel: [w20] -> w11 mode=indexing
    tunnel: [w18] -> w9 mode=indexing
    tunnel: [w17] -> w8 mode=indexing
    tunnel: [w16] -> w5
    i -> [w16]
    n2 = Unbundle By Name(w26) -> ("X"=w24:sgl, "Y"=w21:sgl)
    n3 = Unbundle By Name(w25) -> ("X"=w23:sgl, "Y"=w20:sgl)
    n4 = Subtract(x=w24, y=w23) -> (x-y=w22:sgl)
    n5 = Subtract(x=w21, y=w20) -> (x-y=w19:sgl)
    n6 = Absolute Value(x=w22) -> (abs(x)=w18:sgl)
    n7 = Absolute Value(x=w19) -> (abs(x)=w17:sgl)
  }
  "X 2" <- w15
  "Y 2" <- w12
  "X" <- w13
  "Y" <- w11
  n8 = Add Array Elements(numeric array=w9) -> (sum=w7:sgl)
  n9 = Add Array Elements(numeric array=w8) -> (sum=w6:sgl)
  n10 = Divide(x=w7, y=w5) -> (x/y=→"x/y":sgl)
  n11 = Divide(x=w6, y=w5) -> (x/y=→"x/y 2":sgl)
  n12 = Build Array(w15, w13, w9) -> (→"Waveform Graph":sgl[][])
  n13 = Build Array(w12, w11, w8) -> (→"Waveform Graph 2":sgl[][])
